vi "Main_Marvin Remake.vi"() -> ()   [LabVIEW 2017]
uses:
  PCAN_Driver/ControlCAN.llb/DevType.ctl
  PCAN_Driver/ControlCAN.llb/CAN Channel.ctl
  PCAN_Driver/ControlCAN.llb/VCI_INIT_CONFIG.ctl
  PCAN_Driver/ControlCAN.llb/InitFlag.ctl
  PCAN_Driver/ControlCAN.llb/Fliter.ctl
  PCAN_Driver/ControlCAN.llb/Mode.ctl
  <vilib>/Utility/miscctls.llb/LVRowAndColumnTypeDef.ctl
  <vilib>/Utility/cursorutil.llb/Set Cursor (Icon Pict).vi
  PCAN_Driver/ControlCAN.lvlib
panel:
  out "AO[1]Meas":dbl
  out "FullSpeed2 Speed":dbl
  out "FullSpeed2 Current":u32
  out "FullSpeed1 Current":u32
  out "FullSpeed1 Speed":dbl
  out "MaxBurnInTempVal":dbl
  in  "Stop Burn-in":bool
  out "VISA Tester":refnum<visa-resource-name>
  out "UUT":u8
  out "CAN Status":bool
  in  "Channel 2":T1 caption="Channel" items=["Channel 1", "Channel 2"]
  out "Config_CANAT":T7 {"DevType" items=["USB-CAN"=3, "USB-CAN2"=4]; "CanIndex" items=["通道1", "通道2"]; "VCI_INIT_CONFIG"."Fliter" items=["接收所有类型"=3, "只接收标准帧"=4, "只接收扩展帧"=7]; "VCI_INIT_CONFIG"."Mode" items=["正常工作", "自测模式（环回）", "仅侦听模式"]; "VCI_INIT_CONFIG"."InitFlag" items=["使用Flash参数", "使用界面设置参数"]}
  out "Array":u64[][](array[numeric]) format="%016x"
  out "Motor Phase Current RMS":dbl
  out "Ambient Temperature":dbl
  out "Speed error":bool
  out "Commutation err":bool
  out "Under voltage/Over voltage":bool
  out "Derated drive temp":bool
  out "Motor Over temperature":bool
  out "Motor Sensor temp Fauilre":bool
  out "Drive Over temperature":bool
  out "Drive Sensor temp Failure":bool
  out "Ambient Over temp":bool
  out "Ambient Sensor temp":bool
  out "DC Voltage":dbl
  out "DC Current":dbl
  out "Power transistor Heat sink Temp.":dbl
  out "Motor Stator Temp.":dbl
  out "Motor Speed RPM":dbl
  out "ECS State":u16
  out "UUT":string="EBAY"
  in  "Logger Path":path
  in  "Report":bool
  in  "Start":bool
  in  "ATR":string[][](table)=[["Test Communication", "-", "-", "-", "-", ""], ["Set S/N", "-", "-", "-", "-", ""], ["Set Board Number", "-", "-", "-", "-", ""], [" ", "", "", "", "", ""], ["Test Communication", "-", "-", "-", "-", ""], ["Get S/N", "-", "-", "-", "", ""], ["Get Board Number", "-", "-", "-", "", ""], ["Get FW", "-", "-", "-", "", ""], ["Enable Motor", "", "", "", "", ""], ["Small position command", "", "", "", "", ""], ["Measure delta", "", "", "", "", ""], ["Velocity command", "", "", "", "", ""]]
  in  "Settings":bool
  in  "Refresh Button":bool
  out "Status":bool
  in  "VISA Marvin":refnum<visa-resource-name>="COM6"
  in  "Serial Com":bool
  in  "Help Button":bool
  out "Pannel User Message":string
  in  "Stop Button":bool
  # "Marvin"
  # "REDLER TECHNOLOGIES LTD"
  # "ver 1.0"
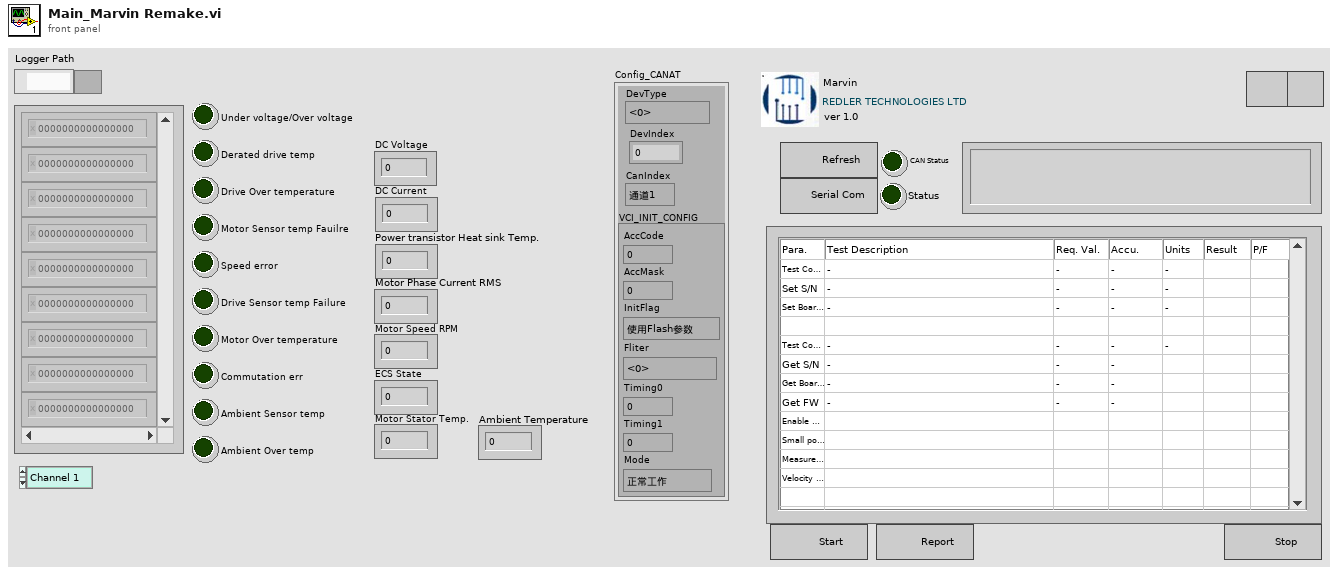
[diagram p1: front panel]
types:
  T1 = typedef "ControlCAN.lvlib/CAN Channel.ctl" = u32
  T2 = typedef "ControlCAN.lvlib/DevType.ctl" = u32
  T3 = typedef "ControlCAN.lvlib/VCI_INIT_CONFIG.ctl" = cluster{"AccCode":u32, "AccMask":u32, "InitFlag":T4, "Fliter":T5, "Timing0":u8, "Timing1":u8, "Mode":T6}
  T4 = typedef "ControlCAN.lvlib/InitFlag.ctl" = u32
  T5 = typedef "ControlCAN.lvlib/Fliter.ctl" = u8
  T6 = typedef "ControlCAN.lvlib/Mode.ctl" = u8
  T7 = cluster{"DevType":T2, "DevIndex":u32, "CanIndex":T1, "VCI_INIT_CONFIG":T3}
  T8 = cluster{"VISA":refnum<visa-resource-name>, "Array Test":enum16{"Auxiliary", "Temp Sens Cal", "Com Test", "Enable Test", "Speed Command", "Stop Time", "Temp Control", "Burn in", "Visual Inspec", "Empty"}[]}
  T9 = cluster{"ID":u32, "MSGTYPE":u8, "LEN":u8, "aDATA":u8[]}[]
  T10 = enum16{"Erase ATR Table", "Stop", "MainProgram", "Initialize"}
  T11 = enum16{"K15", "K16", "K17", "Venable", "Firmeware", "Fan", "Power", "120C", "110C", "100C", "90C", "80C", "70C", "60C", "50C", "40C", "30C", "25C", "20C", "10C", "0C"}
  T12 = enum16{"Stop", "Result", "FullSpeed2", "MD[1]=1", "FullSpeed1", "MD[1]=0"}
  T13 = enum8{"Term1", "Term2", "Current", "Fan", "TempCPU"}
  T14 = enum16{"Stop", "AO[1]=Meas.", "TA[5]", "AO[1]=0", "Start"}
  T15 = enum16{"Stop", "BurnIn", "Ambient Temp", "MotorSpeed", "DC Current Measure", "Start"}
  T16 = enum16{"Auxiliary", "Temp Sens Cal", "Com Test", "Enable Test", "Speed Command", "Stop Time", "Temp Control", "Burn in", "Visual Inspec", "Empty"}[]
  T17 = enum16{"K15", "K16", "K17", "Venable", "Firmeware", "Fan", "Power", "120C", "110C", "100C", "90C", "80C", "70C", "60C", "50C", "40C", "30C", "25C", "20C", "10C", "0C"}[]
  T18 = typedef "LVRowAndColumnTypeDef.ctl" = cluster{"Row":i32, "Column":i32}
  T19 = cluster{"ID":u32, "MSGTYPE":u8, "LEN":u8, "aDATA":u8[]}
  T20 = enum16{"Auxiliary", "Temp Sens Cal", "Com Test", "Enable Test", "Speed Command", "Stop Time", "Temp Control", "Burn in", "Visual Inspec", "Empty"}
  T21 = enum16{"open", "replace", "create", "open or create", "replace or create", "replace or create with confirmation"}
  T22 = enum32{"Invalid", "Standard", "Closed", "Hidden", "Minimized", "Maximized"}
  T23 = typedef "ControlCAN.lvlib/VCI_CAN_OBJ.ctl" = cluster{"ID":u32, "TimeStamp":u32, "TimeFlag":u8, "SendType":u8, "RemoteFlag":u8, "ExternFlag":u8, "DataLen":u8, "Data":u8[], "Reserved":u8[]}
  T24 = cluster{"Type":enum16{"接收", "发送"}, "Channel":T1, "Time":timestamp, "VCI_CAN_OBJ":T23}[]
  T25 = cluster{"Type":enum16{"接收", "发送"}, "Channel":T1, "Time":timestamp, "VCI_CAN_OBJ":T23}
  T26 = typedef "LVPoint32TypeDef.ctl" = cluster{"Horizontal":i32, "Vertical":i32}
  T27 = enum16{"Visual Inspection", "Temp Sens Cal", "Com Test", "Enable Test", "Speed Command", "Stop Time", "Temp Control", "Burn in", "Visual Inspec", "Empty"}[]
  T28 = enum16{"Auxiliary", "Temp Sens Cal", "Com Test", "Enable Test", "Speed Command", "Stop Time", "Burn in", "Visual Inspec", "Empty"}[]
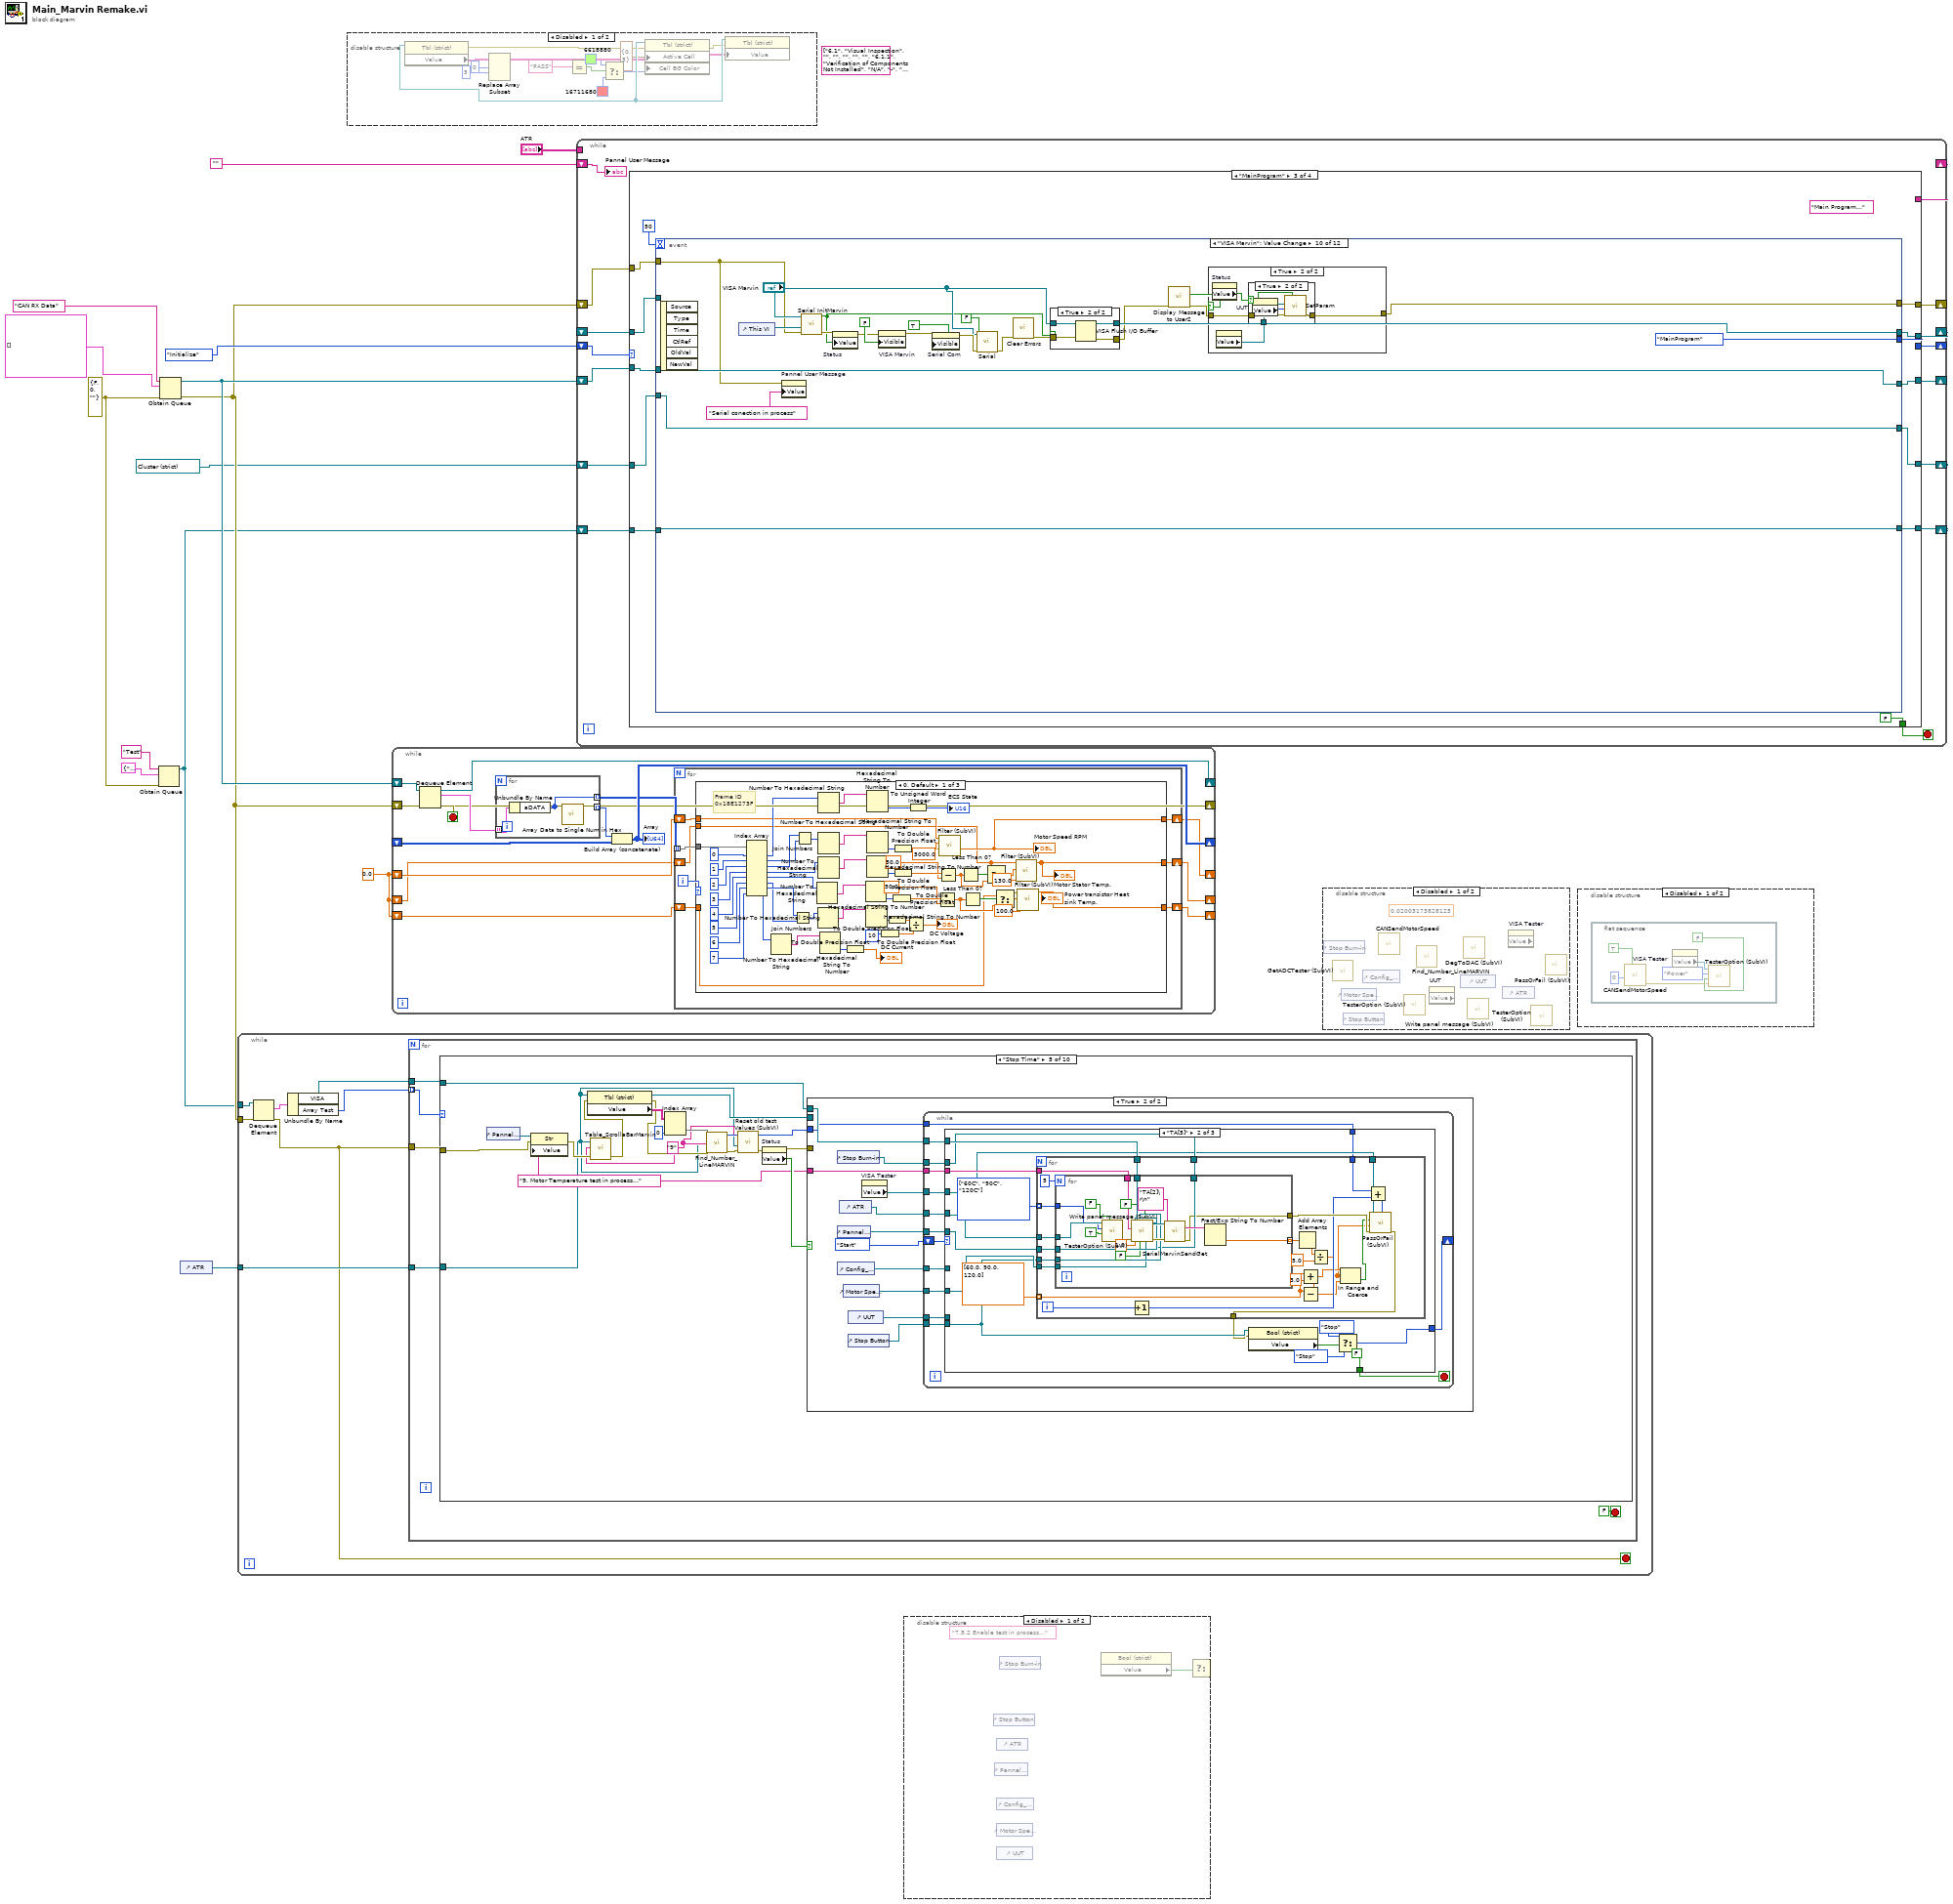
[diagram p0: block diagram]
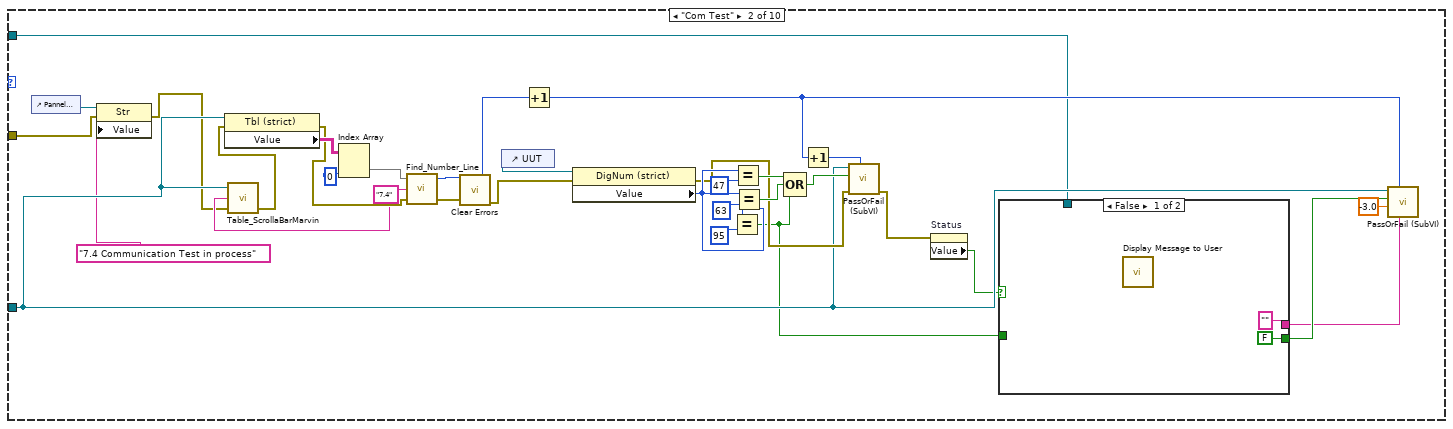
[diagram p6: hidden frame]
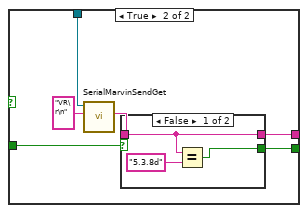
[diagram p7: hidden frame]
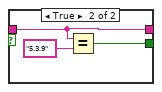
[diagram p8: hidden frame]
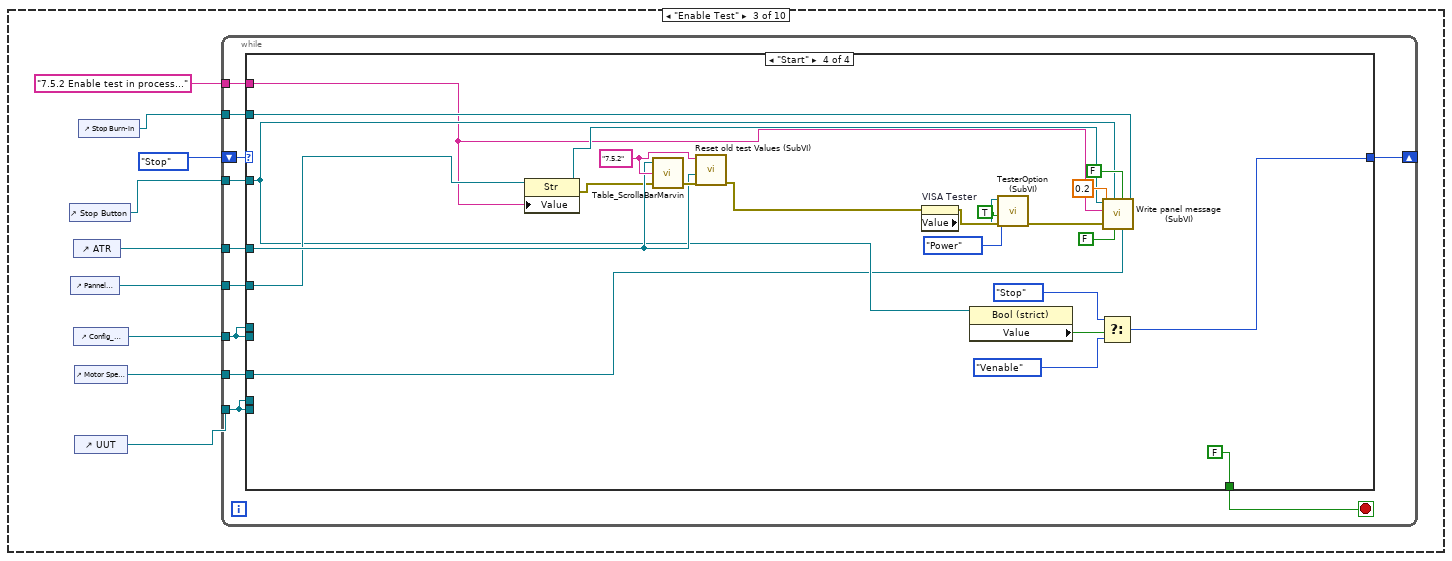
[diagram p9: hidden frame]
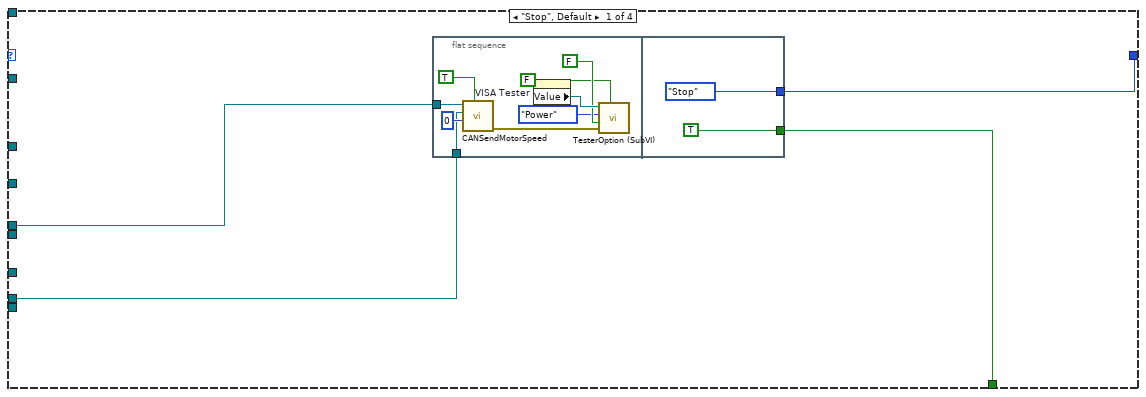
[diagram p10: hidden frame]
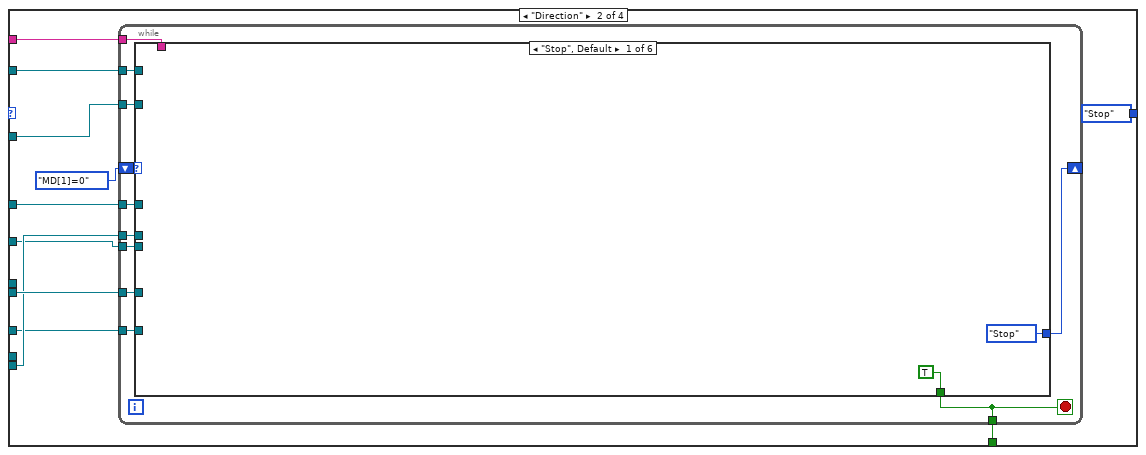
[diagram p11: hidden frame]
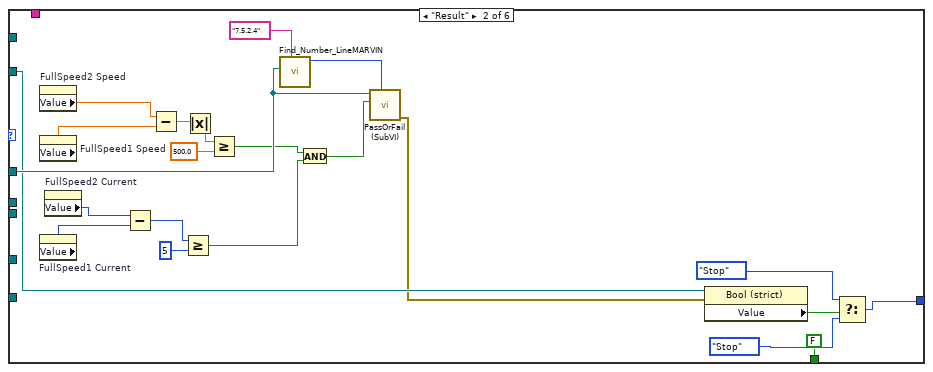
[diagram p12: hidden frame]
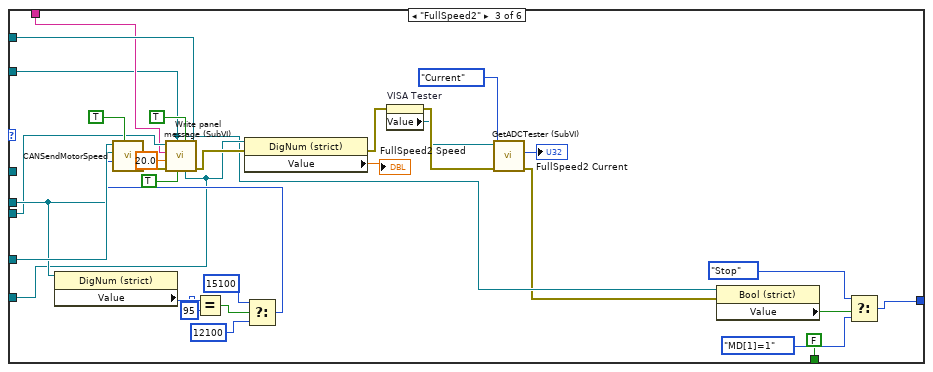
[diagram p13: hidden frame]
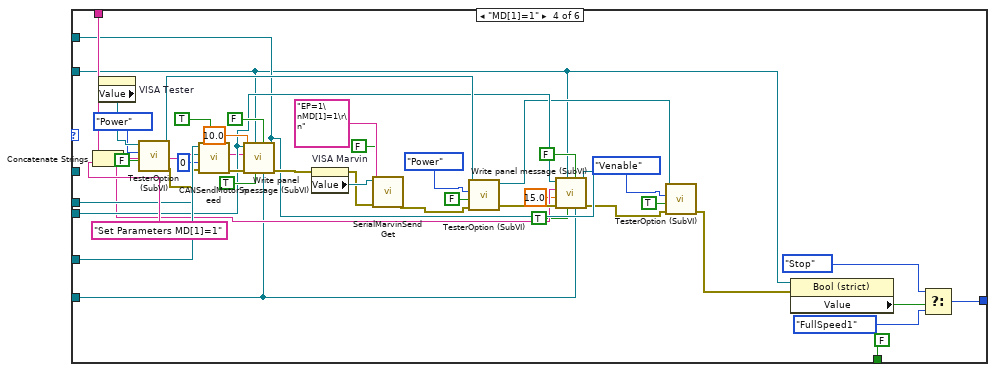
[diagram p14: hidden frame]
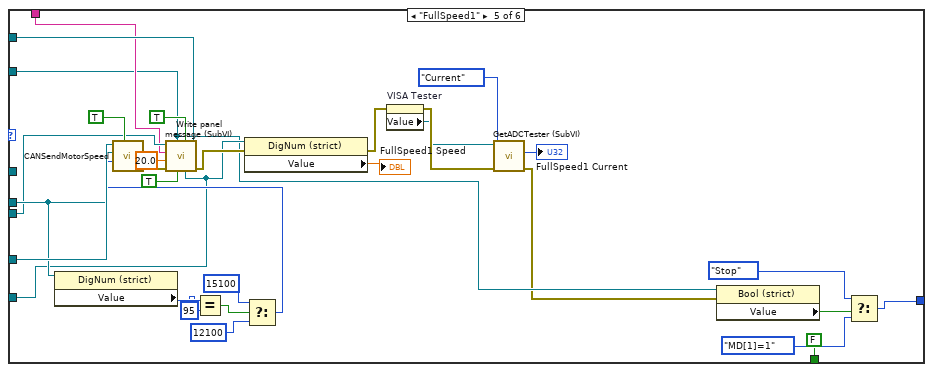
[diagram p15: hidden frame]
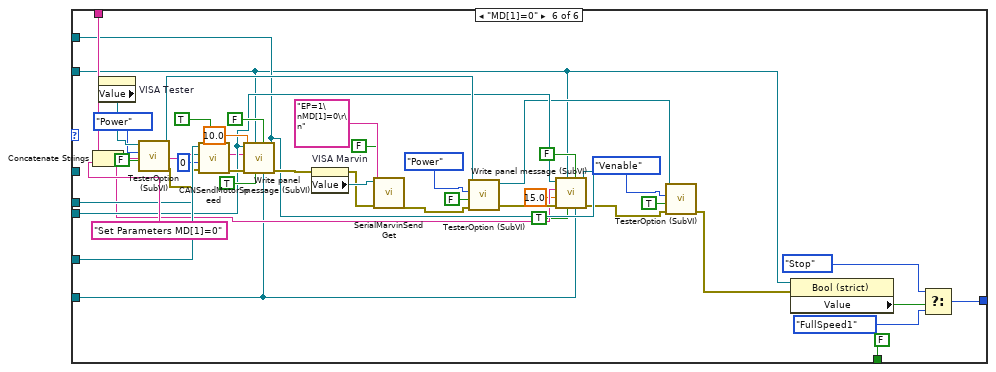
[diagram p16: hidden frame]
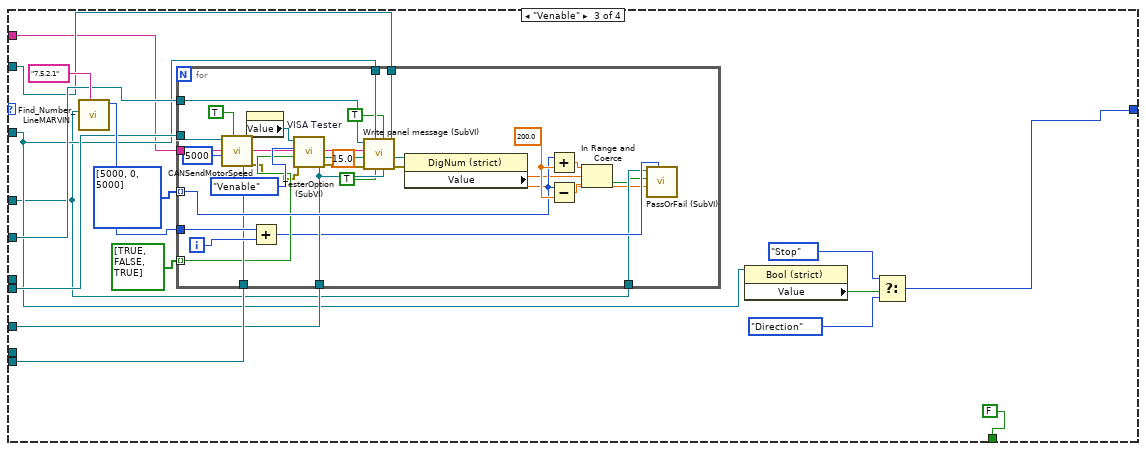
[diagram p17: hidden frame]
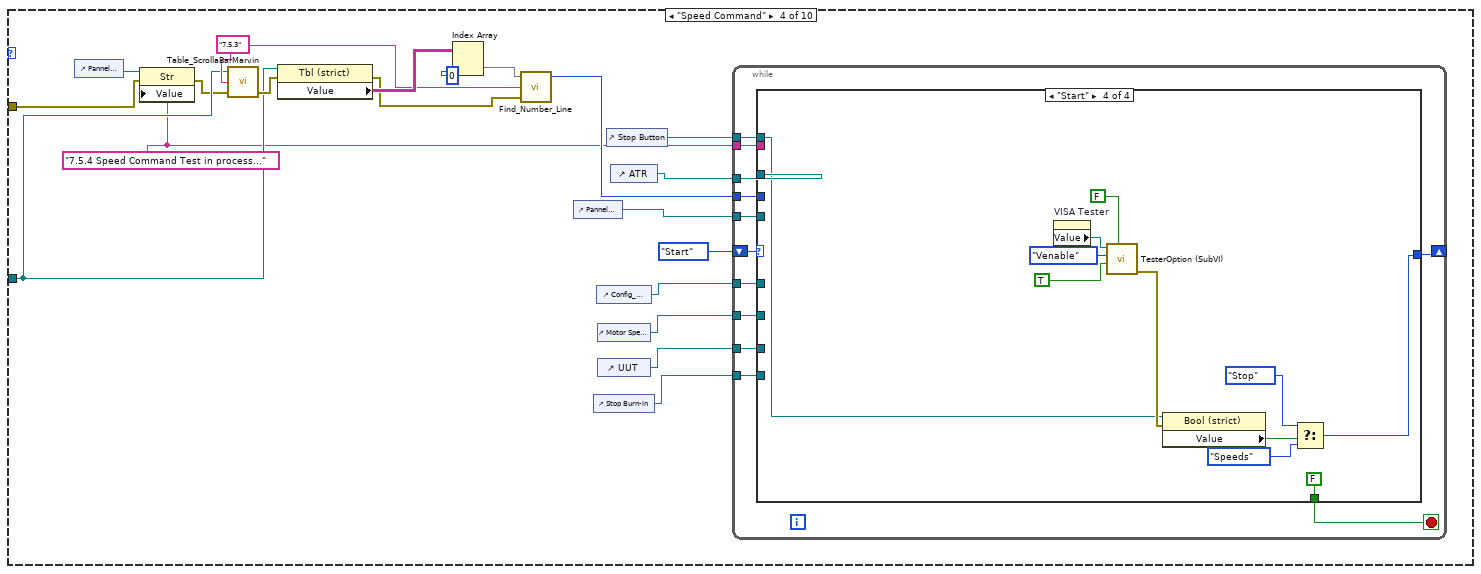
[diagram p18: hidden frame]
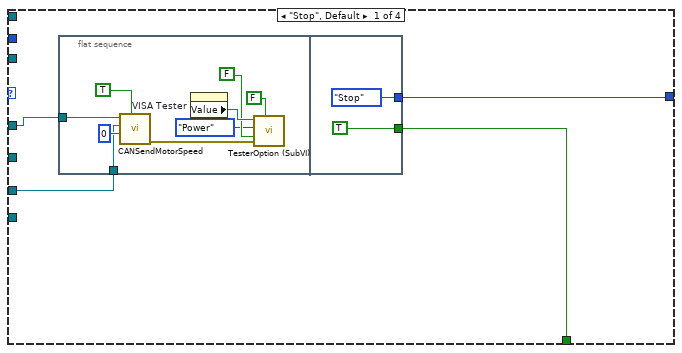
[diagram p19: hidden frame]
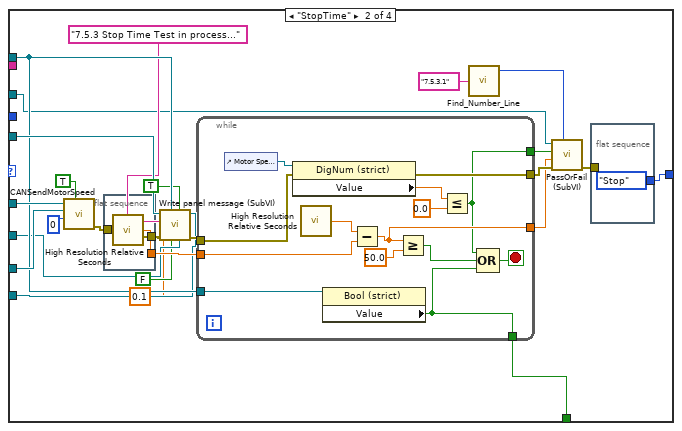
[diagram p20: hidden frame]
diagram:
  w1 = 0.0
  w8 = errorcluster {"status"=FALSE, "code"=0, "source"=""} ("error in (no error)")
  (unwired) string[][] [["6.1", "Visual Inspection", "", "", "", "", ""], ["6.1.1", "Verification of Components Not Installed", "N/A", "-", "", "", ""], ["", "", "", "", "", "", ""], ["6.1.2", "Manufacturing Defects", "N/A", "-", "", "", ""], ["", "", "", "", "", "", ""], ["6.2", "Power Supply Testing", "", "", "", "", ""], ["6.2.1", "Input Current Drawn", "", "", "", "", ""], ["6.2.1.1", "DC Input Current", "< 150", "-", "mA", "", ""], ["", "", "", "", "", "", ""], ["6.2.2", "Power Supply Voltages", "", "", "", "", ""], ["6.2.2.1", "12V", "12.0", "+/-0.500", "V", "", ""], ["6.2.2.2", "5V", "5.0", "+/-0.200", "V", "", ""], ["6.2.2.3", "3.3V", "3.3", "+/-0.100", "V", "", ""], ["6.2.2.4", "1.8V", "1.8", "+/-0.100", "V", "", ""], ["", "", "", "", "", "", ""], ["7", "Functional Test Procedure", "", "", "", "", ""], ["7.1", "Weight Check", "4180", "+/-10.00", "gr", "", ""], ["", "", "", "", "", "", ""], ["7.2", "Insulation Resistance Test", "", "", "", "", ""], ["7.2.1", "J3.B to Chassis", "> 1M", "-", "ohms", "", ""], ["7.2.2", "J1.16 to Chassis", "> 100K", "-", "ohms", "", ""], ["", "", "", "", "", "", ""], ["7.2", "Bonding Resistance", "", "", "", "", ""], ["7.2.3", "J1 Body to Chassis", "< 2m", "-", "ohms", "", ""], ["7.2.4", "J2  Body to Chassis", "< 2m", "-", "ohms", "", ""], ["7.2.5", "J3  Body to Chassis", "< 2m", "-", "ohms", "", ""], ["", "", "", "", "", "", ""], ["7.2.1", "CANbus Resistance Test", "", "", "", "", ""], ["7.2.1.1", "J1.17 to J1.18", "> 10K", "-", "ohms", "", ""], ["", "", "", "", "", "", ""], ["7.3", "Sealing Test", "N/A", "-", "", "", ""], ["", "", "", "", "", "", ""], ["7.4", "Communication Test", "", "", "", "", ""], ["7.4.1", "Serial RS-232", "N/A", "-", "", "", ""], ["7.4.2", "CAN Bus", "N/A", "-", "", "", ""], ["", "", "", "", "", "", ""], ["7.5", "Performances Tests", "", "", "", "", ""], ["7.5.1", "Reverse Polarity Test", "", "", "", "", ""], ["7.5.1.1", "DC Input Current", "< 1", "-", "mA", "", ""], ["", "", "", "", "", "", ""], ["7.5.2", "Enable Test", "", "", "", "", ""], ["7.5.2.1", "Fan Speed at Opened Enable ", "0", "-", "rpm", "", ""], ["7.5.2.2", "Fan Speed at Closed Enable ", "6000", "+/-200.0", "rpm", "", ""], ["7.5.2.3", "Motor Rotation Direction", "Counter-clockwise (Inlet)", "-", "", "", ""], ["", "", "", "", "", "", ""], ["7.5.3", "Stop Time Test ", "", "", "", "", ""], ["7.5.3.1", "Motor Stop time", "< 50", "-", "sec", "", ""], ["", "", "", "", "", "", ""], ["7.5.4", "Speed Command Test", "", "", "", "", ""], ["7.5.4.1", "Fan Speed", "6000", "+/-200.0", "rpm", "", ""], ["7.5.4.2", "Fan Speed", "11500", "+/-200.0", "rpm", "", ""], ["7.5.4.3", "Fan Speed", "15100", "+/-200.0", "rpm", "", ""], ["", "", "", "", "", "", ""], ["7.5.5", "Temperature Sensor Calibration Test", "", "", "", "", ""], ["7.5.5.1", "Sensor Reading Analog Offset", "0", "+/-0.100", ".", "", ""], ["", "", "", "", "", "", ""], ["7.5.6", "Temperature Control Algorithm Test", "", "", "", "", ""], ["7.5.6.1", "Tair <   68 ± 2 oC", "6000", "+/-200.0", "rpm", "", ""], ["7.5.6.2", "Tair >= 68 ± 2 oC", "11500", "+/-200.0", "rpm", "", ""], ["7.5.6.3", "Tair >= 88 ± 2 oC", "15100", "+/-400.0", "rpm", "", ""], ["7.5.6.4", "Tair <= 80 ± 2 oC", "11500", "+/-200.0", "rpm", "", ""], ["7.5.6.5", "Tair <= 60 ± 2 oC", "6000", "+/-200.0", "rpm", "", ""], ["", "", "", "", "", "", ""], ["7.5.7", "Burn-in Test", "", "", "", "", ""], ["7.5.7.1", "DC Input Current", "50", "+/-5.000", "A", "", ""], ["7.5.7.2", "Ambient Temperature", "25", "+/-13.00", "Deg.", "", ""], ["7.5.7.3", "After 10 min of operation", "", "", "Deg.", "", ""], ["7.5.7.4", "After 20 min of operation", "", "", "Deg.", "", ""], ["7.5.7.5", "After 30 min of operation", "", "", "Deg.", "", ""], ["7.5.7.6", "Auxiliary Cooling Fan 60 Deg", "On", "-", ".", "", ""], ["7.5.7.7", "Auxiliary Cooling Fan 55 Deg", "Off", "-", ".", "", ""]] ("data")
  n1 = Obtain Queue(name (unnamed)="Test", element data type=T8 {"VISA"="COM1", "Array Test"=[]}, error in (no error)=w8) -> (queue out=w5:refnum<queue>)  [unwired: 2 in, 2 out]
  n2 = Obtain Queue(name (unnamed)="CAN RX Data", element data type=T9 [], error in (no error)=w8) -> (queue out=w10:refnum<queue>, error out=w6:errorcluster)  [unwired: 2 in, 1 out]
  n3 = control-ref of="ATR"() -> (w7:refnum<vi>)
  n4 = while {
    tunnel: w7 -> [w21]
    tunnel: w6 -> [w19]
    tunnel: w5 -> [w20]
    stop <- w15 stop-if-true
    n5 = Dequeue Element(queue=w20, error in (no error)=w19) -> (element=w18:T8, error out=w15:errorcluster)  [unwired: 1 in, 2 out]
    n6 = Unbundle By Name(w18) -> ("VISA"=w17:refnum<visa-resource-name>, "Array Test"=w16:T16)
    n7 = for {
      tunnel: w16 -> [w22] mode=indexing
      tunnel: w17 -> [w26]
      tunnel: w21 -> [w25]
      tunnel: w15 -> [w24]
      stop <- FALSE stop-if-true
      n8 = case shown="\"Stop Time\"" w22 {
        tunnel: w26 -> [_ w33 _ _ w514 _ _ _ w1006 _]
        tunnel: w25 -> [_ w41 _ w382 w510 w672 _ w1003 w1014 w1226]
        tunnel: w24 -> [_ w37 _ w380 w520 w668 _ w1004 w1012 w1225]
        frame "Empty", Default {
        }
        frame "Com Test" {
          w40 = "7.4" ("Test Paragraph")
          n9 = control-ref of="Pannel User Message"() -> (w38:refnum<vi>)
          n10 = property class="Str"(reference=w38, error in=w37, "Value"="7.4 Communication Test in process") -> (error out=w36:errorcluster)  [unwired: 1 out]
          n11 = call "Table_ScrollaBarMarvin.vi"("error in"=w36, "Line to focus"=w40, "reference in"=w41) -> ("error out"=w39:errorcluster)  [unwired: 2 out]
          n12 = property class="Tbl (strict)"(reference=w41, error in=w39) -> (error out=w56:errorcluster, "Value"=w57:string[][])  [unwired: 1 out]
          n13 = Index Array(array=w57, index (col)=0 ("disabled index (col)")) -> (element=w58:string[])  [unwired: 1 in]
          n14 = call "Find_Number_Line.vi"("error in"=w56, "Test Paragraph"=w40, "Row Headers[]"=w58) -> ("error out"=w54:errorcluster, "Line number"=w53:i32)  [unwired: 1 out]
          n15 = call <vilib>:"Clear Errors.vi"("error in (no error)"=w54) -> ("error out"=w32:errorcluster)  [unwired: 5 in, 1 out]
          n16 = control-ref of="UUT"() -> (w52:refnum<vi>)
          n17 = Increment(x=w53) -> (x+1=w45:i32)
          n18 = property class="DigNum (strict)"(reference=w52, error in=w32) -> (error out=w42:errorcluster, "Value"=w51:u8)  [unwired: 1 out]
          n19 = Equal?(x=w51, y=u8 95) -> (x = y?=w30:bool)
          n20 = Equal?(x=w51, y=u8 47) -> (x = y?=w47:bool)
          n21 = Equal?(x=w51, y=u8 63) -> (x = y?=w46:bool)
          n22 = Compound Arithmetic op=OR(w47, w46, w30) -> (w43:bool)
          n23 = Increment(x=w45) -> (x+1=w44:i32)
          n24 = call "PassOrFail (SubVI).vi"("index (row)"=w44, "error in (no error)"=w42, "Pass?Fail"=w43, "Table in"=w41) -> ("error out"=w31:errorcluster)  [unwired: 7 in]
          n25 = property on="Status" class="Bool (strict)"(error in=w31) -> ("Value"=w34:bool)  [unwired: 1 in, 2 out]
          n26 = case shown="False" w34 {
            tunnel: w33 -> [_ w66]
            tunnel: w30 -> [_ w64]
            tunnel: [FALSE w62] -> w29
            tunnel: ["" ("read buffer") w61] -> w28
            frame False {
              n27 = call "Display Message to User"() -> ()  [unwired: 10 in, 2 out]
            }
            frame True {
              n28 = call "SerialMarvinSendGet.vi"("write buffer"="VR\r\n", "VISA resource name"=w66) -> ("read buffer"=w63:string)  [unwired: 8 in, 1 out]
              n29 = case shown="False" w64 {
                tunnel: w63 -> [w67 w70]
                tunnel: [w68 w71] -> w62
                tunnel: [w67 w70] -> w61
                frame False {
                  n30 = Equal?(x=w67, y="5.3.8d") -> (x = y?=w68:bool)
                }
                frame True {
                  n31 = Equal?(x=w70, y="5.3.9") -> (x = y?=w71:bool)
                }
              }
            }
          }
          n32 = call "PassOrFail (SubVI).vi"("String Res"=w28, "index (row)"=w45, "Data in"=-3.0, "Pass?Fail"=w29, "Table in"=w41) -> ()  [unwired: 6 in, 1 out]
        }
        frame "Enable Test" {
          n33 = control-ref of="Stop Button"() -> (w75:refnum<vi>)
          n34 = control-ref of="Pannel User Message"() -> (w77:refnum<vi>)
          n35 = control-ref of="ATR"() -> (w76:refnum<vi>)
          n36 = control-ref of="Config_CANAT"() -> (w78:refnum<vi>)
          n37 = control-ref of="Motor Speed RPM"() -> (w79:refnum<vi>)
          n38 = control-ref of="UUT"() -> (w80:refnum<vi>)
          n39 = control-ref of="Stop Burn-in"() -> (w81:refnum<vi>)
          n40 = while {
            shift-right: [w86] -> _
            shift-left: enum16{"Stop", "Direction", "Venable", "Start"}."Stop" -> [w92]
            tunnel: w75 -> [w91]
            tunnel: w76 -> [w90]
            tunnel: w77 -> [w89]
            tunnel: w78 -> [w82]
            tunnel: w79 -> [w88]
            tunnel: w80 -> [w83]
            tunnel: w81 -> [w85]
            tunnel: "7.5.2 Enable test in process..." ("Strin") -> [w84]
            stop <- w87 stop-if-true
            n41 = case shown="\"Start\"" w92 {
              tunnel: w91 -> [_ w114 w303 w348]
              tunnel: w90 -> [_ w109 w301 w355]
              tunnel: w89 -> [_ w112 w305 w354]
              tunnel: w82 -> [_ w116 w308 _]
              tunnel: w88 -> [_ w111 w306 w346]
              tunnel: w83 -> [_ w115 w307 _]
              tunnel: [w96 w117 FALSE FALSE] -> w87
              tunnel: [w93 enum16{"Stop", "Direction", "Venable", "Start"}."Stop" w302 w352] -> w86
              tunnel: w85 -> [_ w113 w304 w347]
              tunnel: w84 -> [_ w110 w300 w345]
              tunnel: w83 -> [w95 _ _ _]
              tunnel: w82 -> [w94 _ _ _]
              frame "Stop", Default {
                n42 = flat-sequence {
                  tunnel: w95 -> [w101]
                  tunnel: w94 -> [w100]
                  tunnel: [TRUE] -> w96
                  tunnel: [enum16{"Stop", "Direction", "Venable", "Start"}."Stop"] -> w93
                  frame #0 {
                    n43 = call "CANSendMotorSpeed.vi"("Remote"=TRUE, "Motor Speed RPM"=u16 0, "UUT"=w101, "CAN Cluster in"=w100) -> ("error out"=w104:errorcluster)  [unwired: 7 in]
                    n44 = property on="VISA Tester" class="VISAName"() -> ("Value"=w105:refnum<visa-resource-name>)  [unwired: 2 in, 2 out]
                    n45 = call "TesterOption (SubVI).vi"("2 Options"=FALSE, "error in (no error)"=w104, "On/Off"=FALSE, "Tester Option"=T11."Power", "VISA Refnum in"=w105) -> ()  [unwired: 5 in, 2 out]
                  }
                  frame #1 {
                  }
                }
              }
              frame "Direction" {
                n46 = while {
                  shift-right: [w128] -> _
                  shift-left: T12."MD[1]=0" -> [w129]
                  tunnel: [w127] -> w117
                  tunnel: w116 -> [w126]
                  tunnel: w115 -> [w125]
                  tunnel: w114 -> [w124]
                  tunnel: w113 -> [w123]
                  tunnel: w112 -> [w122]
                  tunnel: w111 -> [w121]
                  tunnel: w110 -> [w120]
                  tunnel: w109 -> [w119]
                  stop <- w127 stop-if-true
                  n47 = case shown="\"Stop\", Default" w129 {
                    tunnel: [T12."Stop" w150 w181 w225 w254 w298] -> w128
                    tunnel: [TRUE FALSE FALSE FALSE FALSE FALSE] -> w127
                    tunnel: w126 -> [_ _ w179 w218 w252 w291]
                    tunnel: w125 -> [_ _ w173 w196 w246 w269]
                    tunnel: w124 -> [_ w133 w155 w186 w228 w259]
                    tunnel: w123 -> [_ _ w167 w197 w240 w270]
                    tunnel: w122 -> [_ _ w168 w198 w241 w271]
                    tunnel: w121 -> [_ _ w165 w192 w238 w265]
                    tunnel: w120 -> [_ _ w162 w206 w235 w279]
                    tunnel: w119 -> [_ w138 _ _ _ _]
                    frame "Stop", Default {
                    }
                    frame "Result" {
                      n48 = property on="FullSpeed2 Speed" class="DigNum (strict)"() -> ("Value"=w147:dbl)  [unwired: 2 in, 2 out]
                      n49 = property on="FullSpeed1 Speed" class="DigNum (strict)"() -> ("Value"=w146:dbl)  [unwired: 2 in, 2 out]
                      n50 = property on="FullSpeed1 Current" class="DigNum (strict)"() -> ("Value"=w143:u32)  [unwired: 2 in, 2 out]
                      n51 = property on="FullSpeed2 Current" class="DigNum (strict)"() -> ("Value"=w144:u32)  [unwired: 2 in, 2 out]
                      n52 = Subtract(x=w144, y=w143) -> (x-y=w142:u32)
                      n53 = Subtract(x=w147, y=w146) -> (x-y=w148:dbl)
                      n54 = Greater Or Equal?(x=w142, y=u32 5) -> (x >= y?=w136:bool)
                      n55 = Absolute Value(x=w148) -> (abs(x)=w145:dbl)
                      n56 = Greater Or Equal?(x=w145, y=500.0) -> (x >= y?=w137:bool)
                      n57 = call "Find_Number_LineMARVIN.vi"("Test Paragraph"="7.5.2.4", "TableIn"=w138) -> ("Line number"=w134:i32)  [unwired: 3 in, 3 out]
                      n58 = And(x=w137, y=w136) -> (x .and. y?=w135:bool)
                      n59 = call "PassOrFail (SubVI).vi"("index (row)"=w134, "Pass?Fail"=w135, "Table in"=w138) -> ("error out"=w132:errorcluster)  [unwired: 8 in]
                      n60 = property class="Bool (strict)"(reference=w133, error in=w132) -> ("Value"=w153:bool)  [unwired: 2 out]
                      n61 = Select(t=T12."Stop", s=w153, f=T12."Stop") -> (s? t:f=w150:T12)
                    }
                    frame "FullSpeed2" {
                      n62 = property class="DigNum (strict)"(reference=w173) -> ("Value"=w178:u8)  [unwired: 1 in, 2 out]
                      n63 = Equal?(x=w178, y=u8 95) -> (x = y?=w177:bool)
                      n64 = Select(t=u16 15100, s=w177, f=u16 12100 ("y")) -> (s? t:f=w172:u16)
                      n65 = call "CANSendMotorSpeed.vi"("Remote"=TRUE, "Motor Speed RPM"=w172, "UUT"=w173, "CAN Cluster in"=w179) -> ("error out"=w170:errorcluster)  [unwired: 7 in]
                      n66 = call "Write panel message (SubVI).vi"("Stop BurnIn"=w167, 4:"rpm"=w165, 5:"rpm"=TRUE ("rpm"), "PrintTime"=TRUE, "Stop"=w155, "error in (no error)"=w170, "Time to wait"=20.0, "Strin"=w162, "String in"=w168) -> ("error out"=w169:errorcluster)  [unwired: 2 in]
                      n67 = property class="DigNum (strict)"(reference=w165, error in=w169) -> (error out=w161:errorcluster, "Value"=→"FullSpeed2 Speed":dbl)  [unwired: 1 out]
                      n68 = property on="VISA Tester" class="VISAName"(error in=w161) -> (error out=w160:errorcluster, "Value"=w159:refnum<visa-resource-name>)  [unwired: 1 in, 1 out]
                      n69 = call "GetADCTester (SubVI).vi"("error in (no error)"=w160, "GetADCTester"=T13."Current", "VISA Refnum in"=w159) -> ("error out"=w154:errorcluster, "ADCValOutput Single"=→"FullSpeed2 Current":u32)  [unwired: 6 in, 1 out]
                      n70 = property class="Bool (strict)"(reference=w155, error in=w154) -> ("Value"=w184:bool)  [unwired: 2 out]
                      n71 = Select(t=T12."Stop", s=w184, f=T12."MD[1]=1") -> (s? t:f=w181:T12)
                    }
                    frame "MD[1]=1" {
                      n72 = Concatenate Strings(w206, "Set Parameters MD[1]=1" ("Strin")) -> (w195:string)
                      n73 = property on="VISA Tester" class="VISAName"() -> ("Value"=w212:refnum<visa-resource-name>)  [unwired: 2 in, 2 out]
                      n74 = call "TesterOption (SubVI).vi"("On/Off"=FALSE, "Tester Option"=T11."Power", "VISA Refnum in"=w212) -> ("error out"=w213:errorcluster, "VISA Refnum out"=w202:refnum<visa-resource-name>)  [unwired: 7 in]
                      n75 = call "CANSendMotorSpeed.vi"("Remote"=TRUE, "error in (no error)"=w213, "Motor Speed RPM"=u16 0, "UUT"=w196, "CAN Cluster in"=w218) -> ("error out"=w215:errorcluster)  [unwired: 6 in]
                      n76 = call "Write panel message (SubVI).vi"("Stop BurnIn"=w197, 4:"rpm"=w192, 5:"rpm"=FALSE ("rpm"), "PrintTime"=TRUE, "Stop"=w186, "error in (no error)"=w215, "Time to wait"=10.0, "Strin"=w195, "String in"=w198) -> ("error out"=w209:errorcluster)  [unwired: 2 in]
                      n77 = property on="VISA Marvin" class="VISAName"(error in=w209) -> (error out=w214:errorcluster, "Value"=w221:refnum<visa-resource-name>)  [unwired: 1 in, 1 out]
                      n78 = call "SerialMarvinSendGet.vi"("error in (no error)"=w214, "Clear Log"=FALSE, "write buffer"="EP=1\nMD[1]=1\r\n", "VISA resource name"=w221) -> ("error out"=w201:errorcluster)  [unwired: 6 in, 1 out]
                      n79 = call "TesterOption (SubVI).vi"("error in (no error)"=w201, "On/Off"=FALSE, "Tester Option"=T11."Power", "VISA Refnum in"=w202) -> ("error out"=w199:errorcluster, "VISA Refnum out"=w187:refnum<visa-resource-name>)  [unwired: 6 in]
                      n80 = call "Write panel message (SubVI).vi"("Stop BurnIn"=w197, 4:"rpm"=w192, 5:"rpm"=FALSE ("rpm"), "PrintTime"=TRUE, "Stop"=w186, "error in (no error)"=w199, "Time to wait"=15.0, "Strin"=w195, "String in"=w198) -> ("error out"=w188:errorcluster)  [unwired: 2 in]
                      n81 = call "TesterOption (SubVI).vi"("error in (no error)"=w188, "On/Off"=TRUE, "Tester Option"=T11."Venable", "VISA Refnum in"=w187) -> ("error out"=w185:errorcluster)  [unwired: 6 in, 1 out]
                      n82 = property class="Bool (strict)"(reference=w186, error in=w185) -> ("Value"=w226:bool)  [unwired: 2 out]
                      n83 = Select(t=T12."Stop", s=w226, f=T12."FullSpeed1") -> (s? t:f=w225:T12)
                    }
                    frame "FullSpeed1" {
                      n84 = property class="DigNum (strict)"(reference=w246) -> ("Value"=w251:u8)  [unwired: 1 in, 2 out]
                      n85 = Equal?(x=w251, y=u8 95) -> (x = y?=w250:bool)
                      n86 = Select(t=u16 15100, s=w250, f=u16 12100 ("y")) -> (s? t:f=w245:u16)
                      n87 = call "CANSendMotorSpeed.vi"("Remote"=TRUE, "Motor Speed RPM"=w245, "UUT"=w246, "CAN Cluster in"=w252) -> ("error out"=w243:errorcluster)  [unwired: 7 in]
                      n88 = call "Write panel message (SubVI).vi"("Stop BurnIn"=w240, 4:"rpm"=w238, 5:"rpm"=TRUE ("rpm"), "PrintTime"=TRUE, "Stop"=w228, "error in (no error)"=w243, "Time to wait"=20.0, "Strin"=w235, "String in"=w241) -> ("error out"=w242:errorcluster)  [unwired: 2 in]
                      n89 = property class="DigNum (strict)"(reference=w238, error in=w242) -> (error out=w234:errorcluster, "Value"=→"FullSpeed1 Speed":dbl)  [unwired: 1 out]
                      n90 = property on="VISA Tester" class="VISAName"(error in=w234) -> (error out=w233:errorcluster, "Value"=w232:refnum<visa-resource-name>)  [unwired: 1 in, 1 out]
                      n91 = call "GetADCTester (SubVI).vi"("error in (no error)"=w233, "GetADCTester"=T13."Current", "VISA Refnum in"=w232) -> ("error out"=w227:errorcluster, "ADCValOutput Single"=→"FullSpeed1 Current":u32)  [unwired: 6 in, 1 out]
                      n92 = property class="Bool (strict)"(reference=w228, error in=w227) -> ("Value"=w257:bool)  [unwired: 2 out]
                      n93 = Select(t=T12."Stop", s=w257, f=T12."MD[1]=1") -> (s? t:f=w254:T12)
                    }
                    frame "MD[1]=0" {
                      n94 = Concatenate Strings(w279, "Set Parameters MD[1]=0" ("Strin")) -> (w268:string)
                      n95 = property on="VISA Tester" class="VISAName"() -> ("Value"=w285:refnum<visa-resource-name>)  [unwired: 2 in, 2 out]
                      n96 = call "TesterOption (SubVI).vi"("On/Off"=FALSE, "Tester Option"=T11."Power", "VISA Refnum in"=w285) -> ("error out"=w286:errorcluster, "VISA Refnum out"=w275:refnum<visa-resource-name>)  [unwired: 7 in]
                      n97 = call "CANSendMotorSpeed.vi"("Remote"=TRUE, "error in (no error)"=w286, "Motor Speed RPM"=u16 0, "UUT"=w269, "CAN Cluster in"=w291) -> ("error out"=w288:errorcluster)  [unwired: 6 in]
                      n98 = call "Write panel message (SubVI).vi"("Stop BurnIn"=w270, 4:"rpm"=w265, 5:"rpm"=FALSE ("rpm"), "PrintTime"=TRUE, "Stop"=w259, "error in (no error)"=w288, "Time to wait"=10.0, "Strin"=w268, "String in"=w271) -> ("error out"=w282:errorcluster)  [unwired: 2 in]
                      n99 = property on="VISA Marvin" class="VISAName"(error in=w282) -> (error out=w287:errorcluster, "Value"=w294:refnum<visa-resource-name>)  [unwired: 1 in, 1 out]
                      n100 = call "SerialMarvinSendGet.vi"("error in (no error)"=w287, "Clear Log"=FALSE, "write buffer"="EP=1\nMD[1]=0\r\n", "VISA resource name"=w294) -> ("error out"=w274:errorcluster)  [unwired: 6 in, 1 out]
                      n101 = call "TesterOption (SubVI).vi"("error in (no error)"=w274, "On/Off"=FALSE, "Tester Option"=T11."Power", "VISA Refnum in"=w275) -> ("error out"=w272:errorcluster, "VISA Refnum out"=w260:refnum<visa-resource-name>)  [unwired: 6 in]
                      n102 = call "Write panel message (SubVI).vi"("Stop BurnIn"=w270, 4:"rpm"=w265, 5:"rpm"=FALSE ("rpm"), "PrintTime"=TRUE, "Stop"=w259, "error in (no error)"=w272, "Time to wait"=15.0, "Strin"=w268, "String in"=w271) -> ("error out"=w261:errorcluster)  [unwired: 2 in]
                      n103 = call "TesterOption (SubVI).vi"("error in (no error)"=w261, "On/Off"=TRUE, "Tester Option"=T11."Venable", "VISA Refnum in"=w260) -> ("error out"=w258:errorcluster)  [unwired: 6 in, 1 out]
                      n104 = property class="Bool (strict)"(reference=w259, error in=w258) -> ("Value"=w299:bool)  [unwired: 2 out]
                      n105 = Select(t=T12."Stop", s=w299, f=T12."FullSpeed1") -> (s? t:f=w298:T12)
                    }
                  }
                }
              }
              frame "Venable" {
                n106 = call "Find_Number_LineMARVIN.vi"("Test Paragraph"="7.5.2.1", "TableIn"=w301) -> ("Line number"=w309:i32)  [unwired: 3 in, 3 out]
                n107 = for {
                  tunnel: u16[] [5000, 0, 5000] -> [w338] mode=indexing
                  tunnel: bool[] [TRUE, FALSE, TRUE] -> [w333] mode=indexing
                  tunnel: w309 -> [w339]
                  tunnel: w308 -> [w337]
                  tunnel: w307 -> [w336]
                  tunnel: w306 -> [w324]
                  tunnel: w305 -> [w328]
                  tunnel: w303 -> [w327]
                  tunnel: w304 -> [w326]
                  tunnel: w301 -> [w320]
                  tunnel: w300 -> [w317]
                  i -> [w340]
                  w342 = 200.0 ("y")
                  n108 = call "CANSendMotorSpeed.vi"("Remote"=TRUE, "Motor Speed RPM"=u16 5000, "UUT"=w336, "CAN Cluster in"=w337) -> ("error out"=w332:errorcluster)  [unwired: 7 in]
                  n109 = property on="VISA Tester" class="VISAName"() -> ("Value"=w331:refnum<visa-resource-name>)  [unwired: 2 in, 2 out]
                  n110 = Add(x=w339, y=w340) -> (x+y=w321:i32)
                  n111 = call "TesterOption (SubVI).vi"("error in (no error)"=w332, "On/Off"=w333, "Tester Option"=T11."Venable", "VISA Refnum in"=w331) -> ("error out"=w330:errorcluster)  [unwired: 6 in, 1 out]
                  n112 = call "Write panel message (SubVI).vi"("Stop BurnIn"=w326, 4:"rpm"=w324, 5:"rpm"=TRUE ("rpm"), "PrintTime"=TRUE, "Stop"=w327, "error in (no error)"=w330, "Time to wait"=15.0, "Strin"=w317, "String in"=w328) -> ("error out"=w329:errorcluster)  [unwired: 2 in]
                  n113 = property class="DigNum (strict)"(reference=w324, error in=w329) -> ("Value"=w318:dbl)  [unwired: 2 out]
                  n114 = Add(x=w338, y=w342) -> (x+y=w344:dbl)
                  n115 = Subtract(x=w338, y=w342) -> (x-y=w343:dbl)
                  n116 = In Range and Coerce(upper limit=w344, x=w318, lower limit=w343) -> (In Range?=w319:bool)  [unwired: 1 out]
                  n117 = call "PassOrFail (SubVI).vi"("index (row)"=w321, "Data in"=w318, "Pass?Fail"=w319, "Table in"=w320) -> ()  [unwired: 7 in, 1 out]
                }
                n118 = property class="Bool (strict)"(reference=w303) -> ("Value"=w316:bool)  [unwired: 1 in, 2 out]
                n119 = Select(t=enum16{"Stop", "Direction", "Venable", "Start"}."Stop", s=w316, f=enum16{"Stop", "Direction", "Venable", "Start"}."Direction") -> (s? t:f=w302:enum16{"Stop", "Direction", "Venable", "Start"})
              }
              frame "Start" {
                w363 = "7.5.2" ("Test Paragraph")
                n120 = property class="Str"(reference=w354, "Value"=w345) -> (reference out=w364:refnum<vi>, error out=w351:errorcluster)  [unwired: 1 in]
                n121 = call "Table_ScrollaBarMarvin.vi"("error in"=w351, "Line to focus"=w363, "reference in"=w355) -> ("error out"=w360:errorcluster)  [unwired: 2 out]
                n122 = call "Reset old test Values (SubVI).vi"("error in"=w360, "Atr in"=w355, "Test Paragraph"=w363) -> ("error out"=w359:errorcluster)  [unwired: 8 in]
                n123 = property on="VISA Tester" class="VISAName"(error in=w359) -> (error out=w358:errorcluster, "Value"=w357:refnum<visa-resource-name>)  [unwired: 1 in, 1 out]
                n124 = property class="Bool (strict)"(reference=w348) -> ("Value"=w368:bool)  [unwired: 1 in, 2 out]
                n125 = call "TesterOption (SubVI).vi"("error in (no error)"=w358, "On/Off"=TRUE, "Tester Option"=T11."Power", "VISA Refnum in"=w357) -> ("error out"=w356:errorcluster)  [unwired: 6 in, 1 out]
                n126 = Select(t=enum16{"Stop", "Direction", "Venable", "Start"}."Stop", s=w368, f=enum16{"Stop", "Direction", "Venable", "Start"}."Venable") -> (s? t:f=w352:enum16{"Stop", "Direction", "Venable", "Start"})
                n127 = call "Write panel message (SubVI).vi"("Stop BurnIn"=w347, 4:"rpm"=w346, 5:"rpm"=FALSE ("rpm"), "PrintTime"=FALSE, "Stop"=w348, "error in (no error)"=w356, "Time to wait"=0.2, "Strin"=w345, "String in"=w364) -> ()  [unwired: 2 in, 1 out]
              }
            }
          }
        }
        frame "Speed Command" {
          w369 = "7.5.4 Speed Command Test in process..." ("Value")
          w384 = "7.5.3" ("Test Paragraph")
          n128 = control-ref of="Pannel User Message"() -> (w381:refnum<vi>)
          n129 = property class="Str"(reference=w381, error in=w380, "Value"=w369) -> (error out=w379:errorcluster)  [unwired: 1 out]
          n130 = call "Table_ScrollaBarMarvin.vi"("error in"=w379, "Line to focus"=w384, "reference in"=w382) -> ("error out"=w383:errorcluster)  [unwired: 2 out]
          n131 = property class="Tbl (strict)"(reference=w382, error in=w383) -> (error out=w386:errorcluster, "Value"=w387:string[][])  [unwired: 1 out]
          n132 = Index Array(array=w387, index (col)=0 ("disabled index (col)")) -> (element=w388:string[])  [unwired: 1 in]
          n133 = call "Find_Number_Line.vi"("error in"=w386, "Test Paragraph"=w384, "Row Headers[]"=w388) -> ("Line number"=w370:i32)  [unwired: 2 out]
          n134 = control-ref of="Pannel User Message"() -> (w374:refnum<vi>)
          n135 = control-ref of="Stop Burn-in"() -> (w378:refnum<vi>)
          n136 = control-ref of="Config_CANAT"() -> (w375:refnum<vi>)
          n137 = control-ref of="Motor Speed RPM"() -> (w376:refnum<vi>)
          n138 = control-ref of="UUT"() -> (w377:refnum<vi>)
          n139 = control-ref of="Stop Button"() -> (w372:refnum<vi>)
          n140 = control-ref of="ATR"() -> (w373:refnum<vi>)
          n141 = while {
            shift-right: [w399] -> _
            shift-left: enum16{"Stop", "StopTime", "Speeds", "Start"}."Start" -> [w400]
            tunnel: w372 -> [w398]
            tunnel: w373 -> [w397]
            tunnel: w374 -> [w396]
            tunnel: w375 -> [w395]
            tunnel: w376 -> [w394]
            tunnel: w377 -> [w393]
            tunnel: w378 -> [w392]
            tunnel: w370 -> [w391]
            tunnel: w369 -> [w390]
            stop <- w389 stop-if-true
            n142 = case shown="\"Start\"" w400 {
              tunnel: [w404 w435 w459 w501] -> w399
              tunnel: w398 -> [_ w429 w464 w499]
              tunnel: w397 -> [_ w418 w469 _]
              tunnel: w396 -> [_ w430 w465 _]
              tunnel: w395 -> [w402 w433 w467 _]
              tunnel: w394 -> [_ w426 w462 _]
              tunnel: w393 -> [w403 w432 w468 _]
              tunnel: w392 -> [_ w427 w463 _]
              tunnel: w391 -> [_ _ w470 _]
              tunnel: w390 -> [_ _ w466 _]
              tunnel: [w401 w434 w461 FALSE ("Value")] -> w389
              frame "Stop", Default {
                n143 = flat-sequence {
                  tunnel: w403 -> [w407]
                  tunnel: w402 -> [w406]
                  tunnel: [enum16{"Stop", "StopTime", "Speeds", "Start"}."Stop"] -> w404
                  tunnel: [TRUE] -> w401
                  frame #0 {
                    n144 = call "CANSendMotorSpeed.vi"("Remote"=TRUE, "Motor Speed RPM"=u16 0, "UUT"=w407, "CAN Cluster in"=w406) -> ("error out"=w412:errorcluster)  [unwired: 7 in]
                    n145 = property on="VISA Tester" class="VISAName"() -> ("Value"=w413:refnum<visa-resource-name>)  [unwired: 2 in, 2 out]
                    n146 = call "TesterOption (SubVI).vi"("2 Options"=FALSE, "error in (no error)"=w412, "On/Off"=FALSE, "Tester Option"=T11."Power", "VISA Refnum in"=w413) -> ()  [unwired: 5 in, 2 out]
                  }
                  frame #1 {
                  }
                }
              }
              frame "StopTime" {
                n147 = call "CANSendMotorSpeed.vi"("Remote"=TRUE, "Motor Speed RPM"=u16 0, "UUT"=w432, "CAN Cluster in"=w433) -> ("error out"=w439:errorcluster)  [unwired: 7 in]
                n148 = flat-sequence {
                  tunnel: [w443] -> w438
                  tunnel: w439 -> [w442]
                  tunnel: [w442] -> w440
                  frame #0 {
                    n149 = call <vilib>:"High Resolution Relative Seconds.vi"() -> ("relative seconds"=w443:dbl)
                  }
                }
                n150 = call "Write panel message (SubVI).vi"("Stop BurnIn"=w427, 4:"rpm"=w426, 5:"rpm"=TRUE ("rpm"), "PrintTime"=FALSE, "Stop"=w429, "error in (no error)"=w440, "Time to wait"=0.1, "Strin"="7.5.3 Stop Time Test in process..." ("Value"), "String in"=w430) -> ("error out"=w431:errorcluster)  [unwired: 2 in]
                n151 = while {
                  tunnel: w438 -> [w453]
                  tunnel: w431 -> [w447]
                  tunnel: [w449] -> w416
                  tunnel: [w448] -> w422
                  tunnel: [w446] -> w434
                  tunnel: w429 -> [w445]
                  tunnel: [w444] -> w417
                  stop <- w451 stop-if-true
                  n152 = control-ref of="Motor Speed RPM"() -> (w457:refnum<vi>)
                  n153 = property class="DigNum (strict)"(reference=w457, error in=w447) -> (error out=w448:errorcluster, "Value"=w456:dbl)  [unwired: 1 out]
                  n154 = call <vilib>:"High Resolution Relative Seconds.vi"() -> ("relative seconds"=w454:dbl)
                  n155 = property class="Bool (strict)"(reference=w445) -> ("Value"=w446:bool)  [unwired: 1 in, 2 out]
                  n156 = Subtract(x=w454, y=w453) -> (x-y=w449:dbl)
                  n157 = Greater Or Equal?(x=w449, y=50.0) -> (x >= y?=w450:bool)
                  n158 = Less Or Equal?(x=w456, y=0.0) -> (x <= y?=w444:bool)
                  n159 = Compound Arithmetic op=OR(w444, w450, w446) -> (w451:bool)
                }
                n160 = call "Find_Number_Line.vi"("Test Paragraph"="7.5.3.1") -> ("Line number"=w419:i32)  [unwired: 2 in, 2 out]
                n161 = call "PassOrFail (SubVI).vi"("index (row)"=w419, "error in (no error)"=w422, "Data in"=w416, "Pass?Fail"=w417, "Table in"=w418) -> ("error out"=w421:errorcluster)  [unwired: 6 in]
                n162 = flat-sequence {
                  tunnel: [enum16{"Stop", "StopTime", "Speeds", "Start"}."Stop"] -> w435
                  tunnel: w421 -> [_]
                  frame #0 {
                  }
                }
              }
              frame "Speeds" {
                n163 = for {
                  tunnel: u16[] [6000, 11500, 15100] -> [w491] mode=indexing
                  tunnel: w470 -> [w484]
                  tunnel: w469 -> [w483]
                  tunnel: w468 -> [w482]
                  tunnel: w467 -> [w481]
                  tunnel: w466 -> [w480]
                  tunnel: w465 -> [w479]
                  tunnel: w464 -> [w478]
                  tunnel: w463 -> [w476]
                  tunnel: w462 -> [w474]
                  tunnel: [w472] -> w461
                  i -> [w490]
                  stop <- w472 stop-if-true
                  w492 = 200.0 ("y")
                  n164 = Increment(x=w490) -> (x+1=w489:i32)
                  n165 = Add(x=w484, y=w489) -> (x+y=w485:i32)
                  n166 = call "CANSendMotorSpeed.vi"("Remote"=TRUE, "Motor Speed RPM"=w491, "UUT"=w482, "CAN Cluster in"=w481) -> ("error out"=w497:errorcluster)  [unwired: 7 in]
                  n167 = control-ref of="Motor Speed RPM"() -> (w498:refnum<vi>)
                  n168 = call "Write panel message (SubVI).vi"("Stop BurnIn"=w476, 4:"rpm"=w474, 5:"rpm"=TRUE ("rpm"), "PrintTime"=TRUE, "Stop"=w478, "error in (no error)"=w497, "Time to wait"=10.0 ("Delay Time (sec)"), "Strin"=w480, "String in"=w479) -> ("error out"=w488:errorcluster)  [unwired: 2 in]
                  n169 = property class="DigNum (strict)"(reference=w498, error in=w488) -> (error out=w496:errorcluster, "Value"=w473:dbl)  [unwired: 1 out]
                  n170 = property class="Bool (strict)"(reference=w478) -> ("Value"=w472:bool)  [unwired: 1 in, 2 out]
                  n171 = Add(x=w491, y=w492) -> (x+y=w494:dbl)
                  n172 = Subtract(x=w491, y=w492) -> (x-y=w493:dbl)
                  n173 = In Range and Coerce(upper limit=w494, x=w473, lower limit=w493) -> (In Range?=w495:bool)  [unwired: 1 out]
                  n174 = call "PassOrFail (SubVI).vi"("index (row)"=w485, "error in (no error)"=w496, "Data in"=w473, "Pass?Fail"=w495, "Table in"=w483) -> ()  [unwired: 6 in, 1 out]
                }
                n175 = Select(t=enum16{"Stop", "StopTime", "Speeds", "Start"}."Stop", s=w461, f=enum16{"Stop", "StopTime", "Speeds", "Start"}."StopTime") -> (s? t:f=w459:enum16{"Stop", "StopTime", "Speeds", "Start"})
              }
              frame "Start" {
                n176 = property on="VISA Tester" class="VISAName"() -> ("Value"=w509:refnum<visa-resource-name>)  [unwired: 2 in, 2 out]
                n177 = call "TesterOption (SubVI).vi"("2 Options"=FALSE, "On/Off"=TRUE, "Tester Option"=T11."Venable", "VISA Refnum in"=w509) -> ("error out"=w500:errorcluster)  [unwired: 6 in, 1 out]
                n178 = property class="Bool (strict)"(reference=w499, error in=w500) -> ("Value"=w505:bool)  [unwired: 2 out]
                n179 = Select(t=enum16{"Stop", "StopTime", "Speeds", "Start"}."Stop", s=w505, f=enum16{"Stop", "StopTime", "Speeds", "Start"}."Speeds") -> (s? t:f=w501:enum16{"Stop", "StopTime", "Speeds", "Start"})
              }
            }
          }
        }
        frame "Stop Time" {
          w513 = "9. Motor Temperature test in process..." ("Value")
          w511 = "9" ("Test Paragraph")
          n180 = control-ref of="Pannel User Message"() -> (w521:refnum<vi>)
          n181 = property class="Str"(reference=w521, error in=w520, "Value"=w513) -> (error out=w519:errorcluster)  [unwired: 1 out]
          n182 = call "Table_ScrollaBarMarvin.vi"("error in"=w519, "Line to focus"=w511, "reference in"=w510) -> ("error out"=w523:errorcluster)  [unwired: 2 out]
          n183 = property class="Tbl (strict)"(reference=w510, error in=w523) -> (reference out=w516:refnum<vi>, error out=w525:errorcluster, "Value"=w526:string[][])
          n184 = Index Array(array=w526, index (col)=0 ("disabled index (col)")) -> (element=w527:string[])  [unwired: 1 in]
          n185 = call "Find_Number_LineMARVIN.vi"("Test Paragraph"=w511, "error in"=w525, "TableIn"=w510, "Row Headers[]"=w527) -> ("error out"=w522:errorcluster, "Line number"=w515:i32)  [unwired: 1 in, 2 out]
          n186 = call "Reset old test Values (SubVI).vi"("error in"=w522, "Atr in"=w510, "Test Paragraph"=w511) -> ("error out"=w512:errorcluster)  [unwired: 8 in]
          n187 = property on="Status" class="Bool (strict)"(error in=w512) -> (error out=w517:errorcluster, "Value"=w518:bool)  [unwired: 1 in, 1 out]
          n188 = case shown="True" w518 {
            selector: w518 -> [w531 _]
            tunnel: w517 -> [w533 _]
            tunnel: w516 -> [w530 _]
            tunnel: w515 -> [w529 w536]
            tunnel: w514 -> [_ w541]
            tunnel: w513 -> [_ w537]
            frame False {
              n189 = flat-sequence {
                tunnel: w533 -> [w534]
                tunnel: [w534] -> w532
                frame #0 {
                  n190 = One Button Dialog(message="Please establish RS connection.") -> ()  [unwired: 1 in, 1 out]
                }
              }
              n191 = Increment(x=w529) -> (x+1=w528:i32)
              n192 = call "PassOrFail (SubVI).vi"("index (row)"=w528, "error in (no error)"=w532, "Pass?Fail"=w531, "Table in"=w530) -> ()  [unwired: 7 in, 1 out]
            }
            frame True {
              n193 = control-ref of="Stop Burn-in"() -> (w543:refnum<vi>)
              n194 = control-ref of="Pannel User Message"() -> (w545:refnum<vi>)
              n195 = control-ref of="Config_CANAT"() -> (w539:refnum<vi>)
              n196 = control-ref of="ATR"() -> (w546:refnum<vi>)
              n197 = control-ref of="Motor Speed RPM"() -> (w547:refnum<vi>)
              n198 = control-ref of="UUT"() -> (w538:refnum<vi>)
              n199 = control-ref of="Stop Button"() -> (w544:refnum<vi>)
              n200 = property on="VISA Tester" class="VISAName"() -> ("Value"=w540:refnum<visa-resource-name>)  [unwired: 2 in, 2 out]
              n201 = while {
                shift-right: [w551] -> _
                shift-left: T14."Start" -> [w561]
                tunnel: w543 -> [w560]
                tunnel: w544 -> [w559]
                tunnel: w545 -> [w558]
                tunnel: w546 -> [w557]
                tunnel: w547 -> [w556]
                tunnel: w541 -> [w555]
                tunnel: w540 -> [w554]
                tunnel: w539 -> [w553]
                tunnel: w538 -> [w552]
                tunnel: w537 -> [w549]
                tunnel: w536 -> [w548]
                stop <- w550 stop-if-true
                n202 = case shown="\"TA[5]\"" w561 {
                  tunnel: w560 -> [_ w582 w641]
                  tunnel: w559 -> [_ w574 w643]
                  tunnel: w558 -> [_ w583 w645]
                  tunnel: w557 -> [_ w572 _]
                  tunnel: w556 -> [_ w581 w640]
                  tunnel: w555 -> [_ w586 _]
                  tunnel: w554 -> [w564 w585 w634]
                  tunnel: w553 -> [_ _ w651]
                  tunnel: w552 -> [_ _ w650]
                  tunnel: [w562 w575 w636] -> w551
                  tunnel: [w563 FALSE FALSE] -> w550
                  tunnel: w549 -> [_ w584 _]
                  tunnel: w548 -> [_ w571 _]
                  frame "Stop", Default {
                    n203 = flat-sequence {
                      tunnel: w564 -> [w565]
                      tunnel: [TRUE] -> w563
                      tunnel: [T14."Stop"] -> w562
                      frame #0 {
                        n204 = call "TesterOption (SubVI).vi"("2 Options"=FALSE, "On/Off"=FALSE, "Tester Option"=T11."Power", "VISA Refnum in"=w565) -> ()  [unwired: 6 in, 2 out]
                      }
                      frame #1 {
                      }
                    }
                  }
                  frame "TA[5]" {
                    w587 = T17 [enum."60C", enum."90C", enum."120C"] items=["K15", "K16", "K17", "Venable", "Firmeware", "Fan", "Power", "120C", "110C", "100C", "90C", "80C", "70C", "60C", "50C", "40C", "30C", "25C", "20C", "10C", "0C"]
                    n205 = for {
                      tunnel: w587 -> [w611] mode=indexing
                      tunnel: w586 -> [w610]
                      tunnel: w585 -> [w609]
                      tunnel: w584 -> [w608]
                      tunnel: w583 -> [w607]
                      tunnel: w574 -> [w606]
                      tunnel: w582 -> [w605]
                      tunnel: w581 -> [w604]
                      tunnel: dbl[] [60.0, 90.0, 120.0] -> [w594] mode=indexing
                      tunnel: [w593] -> w573
                      tunnel: w572 -> [w600]
                      tunnel: w571 -> [w599]
                      i -> [w597]
                      w592 = 3.0 ("y")
                      n206 = for {
                        N: 5 -> [_]
                        tunnel: w611 -> [w613]
                        tunnel: w610 -> [w629]
                        tunnel: w609 -> [w625]
                        tunnel: w608 -> [w623]
                        tunnel: w607 -> [w622]
                        tunnel: w606 -> [w621]
                        tunnel: w605 -> [w619]
                        tunnel: w604 -> [w616]
                        tunnel: [w615] -> w603 mode=indexing
                        tunnel: [w614] -> w601
                        n207 = call "TesterOption (SubVI).vi"("2 Options"=FALSE, "On/Off"=TRUE, "Tester Option"=w613, "VISA Refnum in"=w625) -> ("error out"=w626:errorcluster)  [unwired: 6 in, 1 out]
                        n208 = call "Write panel message (SubVI).vi"("Stop BurnIn"=w619, 4:"rpm"=w616, 5:"rpm"=FALSE ("rpm"), "PrintTime"=FALSE, "Stop"=w621, "error in (no error)"=w626, "Time to wait"=1.0, "Strin"=w623, "String in"=w622) -> ("error out"=w624:errorcluster)  [unwired: 2 in]
                        n209 = call "SerialMarvinSendGet.vi"("error in (no error)"=w624, "write buffer"="TA[2]\r\n", "VISA resource name"=w629) -> ("error out"=w614:errorcluster, "read buffer"=w627:string)  [unwired: 7 in]
                        n210 = Fract/Exp String To Number(string=w627) -> (number=w615:dbl)  [unwired: 3 in, 1 out]
                      }
                      n211 = Increment(x=w597) -> (x+1=w596:i32)
                      n212 = Add Array Elements(numeric array=w603) -> (sum=w602:dbl)
                      n213 = Add(x=w594, y=w592) -> (x+y=w591:dbl)
                      n214 = Subtract(x=w594, y=w592) -> (x-y=w590:dbl)
                      n215 = Divide(x=w602, y=5.0) -> (x/y=w588:dbl)
                      n216 = In Range and Coerce(upper limit=w591, x=w588, lower limit=w590) -> (In Range?=w589:bool)  [unwired: 1 out]
                      n217 = Add(x=w599, y=w596) -> (x+y=w598:i32)
                      n218 = call "PassOrFail (SubVI).vi"("index (row)"=w598, "error in (no error)"=w601, "Data in"=w588, "Pass?Fail"=w589, "Table in"=w600) -> ("error out"=w593:errorcluster)  [unwired: 6 in]
                    }
                    n219 = property class="Bool (strict)"(reference=w574, error in=w573) -> ("Value"=w579:bool)  [unwired: 2 out]
                    n220 = Select(t=T14."Stop", s=w579, f=T14."Stop") -> (s? t:f=w575:T14)
                  }
                  frame "Start" {
                    n221 = call "Write panel message (SubVI).vi"("Stop BurnIn"=w641, 4:"rpm"=w640, 5:"rpm"=FALSE ("rpm"), "PrintTime"=FALSE, "Stop"=w643, "Time to wait"=0.1, "Strin"="9. Motor Temperature test in process...\nInitialization state...", "String in"=w645) -> ("error out"=w646:errorcluster)  [unwired: 3 in]
                    n222 = call "TesterOption (SubVI).vi"("2 Options"=FALSE, "error in (no error)"=w646, "On/Off"=FALSE, "Tester Option"=T11."Venable", "VISA Refnum in"=w634) -> ("error out"=w648:errorcluster)  [unwired: 5 in, 1 out]
                    n223 = call "CANSendMotorSpeed.vi"("Remote"=TRUE, "error in (no error)"=w648, "Motor Speed RPM"=u16 0, "UUT"=w650, "CAN Cluster in"=w651) -> ("error out"=w633:errorcluster)  [unwired: 6 in]
                    n224 = property class="Bool (strict)"(reference=w643, error in=w633) -> ("Value"=w655:bool)  [unwired: 2 out]
                    n225 = Select(t=T14."Stop", s=w655, f=T14."TA[5]") -> (s? t:f=w636:T14)
                  }
                }
              }
            }
          }
        }
        frame "Temp Control" {
          w656 = "7.5.6 Temperature controle test in process..." ("Value")
          w670 = "7.5.6" ("Test Paragraph")
          n226 = control-ref of="Pannel User Message"() -> (w669:refnum<vi>)
          n227 = property class="Str"(reference=w669, error in=w668, "Value"=w656) -> (error out=w667:errorcluster)  [unwired: 1 out]
          n228 = call "Table_ScrollaBarMarvin.vi"("error in"=w667, "Line to focus"=w670, "reference in"=w672) -> ("error out"=w677:errorcluster)  [unwired: 2 out]
          n229 = property class="Tbl (strict)"(reference=w672, error in=w677) -> (reference out=w666:refnum<vi>, error out=w676:errorcluster, "Value"=w675:string[][])
          n230 = Index Array(array=w675, index (col)=0 ("disabled index (col)")) -> (element=w674:string[])  [unwired: 1 in]
          n231 = control-ref of="Pannel User Message"() -> (w661:refnum<vi>)
          n232 = control-ref of="Motor Speed RPM"() -> (w659:refnum<vi>)
          n233 = call "Find_Number_Line.vi"("error in"=w676, "Test Paragraph"=w670, "Row Headers[]"=w674) -> ("error out"=w671:errorcluster)  [unwired: 2 out]
          n234 = control-ref of="Stop Button"() -> (w663:refnum<vi>)
          n235 = control-ref of="ATR"() -> (w662:refnum<vi>)
          n236 = control-ref of="Config_CANAT"() -> (w660:refnum<vi>)
          n237 = control-ref of="UUT"() -> (w658:refnum<vi>)
          n238 = control-ref of="Stop Burn-in"() -> (w657:refnum<vi>)
          n239 = call "Table_ScrollaBarMarvin.vi"("error in"=w671, "Line to focus"=w670, "reference in"=w666) -> ("error out"=w665:errorcluster)  [unwired: 2 out]
          n240 = while {
            tunnel: w665 -> [w689]
            shift-right: [w687] -> _
            shift-left: enum16{"Stop", "Algorithm", "Start"}."Start" -> [w688]
            tunnel: w663 -> [w686]
            tunnel: w662 -> [w685]
            tunnel: w661 -> [w684]
            tunnel: w660 -> [w683]
            tunnel: w659 -> [w682]
            tunnel: w658 -> [w681]
            tunnel: w657 -> [w679]
            tunnel: w656 -> [w678]
            stop <- w680 stop-if-true
            n241 = case shown="\"Algorithm\"" w688 {
              tunnel: w689 -> [_ _ w790]
              tunnel: [w690 w717 w779] -> w687
              tunnel: w686 -> [_ w714 w783]
              tunnel: w685 -> [_ w710 _]
              tunnel: w684 -> [_ w715 _]
              tunnel: w683 -> [w693 _ _]
              tunnel: w682 -> [_ w711 _]
              tunnel: w681 -> [w692 _ _]
              tunnel: [w691 FALSE FALSE] -> w680
              tunnel: w679 -> [_ w713 _]
              tunnel: w678 -> [_ w712 _]
              frame "Stop", Default {
                n242 = flat-sequence {
                  tunnel: w693 -> [w698]
                  tunnel: w692 -> [w695]
                  tunnel: [TRUE] -> w691
                  tunnel: [enum16{"Stop", "Algorithm", "Start"}."Stop"] -> w690
                  frame #0 {
                    n243 = property on="VISA Tester" class="VISAName"() -> ("Value"=w702:refnum<visa-resource-name>)  [unwired: 2 in, 2 out]
                    n244 = call "TesterOption (SubVI).vi"("2 Options"=FALSE, "On/Off"=FALSE, "Tester Option"=T11."Power", "VISA Refnum in"=w702) -> ("error out"=w696:errorcluster)  [unwired: 6 in, 1 out]
                    n245 = call "CANSendMotorSpeed.vi"("Remote"=TRUE, "error in (no error)"=w696, "Motor Speed RPM"=u16 0, "UUT"=w695, "CAN Cluster in"=w698) -> ()  [unwired: 6 in, 1 out]
                  }
                  frame #1 {
                  }
                  frame #2 {
                  }
                }
              }
              frame "Algorithm" {
                # "Speed Goal"
                # "Speed Ind"
                # "Temp Goal"
                # "60 Deg"
                n246 = for {
                  tunnel: [w733] -> w717
                  tunnel: w715 -> [w732]
                  tunnel: w714 -> [w731]
                  tunnel: w713 -> [w730]
                  tunnel: w712 -> [w729]
                  tunnel: w711 -> [w728]
                  tunnel: w710 -> [w727]
                  tunnel: string[] ["7.5.6.1", "7.5.6.3", "7.5.6.5", "7.5.6.7", "7.5.6.9"] -> [w725] mode=indexing
                  shift-right: [w723] -> _
                  shift-left: 1288.0 ("Rt") -> [w724]
                  tunnel: dbl[] [68.0, 68.0, 88.0, 80.0, 60.0] -> [w721] mode=indexing
                  tunnel: dbl[] [6000.0, 11500.0, 15100.0, 11500.0, 6000.0] -> [w720] mode=indexing
                  tunnel: dbl[] [6000.0, 6400.0, 11700.0, 14600.0, 11000.0] -> [w719] mode=indexing
                  i -> [w722]
                  stop <- w726 stop-if-true
                  n247 = call <vilib>:"High Resolution Relative Seconds.vi"() -> ("relative seconds"=w718:dbl)
                  n248 = while {
                    tunnel: w732 -> [w756]
                    tunnel: w731 -> [w744]
                    tunnel: w730 -> [w755]
                    tunnel: w729 -> [w745]
                    tunnel: w728 -> [w765]
                    tunnel: w727 -> [w760]
                    tunnel: w725 -> [w757]
                    shift-right: [w753] -> w723
                    shift-left: w724 -> [w752]
                    tunnel: w722 -> [w754]
                    tunnel: w721 -> [w748]
                    tunnel: w720 -> [w747]
                    tunnel: w719 -> [w746]
                    tunnel: w718 -> [w740]
                    stop <- w742 stop-if-true
                    n249 = call "DegToDAC (SubVI).vi"("R2"=0.0, "Rt"=w752) -> ("error out"=w772:errorcluster, "output array"=w773:u8[])  [unwired: 8 in]
                    n250 = call <vilib>:"High Resolution Relative Seconds.vi"() -> ("relative seconds"=w739:dbl)
                    n251 = property on="VISA Tester" class="VISAName"() -> ("Value"=w775:refnum<visa-resource-name>)  [unwired: 2 in, 2 out]
                    n252 = Byte Array To String(unsigned byte array=w773) -> (string=w774:string)
                    n253 = Subtract(x=w740, y=w739) -> (x-y=w738:dbl)
                    n254 = VISA Write(VISA resource name=w775, write buffer=w774, error in (no error)=w772) -> (error out=w771:errorcluster)  [unwired: 2 out]
                    n255 = Greater Or Equal?(x=w738, y=120.0) -> (x >= y?=w736:bool)
                    n256 = call <vilib>:"Clear Errors.vi"("error in (no error)"=w771) -> ("error out"=w770:errorcluster)  [unwired: 5 in, 1 out]
                    n257 = call "Write panel message (SubVI).vi"("Stop BurnIn"=w755, 4:"rpm"=w765, 5:"rpm"=TRUE ("rpm"), "PrintTime"=TRUE, "Stop"=w744, "error in (no error)"=w770, "Time to wait"=3.0, "Strin"=w745, "String in"=w756) -> ("error out"=w769:errorcluster)  [unwired: 2 in]
                    n258 = control-ref of="Power transistor Heat sink Temp."() -> (w764:refnum<vi>)
                    n259 = call "TempAlgoTest (SubVI).vi"("Temp"=w764, "Speed Ind"=w746, "Motor Speed RPM"=w765, "Round"=w754, "Temp Up In"=w752, "error in (no error)"=w769, "String in"=w756, "Temp Goal"=w748, "Stop"=w744, "Speed Goal"=w747, "Stop BurnIn"=w755, "Strin"=w745) -> (14:"Speed Pass/Fail"=w741:bool, "Temp  Pass/Fail"=w751:dbl, "Temp Up Out"=w753:dbl, 17:"Speed Pass/Fail"=w749:dbl, "Temp Pass/Fail"=w750:bool, "error out"=w763:errorcluster)  [unwired: 2 in]
                    n260 = call "Find_Number_LineMARVIN.vi"("Test Paragraph"=w757, "error in"=w763, "TableIn"=w760) -> ("error out"=w762:errorcluster, "Line number"=w759:i32)  [unwired: 2 in, 2 out]
                    n261 = property class="Bool (strict)"(reference=w744) -> ("Value"=w743:bool)  [unwired: 1 in, 2 out]
                    n262 = call "PassOrFail (SubVI).vi"("index (row)"=w759, "error in (no error)"=w762, "Data in"=w751, "Pass?Fail"=w750, "Table in"=w760) -> ("error out"=w761:errorcluster)  [unwired: 6 in]
                    n263 = Increment(x=w759) -> (x+1=w758:i32)
                    n264 = call "PassOrFail (SubVI).vi"("index (row)"=w758, "error in (no error)"=w761, "Data in"=w749, "Pass?Fail"=w741, "Table in"=w760) -> ()  [unwired: 6 in, 1 out]
                    n265 = Compound Arithmetic op=OR(w736, w741, w743) -> (w742:bool)
                  }
                  n266 = property class="Bool (strict)"(reference=w731) -> ("Value"=w726:bool)  [unwired: 1 in, 2 out]
                  n267 = Select(t=enum16{"Stop", "Algorithm", "Start"}."Stop", s=w726, f=enum16{"Stop", "Algorithm", "Start"}."Algorithm") -> (s? t:f=w733:enum16{"Stop", "Algorithm", "Start"})
                }
              }
              frame "Start" {
                n268 = property on="VISA Tester" class="VISAName"() -> ("Value"=w789:refnum<visa-resource-name>)  [unwired: 2 in, 2 out]
                n269 = call "TesterOption (SubVI).vi"("On/Off 2"=TRUE, "Tester Option 2"=T11."Venable", "2 Options"=TRUE, "error in (no error)"=w790, "On/Off"=TRUE, "Tester Option"=T11."K15", "VISA Refnum in"=w789) -> ("error out"=w777:errorcluster)  [unwired: 3 in, 1 out]
                n270 = property class="Bool (strict)"(reference=w783, error in=w777) -> ("Value"=w782:bool)  [unwired: 2 out]
                n271 = Select(t=enum16{"Stop", "Algorithm", "Start"}."Stop", s=w782, f=enum16{"Stop", "Algorithm", "Start"}."Algorithm") -> (s? t:f=w779:enum16{"Stop", "Algorithm", "Start"})
              }
            }
          }
        }
        frame "Burn in" {
          n272 = control-ref of="Stop Button"() -> (w792:refnum<vi>)
          n273 = control-ref of="Pannel User Message"() -> (w795:refnum<vi>)
          n274 = control-ref of="ATR"() -> (w791:refnum<vi>)
          n275 = control-ref of="Config_CANAT"() -> (w794:refnum<vi>)
          n276 = control-ref of="UUT"() -> (w793:refnum<vi>)
          n277 = while {
            tunnel: w795 -> [w804]
            tunnel: w791 -> [w803]
            tunnel: w794 -> [w802]
            tunnel: w793 -> [w801]
            tunnel: w792 -> [w800]
            shift-right: [w799] -> _
            shift-left: T15."Start" -> [w806]
            shift-right: [w805] -> _
            shift-left: _ -> [w797]
            stop <- w798 stop-if-true
            n278 = case shown="\"DC Current Measure\"" w806 {
              tunnel: [w809 w836 w901 w929 w957 w984] -> w805
              tunnel: w804 -> [_ w827 _ _ _ w983]
              tunnel: w803 -> [_ w830 w869 w911 w938 w968]
              tunnel: w802 -> [_ w826 _ _ _ w982]
              tunnel: w801 -> [_ w822 w884 w912 w946 w981]
              tunnel: w800 -> [_ _ w903 w931 w961 w974]
              tunnel: [w807 T15."Stop" w904 w932 w962 w970] -> w799
              tunnel: [w808 FALSE FALSE FALSE FALSE FALSE] -> w798
              tunnel: w797 -> [w809 w836 w901 w929 w957 _]
              frame "Stop", Default {
                n279 = flat-sequence {
                  tunnel: [TRUE] -> w808
                  tunnel: [T15."Stop"] -> w807
                  frame #0 {
                    n280 = property on="VISA Tester" class="VISAName"() -> ("Value"=w813:refnum<visa-resource-name>)  [unwired: 2 in, 2 out]
                    n281 = call "TesterOption (SubVI).vi"("On/Off"=FALSE, "Tester Option"=T11."Power", "VISA Refnum in"=w813) -> ("error out"=w810:errorcluster)  [unwired: 7 in, 1 out]
                    n282 = property on="Stop Burn-in" class="Bool (strict)"(error in=w810, "Visible"=FALSE) -> ()  [unwired: 1 in, 2 out]
                  }
                  frame #1 {
                  }
                }
              }
              frame "BurnIn" {
                w817 = FALSE ("Stop Burn-in")
                n283 = control-ref of="Motor Speed RPM"() -> (w829:refnum<vi>)
                n284 = control-ref of="Stop Button"() -> (w828:refnum<vi>)
                n285 = property on="Stop Burn-in" class="Bool (strict)"("Visible"=TRUE) -> (error out=w831:errorcluster)  [unwired: 2 in, 1 out]
                n286 = property class="DigNum (strict)"(reference=w822) -> ("Value"=w825:u8)  [unwired: 1 in, 2 out]
                n287 = call "Find_Number_LineMARVIN.vi"("Test Paragraph"="7.5.7.4", "error in"=w831, "TableIn"=w830) -> ("error out"=w834:errorcluster, "Line number"=w835:i32)  [unwired: 2 in, 2 out]
                n288 = Equal?(x=w825, y=u8 95) -> (x = y?=w821:bool)
                n289 = Select(t=u16 15100, s=w821, f=u16 12100 ("y")) -> (s? t:f=w819:u16)
                n290 = for {
                  tunnel: w834 -> [w853]
                  tunnel: dbl[] [600.0, 600.0, 600.0] -> [w857] mode=indexing
                  tunnel: w835 -> [w863]
                  tunnel: w830 -> [w852]
                  tunnel: w829 -> [w851]
                  tunnel: w828 -> [w850]
                  tunnel: w827 -> [w849]
                  tunnel: w826 -> [w844]
                  tunnel: w822 -> [w843]
                  tunnel: w819 -> [w842]
                  tunnel: [w840] -> w818
                  i -> [w859]
                  n291 = call "CANSendMotorSpeed.vi"("Remote"=TRUE, "error in (no error)"=w853, "Motor Speed RPM"=w842, "UUT"=w843, "CAN Cluster in"=w844) -> ("error out"=w846:errorcluster)  [unwired: 6 in]
                  n292 = control-ref of="Stop Burn-in"() -> (w847:refnum<vi>)
                  n293 = Add(x=w863, y=w859) -> (x+y=w858:i32)
                  n294 = call "Write panel message (SubVI).vi"("Stop BurnIn"=w847, 4:"rpm"=w851, 5:"rpm"=TRUE ("rpm"), "PrintTime"=TRUE, "Stop"=w850, "error in (no error)"=w846, "Time to wait"=w857, "Strin"="7.5.7 Burn-in test in process...", "String in"=w849) -> ("error out"=w854:errorcluster)  [unwired: 2 in]
                  n295 = control-ref of="Power transistor Heat sink Temp."() -> (w864:refnum<vi>)
                  n296 = property on="MaxBurnInTempVal" class="DigNum (strict)"() -> ("Value"=w862:dbl)  [unwired: 2 in, 2 out]
                  n297 = property class="DigNum (strict)"(reference=w864, error in=w854) -> (error out=w841:errorcluster, "Value"=w860:dbl)  [unwired: 1 out]
                  n298 = Less Or Equal?(x=w860, y=w862) -> (x <= y?=w861:bool)
                  n299 = call "PassOrFail (SubVI).vi"("index (row)"=w858, "error in (no error)"=w841, "Data in"=w860, "Pass?Fail"=w861, "Table in"=w852) -> ("error out"=w840:errorcluster)  [unwired: 6 in]
                }
                n300 = property on="Stop Burn-in" class="Bool (strict)"(error in=w818, "Value"=w817, "Visible"=w817) -> ()  [unwired: 1 in, 2 out]
              }
              frame "Ambient Temp" {
                w874 = 2 ("disabled index (col)")
                n301 = control-ref of="Ambient Temperature"() -> (w885:refnum<vi>)
                n302 = property class="DigNum (strict)"(reference=w884) -> ("Value"=w896:u8)  [unwired: 1 in, 2 out]
                n303 = call "Find_Number_LineMARVIN.vi"("Test Paragraph"="7.5.7.3", "TableIn"=w869) -> ("error out"=w899:errorcluster, "Line number"=w875:i32)  [unwired: 3 in, 2 out]
                n304 = property class="DigNum (strict)"(reference=w885, error in=w899) -> (error out=w887:errorcluster, "Value"=w876:dbl)  [unwired: 1 out]
                n305 = Equal?(x=w896, y=u8 95) -> (x = y?=w892:bool)
                n306 = Select(t=25.0 ("y"), s=w892, f=25.0 ("y")) -> (s? t:f=w886:dbl)
                n307 = Select(t=13.0 ("y"), s=w892, f=13.0) -> (s? t:f=w889:dbl)
                n308 = Add(x=w886, y=w889) -> (x+y=w898:dbl)
                n309 = Subtract(x=w886, y=w889) -> (x-y=w897:dbl)
                n310 = In Range and Coerce(upper limit=w898, x=w876, lower limit=w897) -> (In Range?=w888:bool)  [unwired: 1 out]
                n311 = call "PassOrFail (SubVI).vi"("index (row)"=w875, "error in (no error)"=w887, "Data in"=w876, "Pass?Fail"=w888, "Table in"=w869) -> ("error out"=w866:errorcluster)  [unwired: 6 in]
                n312 = property class="Tbl (strict)"(reference=w869, error in=w866) -> (reference out=w868:refnum<vi>, error out=w883:errorcluster, "Value"=w882:string[][])
                n313 = Add(x=w876, y=25.0) -> (x+y=w867:dbl)
                "MaxBurnInTempVal" <- w867
                n314 = Number To Fractional String(number=w867, precision (6)=i16 0) -> (F-format string=w881:string)  [unwired: 2 in]
                n315 = Concatenate Strings("< " ("string"), w881) -> (w870:string)
                n316 = Increment(x=w875) -> (x+1=w873:i32)
                n317 = Increment(x=w873) -> (x+1=w872:i32)
                n318 = Increment(x=w872) -> (x+1=w871:i32)
                n319 = Replace Array Subset(array=w882, new element #1=w870, index (row) #1=w873, index (col) #1=w874, new element #2=w870, index (row) #2=w872, index (col) #2=w874, new element #3=w870, index (row) #3=w871, index (col) #3=w874) -> (w880:string[][])
                n320 = property class="Tbl (strict)"(reference=w868, error in=w883, "Value"=w880) -> (error out=w865:errorcluster)  [unwired: 1 out]
                n321 = property class="Bool (strict)"(reference=w903, error in=w865) -> ("Value"=w907:bool)  [unwired: 2 out]
                n322 = Select(t=T15."Stop", s=w907, f=T15."BurnIn") -> (s? t:f=w904:T15)
              }
              frame "MotorSpeed" {
                n323 = property class="DigNum (strict)"(reference=w912) -> ("Value"=w924:u8)  [unwired: 1 in, 2 out]
                n324 = control-ref of="Motor Speed RPM"() -> (w909:refnum<vi>)
                n325 = call "Find_Number_LineMARVIN.vi"("Test Paragraph"="7.5.7.2", "TableIn"=w911) -> ("error out"=w927:errorcluster, "Line number"=w915:i32)  [unwired: 3 in, 2 out]
                n326 = Equal?(x=w924, y=u8 95) -> (x = y?=w920:bool)
                n327 = property class="DigNum (strict)"(reference=w909, error in=w927) -> (error out=w913:errorcluster, "Value"=w914:dbl)  [unwired: 1 out]
                n328 = Select(t=15100.0 ("y"), s=w920, f=12100.0 ("y")) -> (s? t:f=w910:dbl)
                n329 = Select(t=400.0 ("y"), s=w920, f=200.0) -> (s? t:f=w917:dbl)
                n330 = Add(x=w910, y=w917) -> (x+y=w926:dbl)
                n331 = Subtract(x=w910, y=w917) -> (x-y=w925:dbl)
                n332 = In Range and Coerce(upper limit=w926, x=w914, lower limit=w925) -> (In Range?=w916:bool)  [unwired: 1 out]
                n333 = call "PassOrFail (SubVI).vi"("index (row)"=w915, "error in (no error)"=w913, "Data in"=w914, "Pass?Fail"=w916, "Table in"=w911) -> ("error out"=w908:errorcluster)  [unwired: 6 in]
                n334 = property class="Bool (strict)"(reference=w931, error in=w908) -> ("Value"=w935:bool)  [unwired: 2 out]
                n335 = Select(t=T15."Stop", s=w935, f=T15."Ambient Temp") -> (s? t:f=w932:T15)
              }
              frame "DC Current Measure" {
                n336 = property on="VISA Tester" class="VISAName"() -> (error out=w954:errorcluster, "Value"=w959:refnum<visa-resource-name>)  [unwired: 2 in, 1 out]
                n337 = property class="DigNum (strict)"(reference=w946) -> ("Value"=w950:u8)  [unwired: 1 in, 2 out]
                n338 = call "GetADCTester (SubVI).vi"("error in (no error)"=w954, "GetADCTester"=T13."Current", "VISA Refnum in"=w959) -> ("error out"=w955:errorcluster, "ADCValOutput Single"=w937:u32)  [unwired: 6 in, 1 out]
                n339 = call "Find_Number_LineMARVIN.vi"("Test Paragraph"="7.5.7.1", "error in"=w955, "TableIn"=w938) -> ("error out"=w953:errorcluster, "Line number"=w939:i32)  [unwired: 2 in, 2 out]
                n340 = Equal?(x=w950, y=u8 95) -> (x = y?=w945:bool)
                n341 = Select(t=50.0 ("y"), s=w945, f=28.0 ("y")) -> (s? t:f=w942:dbl)
                n342 = Select(t=5.0 ("y"), s=w945, f=2.0) -> (s? t:f=w941:dbl)
                n343 = Add(x=w942, y=w941) -> (x+y=w952:dbl)
                n344 = Subtract(x=w942, y=w941) -> (x-y=w951:dbl)
                n345 = In Range and Coerce(upper limit=w952, x=w937, lower limit=w951) -> (In Range?=w940:bool)  [unwired: 1 out]
                n346 = call "PassOrFail (SubVI).vi"("index (row)"=w939, "error in (no error)"=w953, "Data in"=w937, "Pass?Fail"=w940, "Table in"=w938) -> ("error out"=w936:errorcluster)  [unwired: 6 in]
                n347 = property class="Bool (strict)"(reference=w961, error in=w936) -> ("Value"=w965:bool)  [unwired: 2 out]
                n348 = Select(t=T15."Stop", s=w965, f=T15."MotorSpeed") -> (s? t:f=w962:T15)
              }
              frame "Start" {
                w978 = "7.5.7 Burn-in test in process...\nFull Speed Operation" ("Value")
                w985 = "7.5.7" ("Test Paragraph")
                n349 = property class="Str"(reference=w983, "Value"=w978) -> (reference out=w979:refnum<vi>, error out=w992:errorcluster)  [unwired: 1 in]
                n350 = property class="DigNum (strict)"(reference=w981) -> ("Value"=w1000:u8)  [unwired: 1 in, 2 out]
                n351 = call "Find_Number_LineMARVIN.vi"("Test Paragraph"=w985, "error in"=w992, "TableIn"=w968) -> ("error out"=w993:errorcluster, "Line number"=w994:i32)  [unwired: 2 in, 2 out]
                n352 = Equal?(x=w1000, y=u8 95) -> (x = y?=w1001:bool)
                n353 = call "Table_ScrollaBarMarvin.vi"("error in"=w993, "Line to focus"=w985, "reference in"=w968) -> ("error out"=w995:errorcluster)  [unwired: 2 out]
                n354 = Select(t=u16 15100 ("y"), s=w1001, f=u16 12100 ("y")) -> (s? t:f=w1002:u16)
                n355 = call "Reset old test Values (SubVI).vi"("error in"=w995, "Atr in"=w968, "Test Paragraph"=w985) -> ("error out"=w996:errorcluster)  [unwired: 8 in]
                n356 = Increment(x=w994) -> (x+1=w984:i32)
                n357 = property on="VISA Tester" class="VISAName"(error in=w996) -> (error out=w997:errorcluster, "Value"=w998:refnum<visa-resource-name>)  [unwired: 1 in, 1 out]
                n358 = call "TesterOption (SubVI).vi"("error in (no error)"=w997, "On/Off"=TRUE, "Tester Option"=T11."Venable", "VISA Refnum in"=w998) -> ("error out"=w999:errorcluster)  [unwired: 6 in, 1 out]
                n359 = call "CANSendMotorSpeed.vi"("Remote"=TRUE, "error in (no error)"=w999, "Motor Speed RPM"=w1002, "UUT"=w981, "CAN Cluster in"=w982) -> ("error out"=w980:errorcluster)  [unwired: 6 in]
                n360 = control-ref of="Motor Speed RPM"() -> (w967:refnum<vi>)
                n361 = call "Write panel message (SubVI).vi"(4:"rpm"=w967, 5:"rpm"=TRUE ("rpm"), "PrintTime"=TRUE, "Stop"=w974, "error in (no error)"=w980, "Time to wait"=15.0, "Strin"=w978, "String in"=w979) -> ("error out"=w966:errorcluster)  [unwired: 3 in]
                n362 = property class="Bool (strict)"(reference=w974, error in=w966) -> ("Value"=w973:bool)  [unwired: 2 out]
                n363 = Select(t=T15."Stop", s=w973, f=T15."DC Current Measure") -> (s? t:f=w970:T15)
              }
            }
          }
        }
        frame "Visual Inspec" {
          n364 = call "VisualInspection.vi"("error in (no error)"=w1004, "TableRef"=w1003) -> ()  [unwired: 9 in, 1 out]
        }
        frame "Temp Sens Cal" {
          w1005 = "7.5.5 Temperature sensor calibration test in process..." ("Value")
          w1017 = "7.5.5" ("Test Paragraph")
          n365 = control-ref of="Pannel User Message"() -> (w1013:refnum<vi>)
          n366 = property class="Str"(reference=w1013, error in=w1012, "Value"=w1005) -> (error out=w1011:errorcluster)  [unwired: 1 out]
          n367 = call "Table_ScrollaBarMarvin.vi"("error in"=w1011, "Line to focus"=w1017, "reference in"=w1014) -> ("error out"=w1016:errorcluster)  [unwired: 2 out]
          n368 = property class="Tbl (strict)"(reference=w1014, error in=w1016) -> (reference out=w1008:refnum<vi>, error out=w1019:errorcluster, "Value"=w1020:string[][])
          n369 = Index Array(array=w1020, index (col)=0 ("disabled index (col)")) -> (element=w1021:string[])  [unwired: 1 in]
          n370 = call "Find_Number_Line.vi"("error in"=w1019, "Test Paragraph"=w1017, "Row Headers[]"=w1021) -> ("error out"=w1015:errorcluster, "Line number"=w1007:i32)  [unwired: 1 out]
          n371 = property on="Status" class="Bool (strict)"(error in=w1015) -> (error out=w1009:errorcluster, "Value"=w1010:bool)  [unwired: 1 in, 1 out]
          n372 = case shown="True" w1010 {
            selector: w1010 -> [w1025 _]
            tunnel: w1009 -> [w1027 _]
            tunnel: w1008 -> [w1024 _]
            tunnel: w1007 -> [w1023 _]
            tunnel: w1006 -> [_ w1034]
            tunnel: w1005 -> [_ w1030]
            frame False {
              n373 = flat-sequence {
                tunnel: w1027 -> [w1028]
                tunnel: [w1028] -> w1026
                frame #0 {
                  n374 = One Button Dialog(message="Please establish RS connection.") -> ()  [unwired: 1 in, 1 out]
                }
              }
              n375 = Increment(x=w1023) -> (x+1=w1022:i32)
              n376 = call "PassOrFail (SubVI).vi"("index (row)"=w1022, "error in (no error)"=w1026, "Pass?Fail"=w1025, "Table in"=w1024) -> ()  [unwired: 7 in, 1 out]
            }
            frame True {
              n377 = control-ref of="Stop Burn-in"() -> (w1036:refnum<vi>)
              n378 = control-ref of="Pannel User Message"() -> (w1038:refnum<vi>)
              n379 = control-ref of="Config_CANAT"() -> (w1032:refnum<vi>)
              n380 = control-ref of="ATR"() -> (w1039:refnum<vi>)
              n381 = control-ref of="Motor Speed RPM"() -> (w1040:refnum<vi>)
              n382 = control-ref of="UUT"() -> (w1031:refnum<vi>)
              n383 = control-ref of="Stop Button"() -> (w1037:refnum<vi>)
              n384 = property on="VISA Tester" class="VISAName"() -> ("Value"=w1033:refnum<visa-resource-name>)  [unwired: 2 in, 2 out]
              n385 = while {
                shift-right: [w1043] -> _
                shift-left: T14."Start" -> [w1053]
                tunnel: w1036 -> [w1052]
                tunnel: w1037 -> [w1051]
                tunnel: w1038 -> [w1050]
                tunnel: w1039 -> [w1049]
                tunnel: w1040 -> [w1048]
                tunnel: w1034 -> [w1047]
                tunnel: w1033 -> [w1046]
                tunnel: w1032 -> [w1045]
                tunnel: w1031 -> [w1044]
                tunnel: w1030 -> [w1041]
                stop <- w1042 stop-if-true
                n386 = case shown="\"TA[5]\"" w1053 {
                  tunnel: w1052 -> [_ w1087 w1114 w1169 w1199]
                  tunnel: w1051 -> [_ w1088 w1106 w1155 w1201]
                  tunnel: w1050 -> [_ w1085 w1115 w1167 w1203]
                  tunnel: w1049 -> [_ w1064 _ _ _]
                  tunnel: w1048 -> [_ w1089 w1113 w1170 w1198]
                  tunnel: w1047 -> [_ w1098 w1118 w1179 w1195]
                  tunnel: w1046 -> [w1056 w1094 w1117 w1175 w1183]
                  tunnel: w1045 -> [_ _ _ _ w1209]
                  tunnel: w1044 -> [_ _ _ _ w1208]
                  tunnel: [w1054 w1074 w1107 w1158 w1186] -> w1043
                  tunnel: [w1055 FALSE FALSE FALSE FALSE] -> w1042
                  tunnel: w1041 -> [_ _ w1116 _ _]
                  frame "Stop", Default {
                    n387 = flat-sequence {
                      tunnel: w1056 -> [w1057]
                      tunnel: [TRUE] -> w1055
                      tunnel: [T14."Stop"] -> w1054
                      frame #0 {
                        n388 = call "TesterOption (SubVI).vi"("2 Options"=FALSE, "On/Off"=FALSE, "Tester Option"=T11."Power", "VISA Refnum in"=w1057) -> ()  [unwired: 6 in, 2 out]
                      }
                      frame #1 {
                      }
                    }
                  }
                  frame "AO[1]=Meas." {
                    n389 = property on="AO[1]Meas" class="DigNum (strict)"() -> ("Value"=w1067:dbl)  [unwired: 2 in, 2 out]
                    n390 = Number To Fractional String(number=w1067) -> (F-format string=w1076:string)  [unwired: 3 in]
                    n391 = Search and Replace String(input string="EP=1\r\nAO[1]=0\r\n" ("write buffer"), search string="0", replace string=w1076) -> (result string=w1075:string)  [unwired: 5 in, 3 out]
                    n392 = call "SerialMarvinSendGet.vi"("Clear Log"=FALSE, "write buffer"=w1075, "VISA resource name"=w1098) -> ("error out"=w1093:errorcluster)  [unwired: 7 in, 1 out]
                    n393 = call "TesterOption (SubVI).vi"("2 Options"=FALSE, "error in (no error)"=w1093, "On/Off"=FALSE, "Tester Option"=T11."Power", "VISA Refnum in"=w1094) -> ("error out"=w1092:errorcluster, "VISA Refnum out"=w1079:refnum<visa-resource-name>)  [unwired: 5 in]
                    n394 = call "Write panel message (SubVI).vi"("Stop BurnIn"=w1087, 4:"rpm"=w1089, 5:"rpm"=FALSE ("rpm"), "PrintTime"=TRUE, "Stop"=w1088, "error in (no error)"=w1092, "Time to wait"=20.0, "Strin"="7.5.5 Temperature sensor calibration test in process...\nSet Parameters...", "String in"=w1085) -> ("error out"=w1080:errorcluster)  [unwired: 2 in]
                    n395 = call "TesterOption (SubVI).vi"("2 Options"=FALSE, "error in (no error)"=w1080, "On/Off"=FALSE, "Tester Option"=T11."Venable", "VISA Refnum in"=w1079) -> ("error out"=w1073:errorcluster)  [unwired: 5 in, 1 out]
                    n396 = flat-sequence {
                      tunnel: [T14."Stop"] -> w1074
                      tunnel: w1065 -> [_]
                      frame #0 {
                      }
                    }
                    n397 = In Range and Coerce(upper limit=0.1, x=w1067, lower limit=-0.1) -> (In Range?=w1068:bool)  [unwired: 1 out]
                    n398 = call "Find_Number_LineMARVIN.vi"("Test Paragraph"="7.5.5.1", "error in"=w1073, "TableIn"=w1064) -> ("error out"=w1066:errorcluster, "Line number"=w1071:i32)  [unwired: 2 in, 2 out]
                    n399 = call "PassOrFail (SubVI).vi"("index (row)"=w1071, "error in (no error)"=w1066, "Data in"=w1067, "Pass?Fail"=w1068, "Table in"=w1064) -> ("error out"=w1065:errorcluster)  [unwired: 6 in]
                  }
                  frame "TA[5]" {
                    w1119 = T17 [enum."50C", enum."80C", enum."100C", enum."120C"] items=["K15", "K16", "K17", "Venable", "Firmeware", "Fan", "Power", "120C", "110C", "100C", "90C", "80C", "70C", "60C", "50C", "40C", "30C", "25C", "20C", "10C", "0C"]
                    n400 = for {
                      tunnel: w1119 -> [w1134] mode=indexing
                      tunnel: w1118 -> [w1133]
                      tunnel: w1117 -> [w1132]
                      tunnel: w1116 -> [w1131]
                      tunnel: w1115 -> [w1130]
                      tunnel: w1106 -> [w1129]
                      tunnel: w1114 -> [w1128]
                      tunnel: w1113 -> [w1127]
                      tunnel: dbl[] [0.59774, 0.65238, 0.68545, 0.71584] -> [w1122] mode=indexing
                      tunnel: [w1121] -> w1102 mode=indexing
                      tunnel: [w1120] -> w1105
                      n401 = for {
                        N: 5 -> [_]
                        tunnel: w1134 -> [w1152]
                        tunnel: w1133 -> [w1151]
                        tunnel: w1132 -> [w1147]
                        tunnel: w1131 -> [w1145]
                        tunnel: w1130 -> [w1144]
                        tunnel: w1129 -> [w1143]
                        tunnel: w1128 -> [w1141]
                        tunnel: w1127 -> [w1138]
                        tunnel: [w1137] -> w1126 mode=indexing
                        tunnel: [w1136] -> w1120
                        n402 = call "TesterOption (SubVI).vi"("2 Options"=FALSE, "On/Off"=TRUE, "Tester Option"=w1152, "VISA Refnum in"=w1147) -> ("error out"=w1148:errorcluster)  [unwired: 6 in, 1 out]
                        n403 = call "Write panel message (SubVI).vi"("Stop BurnIn"=w1141, 4:"rpm"=w1138, 5:"rpm"=FALSE ("rpm"), "PrintTime"=FALSE, "Stop"=w1143, "error in (no error)"=w1148, "Time to wait"=1.0, "Strin"=w1145, "String in"=w1144) -> ("error out"=w1146:errorcluster)  [unwired: 2 in]
                        n404 = call "SerialMarvinSendGet.vi"("error in (no error)"=w1146, "write buffer"="TA[5]\r\n", "VISA resource name"=w1151) -> ("error out"=w1136:errorcluster, "read buffer"=w1149:string)  [unwired: 7 in]
                        n405 = Fract/Exp String To Number(string=w1149) -> (number=w1137:dbl)  [unwired: 3 in, 1 out]
                      }
                      n406 = Add Array Elements(numeric array=w1126) -> (sum=w1125:dbl)
                      n407 = Divide(x=w1125, y=5.0) -> (x/y=w1123:dbl)
                      n408 = Subtract(x=w1123, y=w1122) -> (x-y=w1121:dbl)
                    }
                    n409 = property class="Bool (strict)"(reference=w1106, error in=w1105) -> ("Value"=w1111:bool)  [unwired: 2 out]
                    n410 = Select(t=T14."Stop", s=w1111, f=T14."AO[1]=Meas.") -> (s? t:f=w1107:T14)
                    n411 = Add Array Elements(numeric array=w1102) -> (sum=w1103:dbl)
                    n412 = Divide(x=w1103, y=4.0) -> (x/y=→"AO[1]Meas":dbl)
                  }
                  frame "AO[1]=0" {
                    n413 = call "SerialMarvinSendGet.vi"("write buffer"="EP=1\nAO[1]=0\r\n", "VISA resource name"=w1179) -> ("error out"=w1174:errorcluster)  [unwired: 8 in, 1 out]
                    n414 = call "TesterOption (SubVI).vi"("2 Options"=FALSE, "error in (no error)"=w1174, "On/Off"=FALSE, "Tester Option"=T11."Power", "VISA Refnum in"=w1175) -> ("error out"=w1173:errorcluster, "VISA Refnum out"=w1161:refnum<visa-resource-name>)  [unwired: 5 in]
                    n415 = call "Write panel message (SubVI).vi"("Stop BurnIn"=w1169, 4:"rpm"=w1170, 5:"rpm"=FALSE ("rpm"), "PrintTime"=TRUE, "Stop"=w1155, "error in (no error)"=w1173, "Time to wait"=20.0, "Strin"="7.5.5 Temperature sensor calibration test in process...\nSet Parameters...", "String in"=w1167) -> ("error out"=w1162:errorcluster)  [unwired: 2 in]
                    n416 = call "TesterOption (SubVI).vi"("2 Options"=FALSE, "error in (no error)"=w1162, "On/Off"=FALSE, "Tester Option"=T11."Venable", "VISA Refnum in"=w1161) -> ("error out"=w1156:errorcluster)  [unwired: 5 in, 1 out]
                    n417 = property class="Bool (strict)"(reference=w1155, error in=w1156) -> ("Value"=w1160:bool)  [unwired: 2 out]
                    n418 = Select(t=T14."Stop", s=w1160, f=T14."TA[5]") -> (s? t:f=w1158:T14)
                  }
                  frame "Start" {
                    n419 = call "Write panel message (SubVI).vi"("Stop BurnIn"=w1199, 4:"rpm"=w1198, 5:"rpm"=FALSE ("rpm"), "PrintTime"=FALSE, "Stop"=w1201, "Time to wait"=0.1, "Strin"="7.5.5 Temperature sensor calibration test in process...\nInitialization state...", "String in"=w1203) -> ("error out"=w1204:errorcluster)  [unwired: 3 in]
                    n420 = call "TesterOption (SubVI).vi"("2 Options"=FALSE, "error in (no error)"=w1204, "On/Off"=FALSE, "Tester Option"=T11."Venable", "VISA Refnum in"=w1183) -> ("error out"=w1206:errorcluster)  [unwired: 5 in, 1 out]
                    n421 = call "CANSendMotorSpeed.vi"("Remote"=TRUE, "error in (no error)"=w1206, "Motor Speed RPM"=u16 0, "UUT"=w1208, "CAN Cluster in"=w1209) -> ("error out"=w1193:errorcluster)  [unwired: 6 in]
                    n422 = call "SerialMarvinSendGet.vi"("error in (no error)"=w1193, "write buffer"="AO[1]\r\n", "VISA resource name"=w1195) -> ("error out"=w1182:errorcluster, "read buffer"=w1192:string)  [unwired: 7 in]
                    n423 = Equal?(x=w1192, y="0.0") -> (x = y?=w1184:bool)
                    n424 = property class="Bool (strict)"(reference=w1201, error in=w1182) -> ("Value"=w1213:bool)  [unwired: 2 out]
                    n425 = Select(t=T14."TA[5]", s=w1184, f=T14."AO[1]=0") -> (s? t:f=w1188:T14)
                    n426 = Select(t=T14."Stop", s=w1213, f=w1188) -> (s? t:f=w1186:T14)
                  }
                }
              }
            }
          }
        }
        frame "Auxiliary" {
          w1217 = "8. Auxiliary test in process..." ("Value")
          w1229 = "8" ("Test Paragraph")
          n427 = control-ref of="Pannel User Message"() -> (w1228:refnum<vi>)
          n428 = property class="Str"(reference=w1228, error in=w1225, "Value"=w1217) -> (error out=w1227:errorcluster)  [unwired: 1 out]
          n429 = call "Table_ScrollaBarMarvin.vi"("error in"=w1227, "Line to focus"=w1229, "reference in"=w1226) -> ("error out"=w1235:errorcluster)  [unwired: 2 out]
          n430 = property class="Tbl (strict)"(reference=w1226, error in=w1235) -> (reference out=w1224:refnum<vi>, error out=w1234:errorcluster, "Value"=w1233:string[][])
          n431 = Index Array(array=w1233, index (col)=0 ("disabled index (col)")) -> (element=w1232:string[])  [unwired: 1 in]
          n432 = call "Find_Number_Line.vi"("error in"=w1234, "Test Paragraph"=w1229, "Row Headers[]"=w1232) -> ("error out"=w1230:errorcluster, "Line number"=w1215:i32)  [unwired: 1 out]
          n433 = call "Reset old test Values (SubVI).vi"("error in"=w1230, "Atr in"=w1224, "Test Paragraph"=w1229) -> ("error out"=w1222:errorcluster)  [unwired: 8 in]
          n434 = property on="VISA Tester" class="VISAName"() -> ("Value"=w1216:refnum<visa-resource-name>)  [unwired: 2 in, 2 out]
          n435 = control-ref of="Stop Burn-in"() -> (w1219:refnum<vi>)
          n436 = control-ref of="Stop Button"() -> (w1220:refnum<vi>)
          n437 = control-ref of="Pannel User Message"() -> (w1221:refnum<vi>)
          n438 = control-ref of="ATR"() -> (w1214:refnum<vi>)
          n439 = control-ref of="Config_CANAT"() -> ()  [unwired: 1 out]
          n440 = control-ref of="Motor Speed RPM"() -> (w1218:refnum<vi>)
          n441 = control-ref of="UUT"() -> ()  [unwired: 1 out]
          n442 = while {
            shift-right: [w1240] -> _
            shift-left: enum16{"Stop", "CoolingON", "HotGunON", "Start"}."Start" -> [w1247]
            tunnel: w1222 -> [w1238]
            tunnel: w1221 -> [w1246]
            tunnel: w1220 -> [w1245]
            tunnel: w1219 -> [w1244]
            tunnel: w1218 -> [w1243]
            tunnel: w1217 -> [w1242]
            tunnel: w1216 -> [w1241]
            tunnel: w1215 -> [w1237]
            tunnel: w1214 -> [w1236]
            stop <- w1239 stop-if-true
            n443 = case shown="\"CoolingON\"" w1247 {
              tunnel: w1246 -> [_ w1288 w1359 w1418]
              tunnel: w1245 -> [_ w1280 w1351 w1404]
              tunnel: w1244 -> [_ w1287 w1358 w1417]
              tunnel: w1243 -> [_ w1286 w1357 w1413]
              tunnel: w1242 -> [_ w1273 w1344 w1412]
              tunnel: w1241 -> [_ w1274 w1345 w1405]
              tunnel: [w1249 w1276 w1347 w1400] -> w1240
              tunnel: [w1248 FALSE FALSE FALSE] -> w1239
              tunnel: w1238 -> [_ w1272 w1343 _]
              tunnel: w1237 -> [_ w1266 w1337 _]
              tunnel: w1236 -> [_ w1262 w1334 _]
              frame "Stop", Default {
                n444 = flat-sequence {
                  tunnel: [enum16{"Stop", "CoolingON", "HotGunON", "Start"}."Stop"] -> w1249
                  tunnel: [TRUE] -> w1248
                  frame #0 {
                    n445 = property on="VISA Tester" class="VISAName"() -> ("Value"=w1253:refnum<visa-resource-name>)  [unwired: 2 in, 2 out]
                    n446 = call "TesterOption (SubVI).vi"("2 Options"=FALSE, "On/Off"=FALSE, "Tester Option"=T11."Power", "VISA Refnum in"=w1253) -> ()  [unwired: 6 in, 2 out]
                  }
                  frame #1 {
                  }
                }
              }
              frame "CoolingON" {
                n447 = while {
                  tunnel: w1288 -> [w1321]
                  tunnel: w1287 -> [w1320]
                  tunnel: w1286 -> [w1316]
                  tunnel: [w1312] -> w1269
                  tunnel: w1280 -> [w1303]
                  tunnel: w1274 -> [w1313]
                  tunnel: w1273 -> [w1307]
                  tunnel: w1272 -> [w1304]
                  shift-right: [w1296] -> _
                  shift-left: 0.0 -> [w1297]
                  shift-right: [w1293] -> w1260
                  shift-left: 0.0 ("Value") -> [w1294]
                  tunnel: [w1291] -> w1261
                  tunnel: [w1290] -> w1257
                  stop <- w1301 stop-if-true
                  n448 = control-ref of="Ambient Temperature"() -> (w1314:refnum<vi>)
                  n449 = property class="DigNum (strict)"(reference=w1314, error in=w1304) -> (error out=w1310:errorcluster, "Value"=w1293:dbl)  [unwired: 1 out]
                  n450 = Equal?(x=w1293, y=w1294) -> (x = y?=w1292:bool)
                  n451 = Number To Fractional String(number=w1293, precision (6)=i16 2) -> (F-format string=w1306:string)  [unwired: 2 in]
                  n452 = case shown="True" w1292 {
                    tunnel: w1297 -> [_ w1327]
                    tunnel: [0.0 w1325] -> w1296
                    tunnel: [FALSE w1324] -> w1295
                    frame False {
                    }
                    frame True {
                      n453 = Increment(x=w1327) -> (x+1=w1325:dbl)
                      n454 = Greater Or Equal?(x=w1325, y=600.0) -> (x >= y?=w1324:bool)
                    }
                  }
                  n455 = Concatenate Strings(w1307, "PCB Temperature [C]: " ("string"), w1306) -> (w1305:string)
                  n456 = call "Write panel message (SubVI).vi"("Stop BurnIn"=w1320, 4:"rpm"=w1316, 5:"rpm"=FALSE ("rpm"), "PrintTime"=FALSE, "Stop"=w1303, "error in (no error)"=w1310, "Time to wait"=0.2, "Strin"=w1305, "String in"=w1321) -> ("error out"=w1309:errorcluster)  [unwired: 2 in]
                  n457 = property class="Bool (strict)"(reference=w1303) -> ("Value"=w1302:bool)  [unwired: 1 in, 2 out]
                  n458 = Less Or Equal?(x=w1293, y=56.0) -> (x <= y?=w1291:bool)
                  n459 = call "GetADCTester (SubVI).vi"("error in (no error)"=w1309, "GetADCTester"=T13."Fan", "VISA Refnum in"=w1313) -> ("error out"=w1312:errorcluster, "ADCValOutput Single"=w1299:u32)  [unwired: 6 in, 1 out]
                  n460 = Greater?(x=w1299, y=u32 2) -> (0:w1290:bool)
                  n461 = Compound Arithmetic op=OR(w1290, w1302, w1291, w1295) -> (w1301:bool)
                }
                n462 = Add(x=w1266, y=2) -> (x+y=w1264:i32)
                n463 = call "PassOrFail (SubVI).vi"("index (row)"=w1264, "error in (no error)"=w1269, "Data in"=w1260, "Pass?Fail"=w1261, "Table in"=w1262) -> ("error out"=w1268:errorcluster)  [unwired: 6 in]
                n464 = Select(t=-2, s=w1257, f=-1) -> (s? t:f=w1258:i32)
                n465 = Increment(x=w1264) -> (x+1=w1263:i32)
                n466 = call "PassOrFail (SubVI).vi"("index (row)"=w1263, "error in (no error)"=w1268, "Data in"=w1258, "Pass?Fail"=w1257, "Table in"=w1262) -> ("error out"=w1267:errorcluster)  [unwired: 6 in]
                n467 = call "TesterOption (SubVI).vi"("On/Off 2"=TRUE, "Tester Option 2"=T11."Power", "2 Options"=FALSE, "error in (no error)"=w1267, "On/Off"=FALSE, "Tester Option"=T11."Venable", "VISA Refnum in"=w1274) -> ("error out"=w1279:errorcluster)  [unwired: 3 in, 1 out]
                n468 = property class="Bool (strict)"(reference=w1280, error in=w1279) -> ("Value"=w1289:bool)  [unwired: 2 out]
                n469 = Select(t=enum16{"Stop", "CoolingON", "HotGunON", "Start"}."Stop", s=w1289, f=enum16{"Stop", "CoolingON", "HotGunON", "Start"}."Stop") -> (s? t:f=w1276:enum16{"Stop", "CoolingON", "HotGunON", "Start"})
              }
              frame "HotGunON" {
                n470 = while {
                  tunnel: w1359 -> [w1392]
                  tunnel: w1358 -> [w1391]
                  tunnel: w1357 -> [w1387]
                  tunnel: [w1383] -> w1340
                  tunnel: w1351 -> [w1374]
                  tunnel: w1345 -> [w1384]
                  tunnel: w1344 -> [w1378]
                  tunnel: w1343 -> [w1375]
                  shift-right: [w1367] -> _
                  shift-left: 0.0 -> [w1368]
                  shift-right: [w1364] -> w1333
                  shift-left: 0.0 ("Value") -> [w1365]
                  tunnel: [w1362] -> w1328
                  tunnel: [w1361] -> w1332
                  stop <- w1372 stop-if-true
                  n471 = control-ref of="Ambient Temperature"() -> (w1385:refnum<vi>)
                  n472 = property class="DigNum (strict)"(reference=w1385, error in=w1375) -> (error out=w1381:errorcluster, "Value"=w1364:dbl)  [unwired: 1 out]
                  n473 = Equal?(x=w1364, y=w1365) -> (x = y?=w1363:bool)
                  n474 = Number To Fractional String(number=w1364, precision (6)=i16 2) -> (F-format string=w1377:string)  [unwired: 2 in]
                  n475 = case shown="False" w1363 {
                    tunnel: w1368 -> [_ w1398]
                    tunnel: [0.0 w1396] -> w1367
                    tunnel: [FALSE w1395] -> w1366
                    frame False {
                    }
                    frame True {
                      n476 = Increment(x=w1398) -> (x+1=w1396:dbl)
                      n477 = Greater Or Equal?(x=w1396, y=600.0) -> (x >= y?=w1395:bool)
                    }
                  }
                  n478 = Concatenate Strings(w1378, "PCB Temperature [C]: " ("string"), w1377) -> (w1376:string)
                  n479 = call "Write panel message (SubVI).vi"("Stop BurnIn"=w1391, 4:"rpm"=w1387, 5:"rpm"=FALSE ("rpm"), "PrintTime"=FALSE, "Stop"=w1374, "error in (no error)"=w1381, "Time to wait"=0.2, "Strin"=w1376, "String in"=w1392) -> ("error out"=w1380:errorcluster)  [unwired: 2 in]
                  n480 = property class="Bool (strict)"(reference=w1374) -> ("Value"=w1373:bool)  [unwired: 1 in, 2 out]
                  n481 = Greater Or Equal?(x=w1364, y=58.0) -> (x >= y?=w1361:bool)
                  n482 = call "GetADCTester (SubVI).vi"("error in (no error)"=w1380, "GetADCTester"=T13."Fan", "VISA Refnum in"=w1384) -> ("error out"=w1383:errorcluster, "ADCValOutput Single"=w1370:u32)  [unwired: 6 in, 1 out]
                  n483 = Less?(x=w1370, y=u32 1) -> (x < y?=w1362:bool)
                  n484 = Compound Arithmetic op=OR(w1362, w1373, w1361, w1366) -> (w1372:bool)
                }
                n485 = Increment(x=w1337) -> (x+1=w1336:i32)
                n486 = call "PassOrFail (SubVI).vi"("index (row)"=w1336, "error in (no error)"=w1340, "Data in"=w1333, "Pass?Fail"=w1332, "Table in"=w1334) -> ("error out"=w1339:errorcluster)  [unwired: 6 in]
                n487 = Select(t=-1, s=w1328, f=-2) -> (s? t:f=w1330:i32)
                n488 = Increment(x=w1336) -> (x+1=w1335:i32)
                n489 = call "PassOrFail (SubVI).vi"("index (row)"=w1335, "error in (no error)"=w1339, "Data in"=w1330, "Pass?Fail"=w1328, "Table in"=w1334) -> ("error out"=w1338:errorcluster)  [unwired: 6 in]
                n490 = call "TesterOption (SubVI).vi"("On/Off 2"=TRUE, "Tester Option 2"=T11."Fan", "2 Options"=FALSE, "error in (no error)"=w1338, "On/Off"=FALSE, "Tester Option"=T11."Venable", "VISA Refnum in"=w1345) -> ("error out"=w1350:errorcluster)  [unwired: 3 in, 1 out]
                n491 = property class="Bool (strict)"(reference=w1351, error in=w1350) -> ("Value"=w1360:bool)  [unwired: 2 out]
                n492 = Select(t=enum16{"Stop", "CoolingON", "HotGunON", "Start"}."Stop", s=w1360, f=enum16{"Stop", "CoolingON", "HotGunON", "Start"}."CoolingON") -> (s? t:f=w1347:enum16{"Stop", "CoolingON", "HotGunON", "Start"})
              }
              frame "Start" {
                n493 = call "Write panel message (SubVI).vi"("Stop BurnIn"=w1417, 4:"rpm"=w1413, 5:"rpm"=FALSE ("rpm"), "PrintTime"=FALSE, "Stop"=w1404, "Time to wait"=0.1, "Strin"=w1412, "String in"=w1418) -> ("error out"=w1411:errorcluster)  [unwired: 3 in]
                n494 = call "TesterOption (SubVI).vi"("On/Off 2"=TRUE, "Tester Option 2"=T11."Fan", "2 Options"=TRUE, "error in (no error)"=w1411, "On/Off"=FALSE, "Tester Option"=T11."Venable", "VISA Refnum in"=w1405) -> ("error out"=w1403:errorcluster)  [unwired: 3 in, 1 out]
                n495 = property class="Bool (strict)"(reference=w1404, error in=w1403) -> ("Value"=w1419:bool)  [unwired: 2 out]
                n496 = Select(t=enum16{"Stop", "CoolingON", "HotGunON", "Start"}."Stop", s=w1419, f=enum16{"Stop", "CoolingON", "HotGunON", "Start"}."HotGunON") -> (s? t:f=w1400:enum16{"Stop", "CoolingON", "HotGunON", "Start"})
              }
            }
          }
        }
      }
    }
  }
  n497 = disable-structure shown="Disabled" {
    frame Disabled {
      n498 = property class="Tbl (strict)"() -> (reference=w1434:refnum<vi>, error out=w1433:errorcluster, "Value"=w1426:string[][])  [unwired: 1 in, 1 out]
      n499 = Replace Array Subset(array=w1426, index (row)=0, index (col)=5 ("disabled index (col)")) -> (w1427:string[][], new element=w1430:string)
      n500 = Equal?(x="PASS") -> (y=w1431:string, x = y?=w1421:bool)
      n501 = Select(t=u32 6618880, s=w1421, f=u32 16711680) -> (s? t:f=w1425:u32)
      n502 = property class="Tbl (strict)"(reference=w1434, error in=w1433, "Active Cell"=T18 {"Row"=0, "Column"=5} ("Active Cell:Active Cell"), "Cell BG Color"=w1425) -> (error out=w1432:errorcluster)  [unwired: 1 out]
      n503 = property class="Tbl (strict)"(reference=w1434, error in=w1432, "Value"=w1427) -> ()  [unwired: 2 out]
    }
    frame Enabled {
    }
  }
  n504 = while {
    shift-right: [w1447] -> _
    shift-left: w10 -> [w1449]
    shift-right: [w1445] -> _
    shift-left: _ -> [w1446]
    shift-right: [w1441] -> _
    shift-left: w6 -> [w1441]
    shift-right: [w1439] -> _
    shift-left: w1 -> [w1440]
    shift-right: [w1438] -> _
    shift-left: w1 -> [w1437]
    shift-right: [w1436] -> _
    shift-left: w1 -> [w1435]
    stop <- w1448 stop-if-true
    n505 = Dequeue Element(queue=w1449, error in (no error)=w1441) -> (queue out=w1447:refnum<queue>, element=w1442:T9, error out=w1448:errorcluster)  [unwired: 1 in, 1 out]
    n506 = for {
      tunnel: [w1569] -> w1444 mode=indexing
      tunnel: w1442 -> [w1568] mode=indexing
      tunnel: [w1567] -> w1443 mode=indexing
      n507 = Unbundle By Name(w1568) -> ("aDATA"=w1567:u8[])
      n508 = call "Array Data to Single Num in Hex.vi"("aDATA"=w1567) -> ("Numeric"=w1569:u64)  [unwired: 10 in]
    }
    n509 = Build Array (concatenate)(w1444, w1446) -> (w1445:u64[][])
    "Array" <- w1445
    n510 = for {
      tunnel: w1443 -> [w1457] mode=indexing
      shift-right: [w1454] -> w1439
      shift-left: w1440 -> [w1455]
      shift-right: [w1453] -> w1438
      shift-left: w1437 -> [w1452]
      shift-right: [w1451] -> w1436
      shift-left: w1435 -> [w1450]
      i -> [w1456]
      n511 = case shown="0, Default" w1456 {
        tunnel: w1457 -> [w1496 w1528 w1562]
        tunnel: w1455 -> [w1470 w1517 w1550]
        tunnel: [w1468 w1517 w1550] -> w1454
        tunnel: [w1465 w1516 w1549] -> w1453
        tunnel: w1452 -> [w1464 w1516 w1549]
        tunnel: [w1459 w1515 w1548] -> w1451
        tunnel: w1450 -> [w1458 w1515 w1548]
        frame 0, Default {
          # "Frame ID\n0x18E1273F"
          n512 = Index Array(array=w1496, index #1=0 ("index"), index #2=1 ("index"), index #3=2 ("index"), index #4=3 ("index"), index #5=4 ("index"), index #6=5 ("index"), index #7=6 ("index"), index #8=7 ("index")) -> (element #1=w1480:u8, element #2=w1482:u8, element #3=w1483:u8, element #4=w1487:u8, element #5=w1490:u8, element #6=w1494:u8, element #7=w1495:u8, element #8=w1493:u8)
          n513 = Number To Hexadecimal String(2:w1493) -> (0:w1507:string)  [unwired: 1 in]
          n514 = Join Numbers(hi=w1495, lo=w1494) -> ((hi.lo)=w1514:u16)
          n515 = Join Numbers(hi=w1483, lo=w1482) -> ((hi.lo)=w1484:u16)
          n516 = Number To Hexadecimal String(2:w1490) -> (0:w1491:string)  [unwired: 1 in]
          n517 = Number To Hexadecimal String(2:w1514) -> (0:w1513:string)  [unwired: 1 in]
          n518 = Number To Hexadecimal String(2:w1480) -> (0:w1481:string)  [unwired: 1 in]
          n519 = Number To Hexadecimal String(2:w1484) -> (0:w1485:string)  [unwired: 1 in]
          n520 = Number To Hexadecimal String(2:w1487) -> (0:w1488:string)  [unwired: 1 in]
          n521 = Hexadecimal String To Number(string=w1507) -> (number=w1506:u32)  [unwired: 2 in, 1 out]
          n522 = To Double Precision Float(number=w1506) -> (double precision float=→"DC Current":dbl)
          n523 = Hexadecimal String To Number(string=w1491) -> (number=w1492:u32)  [unwired: 2 in, 1 out]
          n524 = Hexadecimal String To Number(string=w1513) -> (number=w1512:u32)  [unwired: 2 in, 1 out]
          n525 = Hexadecimal String To Number(string=w1481) -> (number=w1478:u32)  [unwired: 2 in, 1 out]
          n526 = Hexadecimal String To Number(string=w1485) -> (number=w1486:u32)  [unwired: 2 in, 1 out]
          n527 = Hexadecimal String To Number(string=w1488) -> (number=w1489:u32)  [unwired: 2 in, 1 out]
          n528 = To Double Precision Float(number=u32 10 ("y")) -> (double precision float=w1510:dbl)
          n529 = To Double Precision Float(number=w1512) -> (double precision float=w1509:dbl)
          n530 = To Double Precision Float(number=w1492) -> (double precision float=w1475:dbl)
          n531 = To Double Precision Float(number=w1486) -> (double precision float=w1471:dbl)
          n532 = To Double Precision Float(number=w1489) -> (double precision float=w1477:dbl)
          n533 = Divide(x=w1509, y=w1510) -> (x/y=→"DC Voltage":dbl)
          n534 = To Unsigned Word Integer(number=w1478) -> (unsigned 16bit integer=→"ECS State":u16)
          n535 = Subtract(x=w1475, y=50.0 ("x")) -> (x-y=w1463:dbl)
          n536 = Subtract(x=w1477, y=50.0 ("x")) -> (x-y=w1466:dbl)
          n537 = call "Filter (SubVI).vi"("Delta"=5000.0, "NewVal"=w1471, "OldVal"=w1470) -> ("Val"=w1468:dbl)  [unwired: 8 in]
          "Motor Speed RPM" <- w1468
          n538 = Less Than 0?(x=w1466) -> (x < 0?=w1473:bool)
          n539 = Less Than 0?(x=w1463) -> (x < 0?=w1472:bool)
          n540 = Select(t=w1464, s=w1473, f=w1466) -> (s? t:f=w1467:dbl)
          n541 = Select(t=w1458, s=w1472, f=w1463) -> (s? t:f=w1462:dbl)
          n542 = call "Filter (SubVI).vi"("Delta"=130.0, "NewVal"=w1467, "OldVal"=w1464) -> ("Val"=w1465:dbl)  [unwired: 8 in]
          "Motor Stator Temp." <- w1465
          n543 = call "Filter (SubVI).vi"("Delta"=100.0, "NewVal"=w1462, "OldVal"=w1458) -> ("Val"=w1459:dbl)  [unwired: 8 in]
          "Power transistor Heat sink Temp." <- w1459
        }
        frame 1 {
          # "Framde ID\n0x18E3273F"
          n544 = control-ref of="UUT"() -> (w1518:refnum<vi>)
          n545 = property on="Property Node" class="DigNum (strict)"(reference=w1518) -> ("Value"=w1519:u8)  [unwired: 1 in, 2 out]
          n546 = Index Array(array=w1528, index #1=0 ("index"), index #2=1 ("index")) -> (element #1=w1526:u8, element #2=w1521:u8)
          n547 = Number To Boolean Array(number=w1526) -> (Boolean array=w1525:bool[])
          n548 = Number To Boolean Array(number=w1521) -> (Boolean array=w1523:bool[])
          n549 = Boolean To (0,1)(Boolean=w1523) -> (0, 1=w1520:i16[])
          n550 = Boolean To (0,1)(Boolean=w1525) -> (0, 1=w1524:i16[])
          n551 = case shown="95" w1519 {
            tunnel: w1520 -> [_ w1529]
            frame 0, Default {
            }
            frame 95 {
              n552 = for {
                tunnel: w1529 -> [w1534] mode=indexing
                i -> [w1530]
                stop <- w1532 stop-if-true
                n553 = Not Equal To 0?(x=w1534) -> (x != 0?=w1533:bool)
                n554 = case shown="0, Default" w1530 {
                  tunnel: w1533 -> [w1535 w1536]
                  frame 0, Default {
                    "Ambient Sensor temp" <- w1535
                  }
                  frame 1 {
                    "Ambient Over temp" <- w1536
                  }
                }
                n555 = Equal?(x=w1530, y=1.0) -> (x = y?=w1532:bool)
              }
            }
          }
          n556 = for {
            tunnel: w1524 -> [w1538] mode=indexing
            i -> [w1539]
            n557 = Not Equal To 0?(x=w1538) -> (x != 0?=w1537:bool)
            n558 = case shown="5" w1539 {
              tunnel: w1537 -> [w1540 w1541 w1542 w1543 w1544 w1545 w1546 w1547]
              frame 0, Default {
                "Drive Sensor temp Failure" <- w1540
              }
              frame 1 {
                "Drive Over temperature" <- w1541
              }
              frame 2 {
                "Motor Sensor temp Fauilre" <- w1542
              }
              frame 3 {
                "Motor Over temperature" <- w1543
              }
              frame 4 {
                "Derated drive temp" <- w1544
              }
              frame 5 {
                "Under voltage/Over voltage" <- w1545
              }
              frame 6 {
                "Commutation err" <- w1546
              }
              frame 7 {
                "Speed error" <- w1547
              }
            }
          }
        }
        frame 2 {
          # "Frame ID\n0x18E2273F"
          n559 = Index Array(array=w1562, index #1=0 ("index"), index #2=1 ("index")) -> (element #1=w1559:u8, element #2=w1556:u8)
          n560 = disable-structure shown="Enabled" {
            disable-tunnel: [w1565 w1566] -> w1560
            disable-tunnel: w1559 -> [w1564 w1566]
            frame Disabled {
              n561 = Number To Hexadecimal String(2:w1564) -> (0:w1563:string)  [unwired: 1 in]
              n562 = Hexadecimal String To Number(string=w1563) -> (number=w1565:u32)  [unwired: 2 in, 1 out]
            }
            frame Enabled {
            }
          }
          n563 = Number To Hexadecimal String(2:w1556) -> (0:w1554:string)  [unwired: 1 in]
          n564 = Hexadecimal String To Number(string=w1554) -> (number=w1555:u32)  [unwired: 2 in, 1 out]
          n565 = To Double Precision Float(number=w1555) -> (double precision float=w1552:dbl)
          n566 = To Double Precision Float(number=w1560) -> (double precision float=→"Motor Phase Current RMS":dbl)
          n567 = Subtract(x=w1552, y=50.0) -> (x-y=→"Ambient Temperature":dbl)
        }
      }
    }
  }
  n568 = while {
    shift-right: [w1584] -> _
    shift-left: T10."Initialize" -> [w1583]
    shift-right: [w1579] -> _
    shift-left: "" -> [w1578]
    shift-right: [w1580] -> _
    shift-left: w6 -> [w1581]
    shift-right: [w1577] -> _
    shift-left: _ -> [w1576]
    shift-right: [w1575] -> _
    shift-left: w10 -> [w1573]
    shift-right: [w1574] -> _
    shift-left: refnum<vi> refnum ("Config_CANAT") -> [w1572]
    shift-right: [w1570] -> _
    shift-left: w5 -> [w1571]
    tunnel: "ATR" -> [_]
    stop <- w1582 stop-if-true
    n569 = case shown="\"MainProgram\"" w1583 {
      tunnel: [T10."MainProgram" T10."Stop" w1675 T10."Erase ATR Table"] -> w1584
      tunnel: [FALSE TRUE FALSE FALSE] -> w1582
      tunnel: [w1586 w1654 w1669 w2039] -> w1580
      tunnel: w1581 -> [_ w1641 w1673 _]
      tunnel: ["ATR Reset" "Program Stopped...\r\nPlease turn OFF All Power sinks" _ "Initialization State..."] -> w1579
      tunnel: [w1608 refnum<visa-resource-name> refnum ("VISA resource name") w1670 w2044] -> w1577
      tunnel: w1576 -> [w1608 w1651 w1671 _]
      tunnel: [w1595 refnum<queue> refnum ("queue out") w1665 w2037] -> w1575
      tunnel: [w1594 refnum<vi> refnum ("Config_CANAT") w1666 w2040] -> w1574
      tunnel: w1573 -> [w1595 w1655 w1668 w2037]
      tunnel: w1572 -> [w1594 _ w1667 _]
      tunnel: w1571 -> [w1593 w1645 w1664 w2036]
      tunnel: [w1593 refnum<queue> refnum ("queue out") w1663 w2036] -> w1570
      frame "Erase ATR Table", Default {
        w1589 = refnum<visa-resource-name> "COM4" ("VISA resource name")
        w1603 = FALSE ("Visible")
        n570 = property on="Serial Com" class="Bool"(error in=errorcluster {"status"=FALSE, "code"=0, "source"=""} ("error out"), "Visible"=TRUE) -> (error out=w1590:errorcluster)  [unwired: 1 in, 1 out]
        n571 = property on="VISA Marvin" class="VISAName"(error in=w1590, "Visible"=w1603, "Value"=w1589) -> (error out=w1605:errorcluster)  [unwired: 1 in, 1 out]
        n572 = property on="VISA Marvin" class="VISAName"(error in=w1590, "Value"=w1589) -> ()  [unwired: 1 in, 2 out]
        n573 = property on="Status" class="Bool (strict)"(error in=w1605, "Value"=w1603) -> (error out=w1598:errorcluster)  [unwired: 1 in, 1 out]
        n574 = flat-sequence {
          tunnel: [w1612] -> w1600
          tunnel: w1598 -> [w1610]
          tunnel: [w1610] -> w1597
          frame #0 {
            n575 = Two Button Dialog(message="Please seect the Unit Under Test.", 1:"AHU" ("F button name (\"Cancel\")"), 2:"EBAY" ("T button name (\"OK\")")) -> (T button?=w1612:bool)
          }
        }
        n576 = case shown="False" w1600 {
          tunnel: [string[][] [["6.1", "Visual Inspection", "", "", "", "", ""], ["6.1.1", "Verification of Components Not Installed", "N/A", "-", "", "", ""], ["", "", "", "", "", "", ""], ["6.1.2", "Manufacturing Defects", "N/A", "-", "", "", ""], ["", "", "", "", "", "", ""], ["6.2", "Power Supply Testing", "", "", "", "", ""], ["6.2.1", "Input Current Drawn", "", "", "", "", ""], ["6.2.1.1", "DC Input Current", "< 150", "-", "mA", "", ""], ["", "", "", "", "", "", ""], ["6.2.2", "Power Supply Voltages", "", "", "", "", ""], ["6.2.2.1", "12V", "12.0", "+/-0.500", "V", "", ""], ["6.2.2.2", "5V", "5.0", "+/-0.200", "V", "", ""], ["6.2.2.3", "3.3V", "3.3", "+/-0.100", "V", "", ""], ["6.2.2.4", "1.8V", "1.8", "+/-0.100", "V", "", ""], ["", "", "", "", "", "", ""], ["7", "Functional Test Procedure", "", "", "", "", ""], ["7.1", "Weight Check", "3800", "+/-100.0", "gr", "", ""], ["", "", "", "", "", "", ""], ["7.2", "Insulation Resistance Test", "", "", "", "", ""], ["7.2.1", "J3.B to Chassis", "> 1M", "-", "ohms", "", ""], ["7.2.2", "J1.16 to Chassis", "> 100K", "-", "ohms", "", ""], ["", "", "", "", "", "", ""], ["7.2", "Bonding Resistance", "", "", "", "", ""], ["7.2.3", "J1 Body to Chassis", "< 2m", "-", "ohms", "", ""], ["7.2.4", "J2  Body to Chassis", "< 2m", "-", "ohms", "", ""], ["7.2.5", "J3  Body to Chassis", "< 2m", "-", "ohms", "", ""], ["", "", "", "", "", "", ""], ["7.2.1", "CANbus Resistance Test", "", "", "", "", ""], ["7.2.1.1", "J1.17 to J1.18", "> 10K", "-", "ohms", "", ""], ["", "", "", "", "", "", ""], ["7.3", "Sealing Test", "N/A", "-", "", "", ""], ["", "", "", "", "", "", ""], ["7.4", "Communication Test", "", "", "", "", ""], ["7.4.1", "Serial RS-232", "N/A", "-", "", "", ""], ["7.4.2", "CAN Bus", "N/A", "-", "", "", ""], ["", "", "", "", "", "", ""], ["7.5", "Performances Tests", "", "", "", "", ""], ["7.5.1", "Reverse Polarity Test", "", "", "", "", ""], ["7.5.1.1", "DC Input Current", "< 1", "-", "mA", "", ""], ["", "", "", "", "", "", ""], ["7.5.2", "Enable Test", "", "", "", "", ""], ["7.5.2.1", "Fan Speed at Opened Enable ", "6000", "+/-200.0", "rpm", "", ""], ["7.5.2.2", "Fan Speed at Opened Enable ", "0", "+/-200.0", "rpm", "", ""], ["7.5.2.3", "Fan Speed at Closed Enable ", "6000", "+/-200.0", "rpm", "", ""], ["7.5.2.4", "Motor Rotation Direction", "Counter-clockwise (Inlet)", "-", "", "", ""], ["", "", "", "", "", "", ""], ["7.5.3", "Stop Time Test ", "", "", "", "", ""], ["7.5.3.1", "Motor Stop time", "< 50", "-", "sec", "", ""], ["", "", "", "", "", "", ""], ["7.5.4", "Speed Command Test", "", "", "", "", ""], ["7.5.4.1", "Fan Speed", "6000", "+/-200.0", "rpm", "", ""], ["7.5.4.2", "Fan Speed", "9000", "+/-200.0", "rpm", "", ""], ["7.5.4.3", "Fan Speed", "12100", "+/-200.0", "rpm", "", ""], ["", "", "", "", "", "", ""], ["7.5.5", "Temperature Sensor Calibration Test", "", "", "", "", ""], ["7.5.5.1", "Sensor Reading Analog Offset", "0", "+/-0.100", ".", "", ""], ["", "", "", "", "", "", ""], ["7.5.6", "Burn-in Test", "", "", "", "", ""], ["7.5.6.1", "DC Input Current", "28", "+/-5.000", "A", "", ""], ["7.5.6.2", "Ambient Temperature", "25", "+/-13.00", "Deg.", "", ""], ["7.5.6.3", "After 10 min of operation", "", "", "Deg.", "", ""], ["7.5.6.4", "After 20 min of operation", "", "", "Deg.", "", ""], ["7.5.6.5", "After 30 min of operation", "", "", "Deg.", "", ""], ["", "", "", "", "", "", ""], ["8", "Auxiliary", "", "", "", "", ""], ["8.1", "Auxiliary Cooling Fan 60 Deg", "On", "-", ".", "", ""], ["8.2", "Auxiliary Cooling Fan 55 Deg", "Off", "-", ".", "", ""]] ("data") string[][] [["6.1", "Visual Inspection", "", "", "", "", ""], ["6.1.1", "Verification of Components Not Installed", "N/A", "-", "", "", ""], ["", "", "", "", "", "", ""], ["6.1.2", "Manufacturing Defects", "N/A", "-", "", "", ""], ["", "", "", "", "", "", ""], ["6.2", "Power Supply Testing", "", "", "", "", ""], ["6.2.1", "Input Current Drawn", "", "", "", "", ""], ["6.2.1.1", "DC Input Current", "< 150", "-", "mA", "", ""], ["", "", "", "", "", "", ""], ["6.2.2", "Power Supply Voltages", "", "", "", "", ""], ["6.2.2.1", "12V", "12.0", "+/-0.500", "V", "", ""], ["6.2.2.2", "5V", "5.0", "+/-0.200", "V", "", ""], ["6.2.2.3", "3.3V", "3.3", "+/-0.100", "V", "", ""], ["6.2.2.4", "1.8V", "1.8", "+/-0.100", "V", "", ""], ["", "", "", "", "", "", ""], ["7", "Functional Test Procedure", "", "", "", "", ""], ["7.1", "Weight Check", "4180", "+/-10.00", "gr", "", ""], ["", "", "", "", "", "", ""], ["7.2", "Insulation Resistance Test", "", "", "", "", ""], ["7.2.1", "J3.B to Chassis", "> 1M", "-", "ohms", "", ""], ["7.2.2", "J1.16 to Chassis", "> 100K", "-", "ohms", "", ""], ["", "", "", "", "", "", ""], ["7.2", "Bonding Resistance", "", "", "", "", ""], ["7.2.3", "J1 Body to Chassis", "< 2m", "-", "ohms", "", ""], ["7.2.4", "J2  Body to Chassis", "< 2m", "-", "ohms", "", ""], ["7.2.5", "J3  Body to Chassis", "< 2m", "-", "ohms", "", ""], ["", "", "", "", "", "", ""], ["7.2.1", "CANbus Resistance Test", "", "", "", "", ""], ["7.2.1.1", "J1.17 to J1.18", "> 10K", "-", "ohms", "", ""], ["", "", "", "", "", "", ""], ["7.3", "Sealing Test", "N/A", "-", "", "", ""], ["", "", "", "", "", "", ""], ["7.4", "Communication Test", "", "", "", "", ""], ["7.4.1", "Serial RS-232", "N/A", "-", "", "", ""], ["7.4.2", "CAN Bus", "N/A", "-", "", "", ""], ["", "", "", "", "", "", ""], ["7.5", "Performances Tests", "", "", "", "", ""], ["7.5.1", "Reverse Polarity Test", "", "", "", "", ""], ["7.5.1.1", "DC Input Current", "< 1", "-", "mA", "", ""], ["", "", "", "", "", "", ""], ["7.5.2", "Enable Test", "", "", "", "", ""], ["7.5.2.1", "Fan Speed at Opened Enable ", "6000", "+/-200.0", "rpm", "", ""], ["7.5.2.2", "Fan Speed at Opened Enable ", "0", "+/-200.0", "rpm", "", ""], ["7.5.2.3", "Fan Speed at Closed Enable ", "6000", "+/-200.0", "rpm", "", ""], ["7.5.2.4", "Motor Rotation Direction", "Counter-clockwise (Inlet)", "-", "", "", ""], ["", "", "", "", "", "", ""], ["7.5.3", "Stop Time Test ", "", "", "", "", ""], ["7.5.3.1", "Motor Stop time", "< 50", "-", "sec", "", ""], ["", "", "", "", "", "", ""], ["7.5.4", "Speed Command Test", "", "", "", "", ""], ["7.5.4.1", "Fan Speed", "6000", "+/-200.0", "rpm", "", ""], ["7.5.4.2", "Fan Speed", "11500", "+/-200.0", "rpm", "", ""], ["7.5.4.3", "Fan Speed", "15100", "+/-200.0", "rpm", "", ""], ["", "", "", "", "", "", ""], ["7.5.5", "Temperature Sensor Calibration Test", "", "", "", "", ""], ["7.5.5.1", "Sensor Reading Analog Offset", "0", "+/-0.100", ".", "", ""], ["", "", "", "", "", "", ""], ["7.5.6", "Temperature Control Algorithm Test", "", "", "", "", ""], ["7.5.6.1", "Tair <   68 ± 2 oC", "6000", "+/-200.0", "rpm", "", ""], ["7.5.6.2", "Measured Temp.", "", "", "Deg.", "", ""], ["7.5.6.3", "Tair >= 68 ± 2 oC", "11500", "+/-200.0", "rpm", "", ""], ["7.5.6.4", "Transition Temp.", "", "", "Deg.", "", ""], ["7.5.6.5", "Tair >= 88 ± 2 oC", "15100", "+/-400.0", "rpm", "", ""], ["7.5.6.6", "Transition Temp.", "", "", "Deg.", "", ""], ["7.5.6.7", "Tair <= 80 ± 2 oC", "11500", "+/-200.0", "rpm", "", ""], ["7.5.6.8", "Transition Temp.", "", "", "Deg.", "", ""], ["7.5.6.9", "Tair <= 60 ± 2 oC", "6000", "+/-200.0", "rpm", "", ""], ["7.5.6.10", "Transition Temp.", "", "", "Deg.", "", ""], ["", "", "", "", "", "", ""], ["7.5.7", "Burn-in Test", "", "", "", "", ""], ["7.5.7.1", "DC Input Current", "50", "+/-5.000", "A", "", ""], ["7.5.7.2", "Fan Speed", "15100", "+/-400.0", "rpm", "", ""], ["7.5.7.3", "Ambient Temperature", "25", "+/-13.00", "Deg.", "", ""], ["7.5.7.4", "After 10 min of operation", "", "-", "Deg.", "", ""], ["7.5.7.5", "After 20 min of operation", "", "-", "Deg.", "", ""], ["7.5.7.6", "After 30 min of operation", "", "-", "Deg.", "", ""], ["", "", "", "", "", "", ""], ["8", "Auxiliary", "", "", "", "", ""], ["8.1", "Auxiliary Cooling Fan ON", "60", "+/-2.00", "Deg.", "", ""], ["8.2", "Fan status", "ON", "-", "-", "", ""], ["8.3", "Auxiliary Cooling Fan OFF", "55", "+/-2.00", "Deg.", "", ""], ["8.4", "Fan status", "OFF", "-", "-", "", ""], ["", "", "", "", "", "", ""], ["9", "Motor Temp. Test", "", "", "", "", ""], ["9.1", "60 Degree", "60", "+/-3.00", "C", "", ""], ["9.2", "90 Degree", "90", "+/-3.00", "C", "", ""], ["9.3", "120 Degree", "120", "+/-3.00", "C", "", ""]] ("data")] -> w1601
          tunnel: ["AHU" "EBAY"] -> w1599
          tunnel: [w1615 w1618] -> w1596
          tunnel: w1597 -> [w1615 w1618]
          frame False {
          }
          frame True {
          }
        }
        "UUT" <- w1599
        n577 = for {
          tunnel: w1601 -> [w1625] mode=indexing
          tunnel: w1596 -> [w1623]
          tunnel: [w1622] -> w1592
          tunnel: w1601 -> [w1621]
          i -> [w1624]
          n578 = for {
            tunnel: w1625 -> [_] mode=indexing
            tunnel: w1624 -> [w1631]
            tunnel: w1623 -> [w1628]
            tunnel: [w1627] -> w1622
            tunnel: w1621 -> [w1626]
            i -> [w1632]
            n579 = Bundle By Name(cluster=T18 {"Row"=0, "Column"=0} ("Active Cell:Active Cell"), "Row"=w1631, "Column"=w1632) -> (w1630:T18)
            n580 = control-ref of="ATR"() -> (w1629:refnum<vi>)
            n581 = property class="Tbl (strict)"(reference=w1629, error in=w1628, "Active Cell"=w1630, "Cell BG Color"=u32 16777226, "Value"=w1626) -> (error out=w1627:errorcluster)  [unwired: 1 out]
          }
        }
        n582 = call "COM EvolutionBoard.vi"("error in (no error)"=w1592, "VISA resource name 2"=refnum<visa-resource-name> "COM1" ("VISA resource name")) -> ("error out"=w1586:errorcluster, "VISA resource name out"=w1585:refnum<visa-resource-name>)  [unwired: 8 in]
        "VISA Tester" <- w1585
        n583 = Byte Array To String(unsigned byte array=u8[] [75, 0, 4, 2, 0, 0, 2, 0] ("appended array")) -> (string=w1588:string)
        n584 = VISA Write(VISA resource name=w1585, write buffer=w1588, error in (no error)=w1586) -> ()  [unwired: 3 out]
      }
      frame "Stop" {
        n585 = flat-sequence {
          tunnel: w1641 -> [w1660]
          tunnel: [w1659] -> w1640
          frame #0 {
            n586 = control-ref of="Pannel User Message"() -> (w1662:refnum<vi>)
            n587 = property class="Str"(reference=w1662, error in=w1660, "Value"="Program Stopped...\r\nPlease turn OFF All Power sinks") -> (error out=w1659:errorcluster)  [unwired: 1 out]
          }
        }
        n588 = control-ref of="VISA Tester"() -> (w1643:refnum<vi>)
        n589 = property class="VISAName"(reference=w1643, error in=w1640) -> ("Value"=w1639:refnum<visa-resource-name>)  [unwired: 2 out]
        n590 = VISA Close(VISA resource name=w1651, error in (no error)=w1640) -> (error out=w1644:errorcluster)
        n591 = call "TesterOption (SubVI).vi"("2 Options"=FALSE, "On/Off"=FALSE, "Tester Option"=T11."Power", "VISA Refnum in"=w1639) -> ("VISA Refnum out"=w1638:refnum<visa-resource-name>)  [unwired: 6 in, 1 out]
        n592 = VISA Close(VISA resource name=w1638) -> ()  [unwired: 1 in, 1 out]
        n593 = Flush Queue(queue=w1645, error in (no error)=w1644) -> (queue out=w1647:refnum<queue>, error out=w1646:errorcluster)  [unwired: 1 out]
        n594 = Flush Queue(queue=w1655, error in (no error)=w1644) -> (queue out=w1652:refnum<queue>, error out=w1656:errorcluster)  [unwired: 1 out]
        n595 = Release Queue(queue=w1647, error in (no error)=w1646) -> ()  [unwired: 1 in, 3 out]
        n596 = Release Queue(queue=w1652, error in (no error)=w1656) -> (error out=w1654:errorcluster)  [unwired: 1 in, 2 out]
      }
      frame "MainProgram" {
        (unwired) "Main Program..."
        n597 = event shown="[9] \"VISA Marvin\": Value Change" {
          selector: _ -> [_ _ _ _ _ _ _ _ _ _ _ _]
          dyn-events: _ -> [_ _ _ _ _ _ _ _ _ _ _ _]
          timeout: 50 -> [_ _ _ _ _ _ _ _ _ _ _ _]
          tunnel: [T10."MainProgram" T10."MainProgram" T10."MainProgram" T10."MainProgram" T10."Stop" T10."MainProgram" T10."MainProgram" T10."MainProgram" T10."MainProgram" T10."MainProgram" w2006 T10."MainProgram"] -> w1675
          tunnel: [w1676 w1743 w1749 w1757 w1771 w1774 w1930 w1944 w1956 w1961 w2011 w2020] -> w1669
          tunnel: w1673 -> [w1681 w1742 w1751 w1757 w1771 w1783 w1930 w1945 w1955 w1960 w2011 w2024]
          tunnel: [w1690 w1744 w1750 w1758 w1769 w1777 w1929 w1942 w1953 w1965 w2004 w2017] -> w1670
          tunnel: w1671 -> [w1690 w1744 w1750 w1758 w1769 w1777 w1929 w1942 w1953 _ w2004 w2017]
          tunnel: w1668 -> [w1683 w1738 w1746 w1754 w1768 w1780 w1894 w1941 w1952 w1969 w2003 w2016]
          tunnel: w1667 -> [w1677 w1739 w1747 w1755 w1767 w1781 w1893 w1940 w1951 w1968 w2002 w2015]
          tunnel: [w1679 w1739 w1747 w1755 w1767 w1781 w1893 w1940 w1951 w1968 w2002 w2015] -> w1666
          tunnel: [w1682 w1738 w1746 w1754 w1768 w1780 w1894 w1941 w1952 w1969 w2003 w2016] -> w1665
          tunnel: w1664 -> [w1680 w1737 w1745 w1753 w1766 w1779 w1892 w1939 w1950 w1967 w2001 w2014]
          tunnel: [w1680 w1737 w1745 w1753 w1766 w1773 w1892 w1939 w1950 w1967 w2001 w2014] -> w1663
          event Timeout {
            n598 = event-data() -> ()  [unwired: 1 in, 3 out]
            n599 = property class="Clust (strict)"(reference=w1677, error in=w1681) -> (reference out=w1679:refnum<vi>, error out=w1678:errorcluster, "Value"=w1687:T7)
            n600 = Unbundle By Name(w1687) -> ("DevType"=w1688:T2, "CanIndex"=w1685:T1)
            n601 = call "VCI_Receive.vi"("CANIndex"=w1685, "DevIndex"=u32 0, "DevType"=w1688) -> ("Recieve"=w1684:T23[])  [unwired: 3 in, 5 out]
            n602 = Empty Array?(array=w1684) -> (empty?=w1686:bool)
            n603 = case shown="False" w1686 {
              tunnel: w1685 -> [w1703 _]
              tunnel: w1679 -> [w1701 _]
              tunnel: w1683 -> [w1700 w1736]
              tunnel: w1678 -> [w1699 w1735]
              tunnel: w1684 -> [w1704 _]
              tunnel: [w1694 w1735] -> w1676
              tunnel: [w1693 w1736] -> w1682
              tunnel: [w1692 0] -> _
              frame False {
                n604 = call "Demo_MakeDispBuff.vi"("Channel"=w1703, "Type"=enum16{"接收", "发送"}."接收", "OBJs"=w1704) -> ("Buffer"=w1702:T24)
                n605 = for {
                  N: 3 -> [_]
                  tunnel: w1702 -> [w1718]
                  tunnel: w1701 -> [w1717]
                  tunnel: w1700 -> [w1708]
                  tunnel: w1699 -> [w1707]
                  tunnel: [w1710] -> w1697 mode=indexing
                  tunnel: [w1708] -> w1696
                  tunnel: [w1707] -> w1695
                  tunnel: [w1706] -> w1692
                  i -> [w1706]
                  n606 = property class="Clust (strict)"(reference=w1717) -> ("Value"=w1715:T7)  [unwired: 1 in, 2 out]
                  n607 = Index Array(array=w1718, index=w1706) -> (element=w1711:T25)
                  n608 = Unbundle By Name(w1711) -> ("Channel"=w1713:T1, "VCI_CAN_OBJ"=w1716:T23)  [unwired: 2 out]
                  n609 = Unbundle By Name(w1715) -> ("CanIndex"=w1714:T1)
                  n610 = Equal?(x=w1714, y=w1713) -> (x = y?=w1712:bool)
                  n611 = case shown="True" w1712 {
                    tunnel: w1716 -> [_ w1729]
                    tunnel: [w1719 w1725] -> w1710
                    tunnel: T19 {"ID"=0, "MSGTYPE"=0, "LEN"=0, "aDATA"=[]} ("Msg") -> [w1719 w1724]
                    frame False {
                    }
                    frame True {
                      n612 = Unbundle By Name(w1729) -> ("ID"=w1723:u32, "DataLen"=w1728:u8, "Data"=w1726:u8[])
                      n613 = Bundle By Name(cluster=w1724, "ID"=w1723, "MSGTYPE"=u8 0, "LEN"=w1728, "aDATA"=w1726) -> (w1725:T19)
                      n614 = Unbundle By Name(w1725) -> ("ID"=w1721:u32)
                      n615 = Split Number(x=w1721) -> (lo(x)=w1722:u16)  [unwired: 1 out]
                      n616 = Split Number(x=w1722) -> (lo(x)=w1720:u8)  [unwired: 1 out]
                      "UUT" <- w1720
                      n617 = case shown="63" w1720 {
                        tunnel: ["EBAY 5F" "" "AHU 3F" "AHU 2F"] -> _
                        frame 95 {
                        }
                        frame Default {
                        }
                        frame 63 {
                        }
                        frame 47 {
                        }
                      }
                    }
                  }
                }
                n618 = Enqueue Element(queue=w1696, element=w1697, error in (no error)=w1695) -> (queue out=w1693:refnum<queue>, error out=w1694:errorcluster)  [unwired: 2 out]
              }
              frame True {
              }
            }
          }
          event "ATR": Mouse Enter {
            n619 = event-data() -> ()  [unwired: 1 in, 4 out]
            n620 = call-poly <vilib>:"Set Cursor.vi"("error in (no error)"=w1742, "icon"=u16 1) -> ("error out"=w1743:errorcluster)  [unwired: 8 in, 1 out]
          }
          event "ATR": Mouse Leave {
            n621 = event-data() -> ()  [unwired: 1 in, 4 out]
            n622 = call-poly <vilib>:"Set Cursor.vi"("error in (no error)"=w1751, "icon"=u16 0) -> ("error out"=w1749:errorcluster)  [unwired: 8 in, 1 out]
          }
          event "ATR": Mouse Down? {
            n623 = event-data() -> ("Coords"=w1765:T26)  [unwired: 1 in, 4 out]
            n624 = invoke on="ATR" class="Tbl (strict)" method="Point To Row Column"("Point"=w1765) -> ("InBounds"=w1761:bool, "CellPosition"=w1760:T18)  [unwired: 5 in, 4 out]
            n625 = Greater Than 0?(x=w1760) -> (x > 0?=w1764:cluster{"Row":bool, "Column":bool})
            n626 = Cluster To Array(cluster=w1764) -> (array=w1763:bool[])
            n627 = Or Array Elements(Boolean array=w1763) -> (logical OR=w1762:bool)
            n628 = Or(x=w1761, y=w1762) -> (x .or. y?=w1759:bool)
            n629 = event-data("Discard?"=w1759) -> ()  [unwired: 1 in, 1 out]
          }
          event "Stop Button": Value Change {
            n630 = event-data() -> ()  [unwired: 1 in, 6 out]
          }
          event "Start": Value Change {
            n631 = event-data() -> ()  [unwired: 1 in, 2 out]
            n632 = property on="UUT" class="Str"(error in=w1783) -> ("Value"=w1782:string)  [unwired: 1 in, 2 out]
            n633 = case shown="\"AHU\", Default" w1782 {
              tunnel: [w1797 w1849] -> w1776
              tunnel: [w1796 w1848] -> w1775
              frame "AHU", Default {
                n634 = call "Load Program Process AHU.vi"() -> ("Speed Command Test"=w1789:bool, "Enable Test"=w1790:bool, "Burn-in Test"=w1787:bool, "Auxiliary"=w1785:bool, "Temperature Sensor Calibration Test"=w1792:bool, "Communication Test"=w1791:bool, "Stop Time Test"=w1788:bool, "Visual Inspection"=w1786:bool, "OK"=w1794:bool, "Automation"=w1793:bool, "error out"=w1796:errorcluster)  [unwired: 8 in, 9 out]
                n635 = Or(x=w1794, y=w1793) -> (x .or. y?=w1795:bool)
                n636 = case shown="True" w1795 {
                  tunnel: [w1798 w1808] -> w1797
                  tunnel: w1793 -> [_ w1807]
                  tunnel: w1792 -> [_ w1806]
                  tunnel: w1791 -> [_ w1805]
                  tunnel: w1790 -> [_ w1804]
                  tunnel: w1789 -> [_ w1803]
                  tunnel: w1788 -> [_ w1802]
                  tunnel: w1787 -> [_ w1801]
                  tunnel: w1786 -> [_ w1800]
                  tunnel: w1785 -> [_ w1799]
                  frame False {
                    w1798 = T27 [] items=["Visual Inspection", "Temp Sens Cal", "Com Test", "Enable Test", "Speed Command", "Stop Time", "Temp Control", "Burn in", "Visual Inspec", "Empty"]
                  }
                  frame True {
                    n637 = case shown="False" w1807 {
                      tunnel: [w1834 w1835] -> w1808
                      tunnel: w1806 -> [w1826 _]
                      tunnel: w1805 -> [w1825 _]
                      tunnel: w1804 -> [w1824 _]
                      tunnel: w1803 -> [w1823 _]
                      tunnel: w1802 -> [w1822 _]
                      tunnel: w1801 -> [w1821 _]
                      tunnel: w1800 -> [w1820 _]
                      tunnel: w1799 -> [w1812 _]
                      frame False {
                        w1811 = T20."Empty" ("f")
                        n638 = Select(t=T20."Temp Sens Cal" ("f"), s=w1826, f=w1811) -> (s? t:f=w1819:T20)
                        n639 = Select(t=T20."Com Test" ("f"), s=w1825, f=w1811) -> (s? t:f=w1818:T20)
                        n640 = Select(t=T20."Enable Test" ("f"), s=w1824, f=w1811) -> (s? t:f=w1817:T20)
                        n641 = Select(t=T20."Speed Command" ("f"), s=w1823, f=w1811) -> (s? t:f=w1816:T20)
                        n642 = Select(t=T20."Stop Time" ("f"), s=w1822, f=w1811) -> (s? t:f=w1815:T20)
                        n643 = Select(t=T20."Burn in" ("f"), s=w1821, f=w1811) -> (s? t:f=w1814:T20)
                        n644 = Select(t=T20."Auxiliary" ("f"), s=w1812, f=w1811) -> (s? t:f=w1809:T20)
                        n645 = Select(t=T20."Visual Inspec" ("f"), s=w1820, f=w1811) -> (s? t:f=w1813:T20)
                        n646 = Build Array(w1819, w1818, w1817, w1816, w1815, w1814, w1809, w1813) -> (w1834:T16)
                      }
                      frame True {
                        w1835 = T28 [enum."Temp Sens Cal", enum."Com Test", enum."Enable Test", enum."Speed Command", enum."Stop Time", enum."Burn in", enum."Auxiliary", enum."Visual Inspec"] items=["Auxiliary", "Temp Sens Cal", "Com Test", "Enable Test", "Speed Command", "Stop Time", "Burn in", "Visual Inspec", "Empty"]
                      }
                    }
                  }
                }
              }
              frame "EBAY" {
                n647 = call "Load Program Process EBAY.vi"() -> ("Speed Command Test"=w1841:bool, "Enable Test"=w1842:bool, "Burn-in Test"=w1839:bool, "Temperature Control Algorithm Test"=w1838:bool, "Auxiliary"=w1836:bool, "Temperature Sensor Calibration Test"=w1844:bool, "Communication Test"=w1843:bool, "Stop Time Test"=w1840:bool, "Visual Inspection"=w1837:bool, "OK"=w1846:bool, "Automation"=w1845:bool, "error out"=w1848:errorcluster)  [unwired: 8 in, 8 out]
                n648 = Or(x=w1846, y=w1845) -> (x .or. y?=w1847:bool)
                n649 = case shown="True" w1847 {
                  tunnel: [w1850 w1861] -> w1849
                  tunnel: w1845 -> [_ w1860]
                  tunnel: w1844 -> [_ w1859]
                  tunnel: w1843 -> [_ w1858]
                  tunnel: w1842 -> [_ w1857]
                  tunnel: w1841 -> [_ w1856]
                  tunnel: w1840 -> [_ w1855]
                  tunnel: w1839 -> [_ w1854]
                  tunnel: w1838 -> [_ w1853]
                  tunnel: w1837 -> [_ w1852]
                  tunnel: w1836 -> [_ w1851]
                  frame False {
                    w1850 = T16 [] items=["Auxiliary", "Temp Sens Cal", "Com Test", "Enable Test", "Speed Command", "Stop Time", "Temp Control", "Burn in", "Visual Inspec", "Empty"]
                  }
                  frame True {
                    n650 = case shown="False" w1860 {
                      tunnel: [w1890 w1891] -> w1861
                      tunnel: w1859 -> [w1881 _]
                      tunnel: w1858 -> [w1880 _]
                      tunnel: w1857 -> [w1879 _]
                      tunnel: w1856 -> [w1878 _]
                      tunnel: w1855 -> [w1877 _]
                      tunnel: w1854 -> [w1863 _]
                      tunnel: w1853 -> [w1862 _]
                      tunnel: w1852 -> [w1876 _]
                      tunnel: w1851 -> [w1867 _]
                      frame False {
                        w1865 = T20."Empty" ("f")
                        n651 = Select(t=T20."Temp Sens Cal" ("f"), s=w1881, f=w1865) -> (s? t:f=w1875:T20)
                        n652 = Select(t=T20."Com Test" ("f"), s=w1880, f=w1865) -> (s? t:f=w1874:T20)
                        n653 = Select(t=T20."Enable Test" ("f"), s=w1879, f=w1865) -> (s? t:f=w1873:T20)
                        n654 = Select(t=T20."Speed Command" ("f"), s=w1878, f=w1865) -> (s? t:f=w1872:T20)
                        n655 = Select(t=T20."Stop Time" ("f"), s=w1877, f=w1865) -> (s? t:f=w1871:T20)
                        n656 = Select(t=T20."Temp Control" ("f"), s=w1862, f=w1865) -> (s? t:f=w1870:T20)
                        n657 = Select(t=T20."Burn in" ("f"), s=w1863, f=w1865) -> (s? t:f=w1869:T20)
                        n658 = Select(t=T20."Visual Inspec" ("f"), s=w1876, f=w1865) -> (s? t:f=w1868:T20)
                        n659 = Select(t=T20."Auxiliary" ("f"), s=w1867, f=w1865) -> (s? t:f=w1864:T20)
                        n660 = Build Array(w1875, w1874, w1873, w1872, w1871, w1870, w1869, w1864, w1868) -> (w1890:T16)
                      }
                      frame True {
                        w1891 = T16 [enum."Temp Sens Cal", enum."Com Test", enum."Enable Test", enum."Speed Command", enum."Stop Time", enum."Temp Control", enum."Burn in", enum."Auxiliary", enum."Visual Inspec"] items=["Auxiliary", "Temp Sens Cal", "Com Test", "Enable Test", "Speed Command", "Stop Time", "Temp Control", "Burn in", "Visual Inspec", "Empty"]
                      }
                    }
                  }
                }
              }
            }
            n661 = Bundle By Name(cluster=T8 {"VISA"="COM1", "Array Test"=[]}, "VISA"=w1777, "Array Test"=w1776) -> (w1772:T8)
            n662 = Enqueue Element(queue=w1779, element=w1772, error in (no error)=w1775) -> (queue out=w1773:refnum<queue>, error out=w1774:errorcluster)  [unwired: 2 out]
          }
          event "Report": Value Change {
            n663 = event-data() -> ()  [unwired: 1 in, 6 out]
            n664 = call <vilib>:"Application Directory.vi"() -> ("Application Directory"=w1908:path)
            n665 = Build Path(base path=w1908, name or relative path="Reports") -> (appended path=w1911:path)
            n666 = local read "UUT"() -> (w1895:string)
            n667 = call <vilib>:"Check if File or Folder Exists.vi"("path"=w1911) -> ("error out"=w1909:errorcluster, "file or folder exists?"=w1912:bool, "dup path"=w1910:path)  [unwired: 8 in]
            n668 = control-ref of="ATR"() -> (w1926:refnum<vi>)
            n669 = case shown="False" w1912 {
              tunnel: w1909 -> [w1936 w1937]
              tunnel: w1910 -> [w1935 w1938]
              tunnel: [w1934 w1938] -> w1924
              tunnel: [w1933 w1937] -> w1918
              frame False {
                n670 = Create Folder(path (use dialog)=w1935, error in=w1936) -> (created path=w1934:path, error out=w1933:errorcluster)  [unwired: 1 in, 1 out]
              }
              frame True {
              }
            }
            n671 = Get Date/Time String(want seconds? (F)=TRUE) -> (date string=w1916:string, time string=w1915:string)  [unwired: 2 in]
            n672 = property on="Logger Path" class="Path"(error in=w1918, "Value"=w1924, "StartPath"=w1924) -> (error out=w1919:errorcluster)  [unwired: 1 in, 1 out]
            n673 = Search and Replace String(replace all?=TRUE ("replace all? (F)"), input string=w1916, search string="/") -> (result string=w1914:string)  [unwired: 5 in, 3 out]
            n674 = Search and Replace String(replace all?=TRUE ("replace all? (F)"), input string=w1915, search string=":") -> (result string=w1913:string)  [unwired: 5 in, 3 out]
            n675 = call "HeaderuRayon.vi"("UUT"=w1895) -> ("HEADER1"=w1925:string)  [unwired: 2 in]
            n676 = call <vilib>:"Space Constant.vi"() -> ("String"=w1896:string)
            n677 = Concatenate Strings(w1914, w1896, w1913, w1896, w1895, w1896, "Report.docx" ("string")) -> (w1898:string)
            n678 = property on="Logger Path" class="Path"(error in=w1919) -> (error out=w1920:errorcluster, "StartPath"=w1917:path)  [unwired: 1 in, 1 out]
            n679 = Build Path(base path=w1917, name or relative path=w1898) -> (appended path=w1899:path)
            n680 = call <vilib>:"Check if File or Folder Exists.vi"("error in (no error)"=w1920, "path"=w1899) -> ("error out"=w1921:errorcluster, "file or folder exists?"=w1922:bool)  [unwired: 7 in, 1 out]
            n681 = case shown="True" w1922 {
              tunnel: [T21."create" ("operation (0:open)") T21."replace" ("operation (0:open)")] -> w1923
              frame False {
              }
              frame True {
              }
            }
            n682 = Open/Create/Replace File(file path (use dialog)=w1899, error in=w1921, operation (0:open)=w1923) -> (error out=w1900:errorcluster)  [unwired: 3 in, 2 out]
            n683 = property class="Tbl (strict)"(reference=w1926, error in=w1900) -> ("Value"=w1927:string[][])  [unwired: 2 out]
            n684 = call "MarvinReport.vi"("HEADER1"=w1925, "ATR Or"=w1926, "Steps   pfull"=w1927, "pageNum"=3, "FILE NAME"=w1898, "Report Folder"=w1899) -> ()  [unwired: 8 in, 2 out]
          }
          event "Help Button": Value Change {
            n685 = event-data() -> ()  [unwired: 1 in, 6 out]
            n686 = vi-ref "Help.vi"() -> (w1947:refnum<vi>)
            n687 = invoke class="VI" method="FP.Open"(reference=w1947, error in=w1945, "Activate"=TRUE ("Activate?"), "State"=T22."Standard") -> (error out=w1946:errorcluster)  [unwired: 1 in, 4 out]
            n688 = call "Help.vi"("error in"=w1946) -> ("error out"=w1944:errorcluster)  [unwired: 7 in]
          }
          event "Serial Com": Value Change {
            n689 = event-data() -> ()  [unwired: 1 in, 6 out]
            n690 = property on="Serial Com" class="Bool"(error in=w1955, "Visible"=FALSE) -> (error out=w1959:errorcluster)  [unwired: 1 in, 1 out]
            n691 = property on="VISA Marvin" class="VISAName"(error in=w1959, "Visible"=TRUE) -> (error out=w1956:errorcluster)  [unwired: 1 in, 1 out]
          }
          event "VISA Marvin": Value Change {
            n692 = event-data() -> ()  [unwired: 1 in, 6 out]
            n693 = control-ref of="This VI"() -> (w1974:refnum<vi>)
            n694 = property on="Pannel User Message" class="Str"(error in=w1960, "Value"="Serial conection in process" ("Pannel User Message")) -> ()  [unwired: 1 in, 2 out]
            n695 = call "Serial InitMarvin.vi"("error in (no error)"=w1960, "VI reference (current VI)"=w1974, "VISA Refnum in"="VISA Marvin") -> ("error out"=w1981:errorcluster, "Boolean"=w1966:bool)  [unwired: 7 in]
            n696 = property on="Status" class="Bool (strict)"(error in=w1981, "Value"=w1966) -> (error out=w1978:errorcluster)  [unwired: 1 in, 1 out]
            n697 = property on="VISA Marvin" class="VISAName"(error in=w1978, "Visible"=FALSE) -> (error out=w1977:errorcluster)  [unwired: 1 in, 1 out]
            n698 = property on="Serial Com" class="Bool"(error in=w1977, "Visible"=TRUE) -> (error out=w1973:errorcluster)  [unwired: 1 in, 1 out]
            n699 = call "Serial.vi"("error in (no error)"=w1973, "Clear Log"=FALSE, "VISA resource name"="VISA Marvin") -> ("error out"=w1972:errorcluster)  [unwired: 7 in, 1 out]
            n700 = call <vilib>:"Clear Errors.vi"("error in (no error)"=w1972) -> ("error out"=w1982:errorcluster)  [unwired: 5 in, 1 out]
            n701 = case shown="True" w1966 {
              tunnel: w1982 -> [w1996 w2000]
              tunnel: [w1996 w1999] -> w1964
              tunnel: "VISA Marvin" -> [w1995 w1998]
              tunnel: [w1995 w1997] -> w1965
              frame False {
              }
              frame True {
                n702 = VISA Flush I/O Buffer(VISA resource name=w1998, error in (no error)=w2000) -> (VISA resource name out=w1997:refnum<visa-resource-name>, error out=w1999:errorcluster)  [unwired: 1 in]
              }
            }
            n703 = call "Display Message to User2"("error in (no error)"=w1964) -> ("error out"=w1963:errorcluster, "Yes"=w1962:bool)  [unwired: 9 in]
            n704 = case shown="True" w1962 {
              tunnel: w1963 -> [w1983 w1987]
              tunnel: [w1983 w1986] -> w1961
              frame False {
              }
              frame True {
                n705 = property on="Status" class="Bool (strict)"() -> ("Value"=w1985:bool)  [unwired: 2 in, 2 out]
                n706 = property on="VISA Marvin" class="VISAName"() -> ("Value"=w1984:refnum<visa-resource-name>)  [unwired: 2 in, 2 out]
                n707 = case shown="True" w1985 {
                  selector: w1985 -> [_ w1991]
                  tunnel: w1987 -> [w1989 w1994]
                  tunnel: w1984 -> [_ w1993]
                  tunnel: [w1988 w1992] -> w1986
                  frame False {
                    n708 = call "Display Message to User3"("error in (no error)"=w1989) -> ("error out"=w1988:errorcluster)  [unwired: 9 in, 1 out]
                  }
                  frame True {
                    n709 = property on="UUT" class="DigNum (strict)"() -> ("Value"=w1990:u8)  [unwired: 2 in, 2 out]
                    n710 = call "SetParam.vi"("RS"=w1991, "error in (no error)"=w1994, "Param to Set in"=w1990, "Visa"=w1993) -> ("error out"=w1992:errorcluster)  [unwired: 7 in]
                  }
                }
              }
            }
          }
          event "Refresh Button": Value Change {
            n711 = event-data() -> ()  [unwired: 1 in, 6 out]
            n712 = property on="Refresh Button" class="Bool (strict)"("Value"=FALSE ("Refresh Button")) -> ()  [unwired: 2 in, 2 out]
            n713 = Two Button Dialog(message="Do you want to erase ATR table?", 1:"No" ("F button name (\"Cancel\")"), 2:"Yes" ("T button name (\"OK\")")) -> (T button?=w2007:bool)
            n714 = case shown="False" w2007 {
              tunnel: [T10."Initialize" T10."Erase ATR Table"] -> w2006
              frame False {
              }
              frame True {
              }
            }
          }
          event "Settings": Value Change {
            n715 = event-data() -> ()  [unwired: 1 in, 6 out]
            n716 = call "Settings"("error in (no error)"=w2024) -> ("Password"=w2023:string, "error out"=w2021:errorcluster)  [unwired: 16 in, 1 out]
            n717 = Equal?(x=w2023, y="123") -> (x = y?=w2019:bool)
            n718 = case shown="True" w2019 {
              tunnel: w2021 -> [w2025 w2032]
              tunnel: [w2025 w2030] -> w2020
              frame False {
                n719 = One Button Dialog(message="Wrong Password!") -> ()  [unwired: 1 in, 1 out]
              }
              frame True {
                n720 = vi-ref "Write Configuration (INI) File.vi"() -> (w2029:refnum<vi>)
                n721 = invoke class="VI" method="FP.Open"(reference=w2029, error in=w2032, "Activate"=TRUE ("Activate?"), "State"=T22."Standard") -> (error out=w2031:errorcluster)  [unwired: 1 in, 4 out]
                n722 = call "Write Configuration (INI) File.vi"("error in"=w2031) -> ("error out"=w2030:errorcluster)  [unwired: 10 in]
              }
            }
          }
        }
      }
      frame "Initialize" {
        w2044 = refnum<visa-resource-name> "COM1" ("VISA resource name")
        w2033 = FALSE ("Visible")
        n723 = disable-structure shown="Disabled" {
          frame Disabled {
            n724 = local write "UUT"("" ("UUT")) -> ()
          }
          frame Enabled {
          }
        }
        n725 = property on="Serial Com" class="Bool"(error in=errorcluster {"status"=FALSE, "code"=0, "source"=""} ("error out"), "Visible"=TRUE) -> (error out=w2048:errorcluster)  [unwired: 1 in, 1 out]
        n726 = property on="VISA Marvin" class="VISAName"(error in=w2048, "Visible"=w2033, "Value"=w2044) -> (error out=w2035:errorcluster)  [unwired: 1 in, 1 out]
        n727 = property on="Stop Burn-in" class="Bool (strict)"(error in=w2035, "Visible"=w2033) -> (error out=w2034:errorcluster)  [unwired: 1 in, 1 out]
        n728 = flat-sequence {
          tunnel: w2034 -> [w2052]
          tunnel: [w2051] -> w2042
          tunnel: [w2054] -> w2041
          tunnel: w2042 -> [w2054]
          tunnel: [w2067] -> w2040
          tunnel: w2041 -> [w2068]
          tunnel: [w2068] -> w2039
          frame #0 {
            n729 = control-ref of="This VI"() -> (w2053:refnum<vi>)
            n730 = invoke class="VI" method="Default Vals.Reinit All"(reference=w2053, error in=w2052) -> (error out=w2051:errorcluster)  [unwired: 1 in, 2 out]
          }
          frame #1 {
            w2058 = u32 4294967295  # AccMask
            w2057 = T4 0 items=["使用Flash参数", "使用界面设置参数"] ("InitFlag")
            w2055 = T6 0 items=["normal operation", "Listen-only mode", "test mode"]  # Mode
            w2056 = T5 3 items=["接收所有类型"=1, "只接收标准帧"=2, "只接收扩展帧"=3] ("Fliter")
            w2062 = u8 10 items=["5k bps"=1, "10k bps"=2, "20k bps"=3, "40k bps"=4, "50k bps"=5, "80k bps"=6, "100k bps"=7, "125k bps"=8, "200k bps"=9, "250k bps"=10, "400k bps"=11, "500k bps"=12, "666k bps"=13, "800k bps"=14, "1000k bps"=15, "33.33k bps"=16, "66.66k bps"=17, "83.33k bps"=18]  # kBaudRate
            w2059 = u32 0  # AccCode
            w2060 = T2 4 items=["USB-CAN"=3, "USB-CAN2"=4] ("DevType")
            w2061 = T7 {"DevType"=3, "DevIndex"=0, "CanIndex"=0, "VCI_INIT_CONFIG"={"AccCode"=0, "AccMask"=0, "InitFlag"=1, "Fliter"=7, "Timing0"=0, "Timing1"=0, "Mode"=0}}  # Config
            # "CANalystII"
            n731 = call "Demo_GetT0T1.vi"("kBaudRate"=w2062) -> ("Timing0"=w2064:u8, "Timing1"=w2065:u8)
            n732 = Bundle By Name(cluster=w2061, "DevType"=w2060, "CanIndex"="Channel 2", "VCI_INIT_CONFIG.AccCode"=w2059, "VCI_INIT_CONFIG.AccMask"=w2058, "VCI_INIT_CONFIG.InitFlag"=w2057, "VCI_INIT_CONFIG.Fliter"=w2056, "VCI_INIT_CONFIG.Timing0"=w2064, "VCI_INIT_CONFIG.Timing1"=w2065, "VCI_INIT_CONFIG.Mode"=w2055) -> (→"Config_CANAT":T7)
          }
          frame #2 {
            w2069 = u16 284 items=["1M"=20, "500K"=28, "250K"=284, "125K"=796, "100K"=17199, "50K"=18223, "20K"=21295, "10K"=26415, "5K"=32639] ("baud in")
            n733 = control-ref of="Config_CANAT"() -> (w2067:refnum<vi>)
            n734 = call "InitCAN_ATII.vi"("Config"=w2067) -> ("Sts"=→"CAN Status":bool)
            n735 = call "ChangeCANBaud.vi"("baud in"=w2069, "reference"=w2067) -> ()
          }
        }
        n736 = Wait (ms)(milliseconds to wait=u32 500) -> ()  [unwired: 1 out]
        "Status" <- FALSE ("Serial Status")
      }
    }
    "Pannel User Message" <- w1578
  }
  n737 = disable-structure shown="Disabled" {
    frame Disabled {
      (unwired) "7.5.2 Enable test in process..." ("Strin")
      n738 = control-ref of="Stop Button"() -> (w2079:refnum<vi>)
      n739 = control-ref of="Pannel User Message"() -> (w2077:refnum<vi>)
      n740 = control-ref of="ATR"() -> (w2078:refnum<vi>)
      n741 = control-ref of="Config_CANAT"() -> (w2076:refnum<vi>)
      n742 = control-ref of="Motor Speed RPM"() -> (w2075:refnum<vi>)
      n743 = control-ref of="UUT"() -> (w2074:refnum<vi>)
      n744 = control-ref of="Stop Burn-in"() -> (w2073:refnum<vi>)
      n745 = property class="Bool (strict)"() -> ("Value"=w2072:bool)  [unwired: 2 in, 2 out]
      n746 = Select(s=w2072) -> ()  [unwired: 2 in, 1 out]
    }
    frame Enabled {
    }
  }
  n747 = disable-structure shown="Disabled" {
    frame Disabled {
      (unwired) 0.02003173828125 ("x")
      n748 = control-ref of="Stop Burn-in"() -> ()  [unwired: 1 out]
      n749 = call "GetADCTester (SubVI).vi"() -> ()  [unwired: 9 in, 3 out]
      n750 = control-ref of="Motor Speed RPM"() -> ()  [unwired: 1 out]
      n751 = control-ref of="Stop Button"() -> ()  [unwired: 1 out]
      n752 = control-ref of="Config_CANAT"() -> ()  [unwired: 1 out]
      n753 = call "CANSendMotorSpeed.vi"() -> ()  [unwired: 11 in, 1 out]
      n754 = call "TesterOption (SubVI).vi"() -> ()  [unwired: 10 in, 2 out]
      n755 = call "Find_Number_LineMARVIN.vi"() -> ()  [unwired: 5 in, 4 out]
      n756 = property on="UUT" class="DigNum (strict)" props=["Value"]() -> ()  [unwired: 2 in, 3 out]
      n757 = control-ref of="UUT"() -> ()  [unwired: 1 out]
      n758 = call "DegToDAC (SubVI).vi"() -> ()  [unwired: 10 in, 2 out]
      n759 = call "Write panel message (SubVI).vi"() -> ()  [unwired: 11 in, 1 out]
      n760 = control-ref of="ATR"() -> ()  [unwired: 1 out]
      n761 = property on="VISA Tester" class="VISAName" props=["Value"]() -> ()  [unwired: 2 in, 3 out]
      n762 = call "TesterOption (SubVI).vi"() -> ()  [unwired: 10 in, 2 out]
      n763 = call "PassOrFail (SubVI).vi"() -> ()  [unwired: 11 in, 1 out]
    }
    frame Enabled {
    }
  }
  n764 = disable-structure shown="Disabled" {
    frame Disabled {
      n765 = flat-sequence {
        frame #0 {
          n766 = call "CANSendMotorSpeed.vi"("Remote"=TRUE, "Motor Speed RPM"=u16 0) -> ("error out"=w2081:errorcluster, "UUT"=w2084:refnum<vi>)  [unwired: 8 in]
          n767 = property on="VISA Tester" class="VISAName"() -> ("Value"=w2080:refnum<visa-resource-name>)  [unwired: 2 in, 2 out]
          n768 = call "TesterOption (SubVI).vi"("error in (no error)"=w2081, "On/Off"=FALSE, "Tester Option"=T11."Power", "VISA Refnum in"=w2080) -> ()  [unwired: 6 in, 2 out]
        }
      }
    }
    frame Enabled {
    }
  }
